vi "Autonomous Independent.vi"() -> ()   [LabVIEW 2017]
doc: "This VI is called when autonomous begins, and will automatically be terminated when autonomous ends. You can carry out timed or sensor driven robot movement independently without needing to return to the caller."
uses:
  <vilib>/Rock Robotics/WPI/Utilities/WPI_GetSetVariantRefNum.vi
  <vilib>/Rock Robotics/Network Tables/NT Read String.vi
  <vilib>/Rock Robotics/Network Tables/NT Write Numeric Array.vi
  Robot Global Data.vi
  <vilib>/Rock Robotics/WPI/Solenoid/Deprecated/WPI_SolenoidSetBool.vi
panel:
  in  "Right LLL":T1(array[cluster])=[{"Left Joystick"=0.975, "Right Joystick"=1.0, "Duration"=5.0, "SOL A"=TRUE, "SOL B"=FALSE, "Lift Up"=FALSE, "Lift Down"=FALSE, "Intake In"=FALSE, "Intake Out"=FALSE, "Left Distance"=10.0, "Right Distance"=10.0, "Drive?"=TRUE, "Wrist Up"=FALSE, "Wrist Down"=FALSE, "Lift Target"=0.0, "Wrist Target"=0.0}, {"Left Joystick"=0.0, "Right Joystick"=0.0, "Duration"=0.5, "SOL A"=TRUE, "SOL B"=FALSE, "Lift Up"=FALSE, "Lift Down"=FALSE, "Intake In"=FALSE, "Intake Out"=FALSE, "Left Distance"=0.0, "Right Distance"=0.0, "Drive?"=FALSE, "Wrist Up"=FALSE, "Wrist Down"=FALSE, "Lift Target"=0.0, "Wrist Target"=0.0}, {"Left Joystick"=0.975, "Right Joystick"=-1.0, "Duration"=5.0, "SOL A"=FALSE, "SOL B"=TRUE, "Lift Up"=FALSE, "Lift Down"=FALSE, "Intake In"=FALSE, "Intake Out"=FALSE, "Left Distance"=24.2, "Right Distance"=24.2, "Drive?"=TRUE, "Wrist Up"=FALSE, "Wrist Down"=FALSE, "Lift Target"=0.0, "Wrist Target"=0.0}, {"Left Joystick"=0.0, "Right Joystick"=0.0, "Duration"=0.5, "SOL A"=TRUE, "SOL B"=FALSE, "Lift Up"=FALSE, "Lift Down"=FALSE, "Intake In"=FALSE, "Intake Out"=FALSE, "Left Distance"=0.0, "Right Distance"=0.0, "Drive?"=FALSE, "Wrist Up"=FALSE, "Wrist Down"=FALSE, "Lift Target"=0.0, "Wrist Target"=0.0}, {"Left Joystick"=0.975, "Right Joystick"=1.0, "Duration"=5.0, "SOL A"=TRUE, "SOL B"=FALSE, "Lift Up"=FALSE, "Lift Down"=FALSE, "Intake In"=FALSE, "Intake Out"=FALSE, "Left Distance"=192.0, "Right Distance"=192.0, "Drive?"=TRUE, "Wrist Up"=FALSE, "Wrist Down"=FALSE, "Lift Target"=0.0, "Wrist Target"=0.0}, {"Left Joystick"=0.0, "Right Joystick"=0.0, "Duration"=0.5, "SOL A"=TRUE, "SOL B"=FALSE, "Lift Up"=FALSE, "Lift Down"=FALSE, "Intake In"=FALSE, "Intake Out"=FALSE, "Left Distance"=0.0, "Right Distance"=0.0, "Drive?"=FALSE, "Wrist Up"=FALSE, "Wrist Down"=FALSE, "Lift Target"=0.0, "Wrist Target"=0.0}, {"Left Joystick"=-0.975, "Right Joystick"=-1.0, "Duration"=5.0, "SOL A"=FALSE, "SOL B"=TRUE, "Lift Up"=FALSE, "Lift Down"=FALSE, "Intake In"=FALSE, "Intake Out"=FALSE, "Left Distance"=24.2, "Right Distance"=24.2, "Drive?"=TRUE, "Wrist Up"=FALSE, "Wrist Down"=FALSE, "Lift Target"=0.0, "Wrist Target"=0.0}, {"Left Joystick"=0.0, "Right Joystick"=0.0, "Duration"=0.5, "SOL A"=TRUE, "SOL B"=FALSE, "Lift Up"=FALSE, "Lift Down"=FALSE, "Intake In"=FALSE, "Intake Out"=FALSE, "Left Distance"=0.0, "Right Distance"=0.0, "Drive?"=FALSE, "Wrist Up"=FALSE, "Wrist Down"=FALSE, "Lift Target"=0.0, "Wrist Target"=0.0}, {"Left Joystick"=0.975, "Right Joystick"=1.0, "Duration"=5.0, "SOL A"=TRUE, "SOL B"=FALSE, "Lift Up"=FALSE, "Lift Down"=FALSE, "Intake In"=FALSE, "Intake Out"=FALSE, "Left Distance"=152.0, "Right Distance"=152.0, "Drive?"=TRUE, "Wrist Up"=FALSE, "Wrist Down"=FALSE, "Lift Target"=0.0, "Wrist Target"=0.0}, {"Left Joystick"=0.0, "Right Joystick"=0.0, "Duration"=0.5, "SOL A"=TRUE, "SOL B"=FALSE, "Lift Up"=FALSE, "Lift Down"=FALSE, "Intake In"=FALSE, "Intake Out"=FALSE, "Left Distance"=0.0, "Right Distance"=0.0, "Drive?"=FALSE, "Wrist Up"=FALSE, "Wrist Down"=FALSE, "Lift Target"=0.0, "Wrist Target"=0.0}, {"Left Joystick"=0.975, "Right Joystick"=-1.0, "Duration"=5.0, "SOL A"=FALSE, "SOL B"=TRUE, "Lift Up"=TRUE, "Lift Down"=FALSE, "Intake In"=FALSE, "Intake Out"=FALSE, "Left Distance"=12.1, "Right Distance"=12.1, "Drive?"=TRUE, "Wrist Up"=TRUE, "Wrist Down"=FALSE, "Lift Target"=15.0, "Wrist Target"=45.0}, {"Left Joystick"=0.0, "Right Joystick"=0.0, "Duration"=0.75, "SOL A"=TRUE, "SOL B"=FALSE, "Lift Up"=FALSE, "Lift Down"=FALSE, "Intake In"=FALSE, "Intake Out"=TRUE, "Left Distance"=0.0, "Right Distance"=0.0, "Drive?"=FALSE, "Wrist Up"=FALSE, "Wrist Down"=FALSE, "Lift Target"=0.0, "Wrist Target"=0.0}, {"Left Joystick"=0.0, "Right Joystick"=0.0, "Duration"=3.0, "SOL A"=TRUE, "SOL B"=FALSE, "Lift Up"=FALSE, "Lift Down"=FALSE, "Intake In"=FALSE, "Intake Out"=FALSE, "Left Distance"=25.0, "Right Distance"=25.0, "Drive?"=TRUE, "Wrist Up"=FALSE, "Wrist Down"=FALSE, "Lift Target"=0.0, "Wrist Target"=0.0}, {"Left Joystick"=0.0, "Right Joystick"=0.0, "Duration"=0.75, "SOL A"=TRUE, "SOL B"=FALSE, "Lift Up"=FALSE, "Lift Down"=FALSE, "Intake In"=TRUE, "Intake Out"=FALSE, "Left Distance"=0.0, "Right Distance"=0.0, "Drive?"=TRUE, "Wrist Up"=FALSE, "Wrist Down"=FALSE, "Lift Target"=0.0, "Wrist Target"=0.0}]
  in  "Right LRL":T1(array[cluster])=[{"Left Joystick"=0.975, "Right Joystick"=1.0, "Duration"=5.0, "SOL A"=TRUE, "SOL B"=FALSE, "Lift Up"=FALSE, "Lift Down"=FALSE, "Intake In"=FALSE, "Intake Out"=FALSE, "Left Distance"=10.0, "Right Distance"=10.0, "Drive?"=TRUE, "Wrist Up"=FALSE, "Wrist Down"=FALSE, "Lift Target"=0.0, "Wrist Target"=0.0}, {"Left Joystick"=0.0, "Right Joystick"=0.0, "Duration"=0.5, "SOL A"=TRUE, "SOL B"=FALSE, "Lift Up"=FALSE, "Lift Down"=FALSE, "Intake In"=FALSE, "Intake Out"=FALSE, "Left Distance"=0.0, "Right Distance"=0.0, "Drive?"=FALSE, "Wrist Up"=FALSE, "Wrist Down"=FALSE, "Lift Target"=0.0, "Wrist Target"=0.0}, {"Left Joystick"=0.975, "Right Joystick"=-1.0, "Duration"=5.0, "SOL A"=FALSE, "SOL B"=TRUE, "Lift Up"=FALSE, "Lift Down"=FALSE, "Intake In"=FALSE, "Intake Out"=FALSE, "Left Distance"=24.2, "Right Distance"=24.2, "Drive?"=TRUE, "Wrist Up"=FALSE, "Wrist Down"=FALSE, "Lift Target"=0.0, "Wrist Target"=0.0}, {"Left Joystick"=0.0, "Right Joystick"=0.0, "Duration"=0.5, "SOL A"=TRUE, "SOL B"=FALSE, "Lift Up"=FALSE, "Lift Down"=FALSE, "Intake In"=FALSE, "Intake Out"=FALSE, "Left Distance"=0.0, "Right Distance"=0.0, "Drive?"=FALSE, "Wrist Up"=FALSE, "Wrist Down"=FALSE, "Lift Target"=0.0, "Wrist Target"=0.0}, {"Left Joystick"=0.975, "Right Joystick"=1.0, "Duration"=5.0, "SOL A"=TRUE, "SOL B"=FALSE, "Lift Up"=FALSE, "Lift Down"=FALSE, "Intake In"=FALSE, "Intake Out"=FALSE, "Left Distance"=192.0, "Right Distance"=192.0, "Drive?"=TRUE, "Wrist Up"=FALSE, "Wrist Down"=FALSE, "Lift Target"=0.0, "Wrist Target"=0.0}, {"Left Joystick"=0.0, "Right Joystick"=0.0, "Duration"=0.5, "SOL A"=TRUE, "SOL B"=FALSE, "Lift Up"=FALSE, "Lift Down"=FALSE, "Intake In"=FALSE, "Intake Out"=FALSE, "Left Distance"=0.0, "Right Distance"=0.0, "Drive?"=FALSE, "Wrist Up"=FALSE, "Wrist Down"=FALSE, "Lift Target"=0.0, "Wrist Target"=0.0}, {"Left Joystick"=-0.975, "Right Joystick"=-1.0, "Duration"=5.0, "SOL A"=FALSE, "SOL B"=TRUE, "Lift Up"=FALSE, "Lift Down"=FALSE, "Intake In"=FALSE, "Intake Out"=FALSE, "Left Distance"=24.2, "Right Distance"=24.2, "Drive?"=TRUE, "Wrist Up"=FALSE, "Wrist Down"=FALSE, "Lift Target"=0.0, "Wrist Target"=0.0}, {"Left Joystick"=0.0, "Right Joystick"=0.0, "Duration"=0.5, "SOL A"=TRUE, "SOL B"=FALSE, "Lift Up"=FALSE, "Lift Down"=FALSE, "Intake In"=FALSE, "Intake Out"=FALSE, "Left Distance"=0.0, "Right Distance"=0.0, "Drive?"=FALSE, "Wrist Up"=FALSE, "Wrist Down"=FALSE, "Lift Target"=0.0, "Wrist Target"=0.0}, {"Left Joystick"=0.975, "Right Joystick"=1.0, "Duration"=5.0, "SOL A"=TRUE, "SOL B"=FALSE, "Lift Up"=FALSE, "Lift Down"=FALSE, "Intake In"=FALSE, "Intake Out"=FALSE, "Left Distance"=152.0, "Right Distance"=152.0, "Drive?"=TRUE, "Wrist Up"=FALSE, "Wrist Down"=FALSE, "Lift Target"=0.0, "Wrist Target"=0.0}, {"Left Joystick"=0.0, "Right Joystick"=0.0, "Duration"=0.5, "SOL A"=TRUE, "SOL B"=FALSE, "Lift Up"=FALSE, "Lift Down"=FALSE, "Intake In"=FALSE, "Intake Out"=FALSE, "Left Distance"=0.0, "Right Distance"=0.0, "Drive?"=FALSE, "Wrist Up"=FALSE, "Wrist Down"=FALSE, "Lift Target"=0.0, "Wrist Target"=0.0}, {"Left Joystick"=0.975, "Right Joystick"=-1.0, "Duration"=5.0, "SOL A"=FALSE, "SOL B"=TRUE, "Lift Up"=TRUE, "Lift Down"=FALSE, "Intake In"=FALSE, "Intake Out"=FALSE, "Left Distance"=12.1, "Right Distance"=12.1, "Drive?"=TRUE, "Wrist Up"=TRUE, "Wrist Down"=FALSE, "Lift Target"=15.0, "Wrist Target"=45.0}, {"Left Joystick"=0.0, "Right Joystick"=0.0, "Duration"=0.75, "SOL A"=TRUE, "SOL B"=FALSE, "Lift Up"=FALSE, "Lift Down"=FALSE, "Intake In"=FALSE, "Intake Out"=TRUE, "Left Distance"=0.0, "Right Distance"=0.0, "Drive?"=FALSE, "Wrist Up"=FALSE, "Wrist Down"=FALSE, "Lift Target"=0.0, "Wrist Target"=0.0}, {"Left Joystick"=0.0, "Right Joystick"=0.0, "Duration"=3.0, "SOL A"=TRUE, "SOL B"=FALSE, "Lift Up"=FALSE, "Lift Down"=FALSE, "Intake In"=FALSE, "Intake Out"=FALSE, "Left Distance"=25.0, "Right Distance"=25.0, "Drive?"=TRUE, "Wrist Up"=FALSE, "Wrist Down"=FALSE, "Lift Target"=0.0, "Wrist Target"=0.0}, {"Left Joystick"=0.0, "Right Joystick"=0.0, "Duration"=0.75, "SOL A"=TRUE, "SOL B"=FALSE, "Lift Up"=FALSE, "Lift Down"=FALSE, "Intake In"=TRUE, "Intake Out"=FALSE, "Left Distance"=0.0, "Right Distance"=0.0, "Drive?"=TRUE, "Wrist Up"=FALSE, "Wrist Down"=FALSE, "Lift Target"=0.0, "Wrist Target"=0.0}, {"Left Joystick"=0.0, "Right Joystick"=0.0, "Duration"=0.5, "SOL A"=TRUE, "SOL B"=FALSE, "Lift Up"=FALSE, "Lift Down"=FALSE, "Intake In"=FALSE, "Intake Out"=FALSE, "Left Distance"=0.0, "Right Distance"=0.0, "Drive?"=FALSE, "Wrist Up"=FALSE, "Wrist Down"=FALSE, "Lift Target"=0.0, "Wrist Target"=0.0}, {"Left Joystick"=0.975, "Right Joystick"=1.0, "Duration"=5.0, "SOL A"=TRUE, "SOL B"=FALSE, "Lift Up"=FALSE, "Lift Down"=FALSE, "Intake In"=FALSE, "Intake Out"=FALSE, "Left Distance"=12.0, "Right Distance"=12.0, "Drive?"=TRUE, "Wrist Up"=FALSE, "Wrist Down"=FALSE, "Lift Target"=0.0, "Wrist Target"=0.0}, {"Left Joystick"=0.0, "Right Joystick"=0.0, "Duration"=0.5, "SOL A"=TRUE, "SOL B"=FALSE, "Lift Up"=FALSE, "Lift Down"=FALSE, "Intake In"=FALSE, "Intake Out"=FALSE, "Left Distance"=0.0, "Right Distance"=0.0, "Drive?"=FALSE, "Wrist Up"=FALSE, "Wrist Down"=FALSE, "Lift Target"=0.0, "Wrist Target"=0.0}, {"Left Joystick"=0.975, "Right Joystick"=-1.0, "Duration"=5.0, "SOL A"=FALSE, "SOL B"=TRUE, "Lift Up"=FALSE, "Lift Down"=FALSE, "Intake In"=FALSE, "Intake Out"=FALSE, "Left Distance"=12.1, "Right Distance"=12.1, "Drive?"=TRUE, "Wrist Up"=FALSE, "Wrist Down"=FALSE, "Lift Target"=0.0, "Wrist Target"=0.0}, {"Left Joystick"=0.0, "Right Joystick"=0.0, "Duration"=0.5, "SOL A"=TRUE, "SOL B"=FALSE, "Lift Up"=FALSE, "Lift Down"=FALSE, "Intake In"=FALSE, "Intake Out"=FALSE, "Left Distance"=0.0, "Right Distance"=0.0, "Drive?"=FALSE, "Wrist Up"=FALSE, "Wrist Down"=FALSE, "Lift Target"=0.0, "Wrist Target"=0.0}, {"Left Joystick"=-0.975, "Right Joystick"=-1.0, "Duration"=5.0, "SOL A"=TRUE, "SOL B"=FALSE, "Lift Up"=FALSE, "Lift Down"=FALSE, "Intake In"=FALSE, "Intake Out"=FALSE, "Left Distance"=156.0, "Right Distance"=156.0, "Drive?"=TRUE, "Wrist Up"=FALSE, "Wrist Down"=FALSE, "Lift Target"=0.0, "Wrist Target"=0.0}, {"Left Joystick"=0.0, "Right Joystick"=0.0, "Duration"=0.5, "SOL A"=TRUE, "SOL B"=FALSE, "Lift Up"=FALSE, "Lift Down"=FALSE, "Intake In"=FALSE, "Intake Out"=FALSE, "Left Distance"=0.0, "Right Distance"=0.0, "Drive?"=FALSE, "Wrist Up"=FALSE, "Wrist Down"=FALSE, "Lift Target"=0.0, "Wrist Target"=0.0}, {"Left Joystick"=0.975, "Right Joystick"=-1.0, "Duration"=5.0, "SOL A"=FALSE, "SOL B"=TRUE, "Lift Up"=FALSE, "Lift Down"=FALSE, "Intake In"=FALSE, "Intake Out"=FALSE, "Left Distance"=24.2, "Right Distance"=24.2, "Drive?"=TRUE, "Wrist Up"=FALSE, "Wrist Down"=FALSE, "Lift Target"=0.0, "Wrist Target"=0.0}, {"Left Joystick"=0.0, "Right Joystick"=0.0, "Duration"=0.5, "SOL A"=TRUE, "SOL B"=FALSE, "Lift Up"=FALSE, "Lift Down"=FALSE, "Intake In"=FALSE, "Intake Out"=FALSE, "Left Distance"=0.0, "Right Distance"=0.0, "Drive?"=FALSE, "Wrist Up"=FALSE, "Wrist Down"=FALSE, "Lift Target"=0.0, "Wrist Target"=0.0}, {"Left Joystick"=-0.975, "Right Joystick"=-1.0, "Duration"=5.0, "SOL A"=TRUE, "SOL B"=FALSE, "Lift Up"=FALSE, "Lift Down"=FALSE, "Intake In"=FALSE, "Intake Out"=FALSE, "Left Distance"=48.0, "Right Distance"=48.0, "Drive?"=TRUE, "Wrist Up"=FALSE, "Wrist Down"=FALSE, "Lift Target"=0.0, "Wrist Target"=0.0}, {"Left Joystick"=0.0, "Right Joystick"=0.0, "Duration"=0.5, "SOL A"=TRUE, "SOL B"=FALSE, "Lift Up"=FALSE, "Lift Down"=FALSE, "Intake In"=FALSE, "Intake Out"=FALSE, "Left Distance"=0.0, "Right Distance"=0.0, "Drive?"=FALSE, "Wrist Up"=FALSE, "Wrist Down"=FALSE, "Lift Target"=0.0, "Wrist Target"=0.0}, {"Left Joystick"=0.975, "Right Joystick"=-1.0, "Duration"=5.0, "SOL A"=FALSE, "SOL B"=TRUE, "Lift Up"=TRUE, "Lift Down"=FALSE, "Intake In"=FALSE, "Intake Out"=FALSE, "Left Distance"=6.05, "Right Distance"=6.05, "Drive?"=TRUE, "Wrist Up"=TRUE, "Wrist Down"=FALSE, "Lift Target"=50.0, "Wrist Target"=45.0}, {"Left Joystick"=0.0, "Right Joystick"=0.0, "Duration"=0.75, "SOL A"=TRUE, "SOL B"=FALSE, "Lift Up"=FALSE, "Lift Down"=FALSE, "Intake In"=FALSE, "Intake Out"=TRUE, "Left Distance"=0.0, "Right Distance"=0.0, "Drive?"=FALSE, "Wrist Up"=FALSE, "Wrist Down"=FALSE, "Lift Target"=0.0, "Wrist Target"=0.0}]
  in  "Left RLR":T1(array[cluster])=[{"Left Joystick"=0.975, "Right Joystick"=1.0, "Duration"=5.0, "SOL A"=TRUE, "SOL B"=FALSE, "Lift Up"=FALSE, "Lift Down"=FALSE, "Intake In"=FALSE, "Intake Out"=FALSE, "Left Distance"=10.0, "Right Distance"=10.0, "Drive?"=TRUE, "Wrist Up"=FALSE, "Wrist Down"=FALSE, "Lift Target"=0.0, "Wrist Target"=0.0}, {"Left Joystick"=0.0, "Right Joystick"=0.0, "Duration"=0.5, "SOL A"=TRUE, "SOL B"=FALSE, "Lift Up"=FALSE, "Lift Down"=FALSE, "Intake In"=FALSE, "Intake Out"=FALSE, "Left Distance"=0.0, "Right Distance"=0.0, "Drive?"=FALSE, "Wrist Up"=FALSE, "Wrist Down"=FALSE, "Lift Target"=0.0, "Wrist Target"=0.0}, {"Left Joystick"=-0.975, "Right Joystick"=1.0, "Duration"=5.0, "SOL A"=FALSE, "SOL B"=TRUE, "Lift Up"=FALSE, "Lift Down"=FALSE, "Intake In"=FALSE, "Intake Out"=FALSE, "Left Distance"=24.2, "Right Distance"=24.2, "Drive?"=TRUE, "Wrist Up"=FALSE, "Wrist Down"=FALSE, "Lift Target"=0.0, "Wrist Target"=0.0}, {"Left Joystick"=0.0, "Right Joystick"=0.0, "Duration"=0.5, "SOL A"=TRUE, "SOL B"=FALSE, "Lift Up"=FALSE, "Lift Down"=FALSE, "Intake In"=FALSE, "Intake Out"=FALSE, "Left Distance"=0.0, "Right Distance"=0.0, "Drive?"=FALSE, "Wrist Up"=FALSE, "Wrist Down"=FALSE, "Lift Target"=0.0, "Wrist Target"=0.0}, {"Left Joystick"=0.975, "Right Joystick"=1.0, "Duration"=5.0, "SOL A"=TRUE, "SOL B"=FALSE, "Lift Up"=FALSE, "Lift Down"=FALSE, "Intake In"=FALSE, "Intake Out"=FALSE, "Left Distance"=192.0, "Right Distance"=192.0, "Drive?"=TRUE, "Wrist Up"=FALSE, "Wrist Down"=FALSE, "Lift Target"=0.0, "Wrist Target"=0.0}, {"Left Joystick"=0.0, "Right Joystick"=0.0, "Duration"=0.5, "SOL A"=TRUE, "SOL B"=FALSE, "Lift Up"=FALSE, "Lift Down"=FALSE, "Intake In"=FALSE, "Intake Out"=FALSE, "Left Distance"=0.0, "Right Distance"=0.0, "Drive?"=FALSE, "Wrist Up"=FALSE, "Wrist Down"=FALSE, "Lift Target"=0.0, "Wrist Target"=0.0}, {"Left Joystick"=0.975, "Right Joystick"=-1.0, "Duration"=5.0, "SOL A"=FALSE, "SOL B"=TRUE, "Lift Up"=FALSE, "Lift Down"=FALSE, "Intake In"=FALSE, "Intake Out"=FALSE, "Left Distance"=24.2, "Right Distance"=24.2, "Drive?"=TRUE, "Wrist Up"=FALSE, "Wrist Down"=FALSE, "Lift Target"=0.0, "Wrist Target"=0.0}, {"Left Joystick"=0.0, "Right Joystick"=0.0, "Duration"=0.5, "SOL A"=TRUE, "SOL B"=FALSE, "Lift Up"=FALSE, "Lift Down"=FALSE, "Intake In"=FALSE, "Intake Out"=FALSE, "Left Distance"=0.0, "Right Distance"=0.0, "Drive?"=FALSE, "Wrist Up"=FALSE, "Wrist Down"=FALSE, "Lift Target"=0.0, "Wrist Target"=0.0}, {"Left Joystick"=0.975, "Right Joystick"=1.0, "Duration"=5.0, "SOL A"=TRUE, "SOL B"=FALSE, "Lift Up"=FALSE, "Lift Down"=FALSE, "Intake In"=FALSE, "Intake Out"=FALSE, "Left Distance"=152.0, "Right Distance"=152.0, "Drive?"=TRUE, "Wrist Up"=FALSE, "Wrist Down"=FALSE, "Lift Target"=0.0, "Wrist Target"=0.0}, {"Left Joystick"=0.0, "Right Joystick"=0.0, "Duration"=0.5, "SOL A"=TRUE, "SOL B"=FALSE, "Lift Up"=FALSE, "Lift Down"=FALSE, "Intake In"=FALSE, "Intake Out"=FALSE, "Left Distance"=0.0, "Right Distance"=0.0, "Drive?"=FALSE, "Wrist Up"=FALSE, "Wrist Down"=FALSE, "Lift Target"=0.0, "Wrist Target"=0.0}, {"Left Joystick"=-0.975, "Right Joystick"=1.0, "Duration"=5.0, "SOL A"=FALSE, "SOL B"=TRUE, "Lift Up"=TRUE, "Lift Down"=FALSE, "Intake In"=FALSE, "Intake Out"=FALSE, "Left Distance"=12.1, "Right Distance"=12.1, "Drive?"=TRUE, "Wrist Up"=TRUE, "Wrist Down"=FALSE, "Lift Target"=15.0, "Wrist Target"=45.0}, {"Left Joystick"=0.0, "Right Joystick"=0.0, "Duration"=0.75, "SOL A"=TRUE, "SOL B"=FALSE, "Lift Up"=FALSE, "Lift Down"=FALSE, "Intake In"=FALSE, "Intake Out"=TRUE, "Left Distance"=0.0, "Right Distance"=0.0, "Drive?"=FALSE, "Wrist Up"=FALSE, "Wrist Down"=FALSE, "Lift Target"=0.0, "Wrist Target"=0.0}, {"Left Joystick"=0.0, "Right Joystick"=0.0, "Duration"=3.0, "SOL A"=TRUE, "SOL B"=FALSE, "Lift Up"=FALSE, "Lift Down"=FALSE, "Intake In"=FALSE, "Intake Out"=FALSE, "Left Distance"=25.0, "Right Distance"=25.0, "Drive?"=TRUE, "Wrist Up"=FALSE, "Wrist Down"=FALSE, "Lift Target"=0.0, "Wrist Target"=0.0}, {"Left Joystick"=0.0, "Right Joystick"=0.0, "Duration"=0.75, "SOL A"=TRUE, "SOL B"=FALSE, "Lift Up"=FALSE, "Lift Down"=FALSE, "Intake In"=TRUE, "Intake Out"=FALSE, "Left Distance"=0.0, "Right Distance"=0.0, "Drive?"=TRUE, "Wrist Up"=FALSE, "Wrist Down"=FALSE, "Lift Target"=0.0, "Wrist Target"=0.0}]
  in  "Left RRR":T1(array[cluster])=[{"Left Joystick"=0.975, "Right Joystick"=1.0, "Duration"=5.0, "SOL A"=TRUE, "SOL B"=FALSE, "Lift Up"=FALSE, "Lift Down"=FALSE, "Intake In"=FALSE, "Intake Out"=FALSE, "Left Distance"=10.0, "Right Distance"=10.0, "Drive?"=TRUE, "Wrist Up"=FALSE, "Wrist Down"=FALSE, "Lift Target"=0.0, "Wrist Target"=0.0}, {"Left Joystick"=0.0, "Right Joystick"=0.0, "Duration"=0.5, "SOL A"=TRUE, "SOL B"=FALSE, "Lift Up"=FALSE, "Lift Down"=FALSE, "Intake In"=FALSE, "Intake Out"=FALSE, "Left Distance"=0.0, "Right Distance"=0.0, "Drive?"=FALSE, "Wrist Up"=FALSE, "Wrist Down"=FALSE, "Lift Target"=0.0, "Wrist Target"=0.0}, {"Left Joystick"=-0.975, "Right Joystick"=1.0, "Duration"=5.0, "SOL A"=FALSE, "SOL B"=TRUE, "Lift Up"=FALSE, "Lift Down"=FALSE, "Intake In"=FALSE, "Intake Out"=FALSE, "Left Distance"=24.2, "Right Distance"=24.2, "Drive?"=TRUE, "Wrist Up"=FALSE, "Wrist Down"=FALSE, "Lift Target"=0.0, "Wrist Target"=0.0}, {"Left Joystick"=0.0, "Right Joystick"=0.0, "Duration"=0.5, "SOL A"=TRUE, "SOL B"=FALSE, "Lift Up"=FALSE, "Lift Down"=FALSE, "Intake In"=FALSE, "Intake Out"=FALSE, "Left Distance"=0.0, "Right Distance"=0.0, "Drive?"=FALSE, "Wrist Up"=FALSE, "Wrist Down"=FALSE, "Lift Target"=0.0, "Wrist Target"=0.0}, {"Left Joystick"=0.975, "Right Joystick"=1.0, "Duration"=5.0, "SOL A"=TRUE, "SOL B"=FALSE, "Lift Up"=FALSE, "Lift Down"=FALSE, "Intake In"=FALSE, "Intake Out"=FALSE, "Left Distance"=192.0, "Right Distance"=192.0, "Drive?"=TRUE, "Wrist Up"=FALSE, "Wrist Down"=FALSE, "Lift Target"=0.0, "Wrist Target"=0.0}, {"Left Joystick"=0.0, "Right Joystick"=0.0, "Duration"=0.5, "SOL A"=TRUE, "SOL B"=FALSE, "Lift Up"=FALSE, "Lift Down"=FALSE, "Intake In"=FALSE, "Intake Out"=FALSE, "Left Distance"=0.0, "Right Distance"=0.0, "Drive?"=FALSE, "Wrist Up"=FALSE, "Wrist Down"=FALSE, "Lift Target"=0.0, "Wrist Target"=0.0}, {"Left Joystick"=0.975, "Right Joystick"=-1.0, "Duration"=5.0, "SOL A"=FALSE, "SOL B"=TRUE, "Lift Up"=FALSE, "Lift Down"=FALSE, "Intake In"=FALSE, "Intake Out"=FALSE, "Left Distance"=24.2, "Right Distance"=24.2, "Drive?"=TRUE, "Wrist Up"=FALSE, "Wrist Down"=FALSE, "Lift Target"=0.0, "Wrist Target"=0.0}, {"Left Joystick"=0.0, "Right Joystick"=0.0, "Duration"=0.5, "SOL A"=TRUE, "SOL B"=FALSE, "Lift Up"=FALSE, "Lift Down"=FALSE, "Intake In"=FALSE, "Intake Out"=FALSE, "Left Distance"=0.0, "Right Distance"=0.0, "Drive?"=FALSE, "Wrist Up"=FALSE, "Wrist Down"=FALSE, "Lift Target"=0.0, "Wrist Target"=0.0}, {"Left Joystick"=0.975, "Right Joystick"=1.0, "Duration"=5.0, "SOL A"=TRUE, "SOL B"=FALSE, "Lift Up"=FALSE, "Lift Down"=FALSE, "Intake In"=FALSE, "Intake Out"=FALSE, "Left Distance"=152.0, "Right Distance"=152.0, "Drive?"=TRUE, "Wrist Up"=FALSE, "Wrist Down"=FALSE, "Lift Target"=0.0, "Wrist Target"=0.0}, {"Left Joystick"=0.0, "Right Joystick"=0.0, "Duration"=0.5, "SOL A"=TRUE, "SOL B"=FALSE, "Lift Up"=FALSE, "Lift Down"=FALSE, "Intake In"=FALSE, "Intake Out"=FALSE, "Left Distance"=0.0, "Right Distance"=0.0, "Drive?"=FALSE, "Wrist Up"=FALSE, "Wrist Down"=FALSE, "Lift Target"=0.0, "Wrist Target"=0.0}, {"Left Joystick"=-0.975, "Right Joystick"=1.0, "Duration"=5.0, "SOL A"=FALSE, "SOL B"=TRUE, "Lift Up"=TRUE, "Lift Down"=FALSE, "Intake In"=FALSE, "Intake Out"=FALSE, "Left Distance"=12.1, "Right Distance"=12.1, "Drive?"=TRUE, "Wrist Up"=TRUE, "Wrist Down"=FALSE, "Lift Target"=15.0, "Wrist Target"=45.0}, {"Left Joystick"=0.0, "Right Joystick"=0.0, "Duration"=0.75, "SOL A"=TRUE, "SOL B"=FALSE, "Lift Up"=FALSE, "Lift Down"=FALSE, "Intake In"=FALSE, "Intake Out"=TRUE, "Left Distance"=0.0, "Right Distance"=0.0, "Drive?"=FALSE, "Wrist Up"=FALSE, "Wrist Down"=FALSE, "Lift Target"=0.0, "Wrist Target"=0.0}, {"Left Joystick"=0.0, "Right Joystick"=0.0, "Duration"=3.0, "SOL A"=TRUE, "SOL B"=FALSE, "Lift Up"=FALSE, "Lift Down"=FALSE, "Intake In"=FALSE, "Intake Out"=FALSE, "Left Distance"=25.0, "Right Distance"=25.0, "Drive?"=TRUE, "Wrist Up"=FALSE, "Wrist Down"=FALSE, "Lift Target"=0.0, "Wrist Target"=0.0}, {"Left Joystick"=0.0, "Right Joystick"=0.0, "Duration"=0.75, "SOL A"=TRUE, "SOL B"=FALSE, "Lift Up"=FALSE, "Lift Down"=FALSE, "Intake In"=TRUE, "Intake Out"=FALSE, "Left Distance"=0.0, "Right Distance"=0.0, "Drive?"=TRUE, "Wrist Up"=FALSE, "Wrist Down"=FALSE, "Lift Target"=0.0, "Wrist Target"=0.0}]
  in  "Center LRL":T1(array[cluster])=[{"Left Joystick"=-0.975, "Right Joystick"=-1.0, "Duration"=5.0, "SOL A"=TRUE, "SOL B"=FALSE, "Lift Up"=FALSE, "Lift Down"=FALSE, "Intake In"=FALSE, "Intake Out"=FALSE, "Left Distance"=10.0, "Right Distance"=10.0, "Drive?"=TRUE, "Wrist Up"=FALSE, "Wrist Down"=FALSE, "Lift Target"=0.0, "Wrist Target"=0.0}, {"Left Joystick"=0.0, "Right Joystick"=0.0, "Duration"=0.5, "SOL A"=TRUE, "SOL B"=FALSE, "Lift Up"=FALSE, "Lift Down"=FALSE, "Intake In"=FALSE, "Intake Out"=FALSE, "Left Distance"=0.0, "Right Distance"=0.0, "Drive?"=FALSE, "Wrist Up"=FALSE, "Wrist Down"=FALSE, "Lift Target"=0.0, "Wrist Target"=0.0}, {"Left Joystick"=0.975, "Right Joystick"=-1.0, "Duration"=5.0, "SOL A"=FALSE, "SOL B"=TRUE, "Lift Up"=FALSE, "Lift Down"=FALSE, "Intake In"=FALSE, "Intake Out"=FALSE, "Left Distance"=24.2, "Right Distance"=24.2, "Drive?"=TRUE, "Wrist Up"=FALSE, "Wrist Down"=FALSE, "Lift Target"=0.0, "Wrist Target"=0.0}, {"Left Joystick"=0.0, "Right Joystick"=0.0, "Duration"=0.5, "SOL A"=TRUE, "SOL B"=FALSE, "Lift Up"=FALSE, "Lift Down"=FALSE, "Intake In"=FALSE, "Intake Out"=FALSE, "Left Distance"=0.0, "Right Distance"=0.0, "Drive?"=FALSE, "Wrist Up"=FALSE, "Wrist Down"=FALSE, "Lift Target"=0.0, "Wrist Target"=0.0}, {"Left Joystick"=-0.975, "Right Joystick"=-1.0, "Duration"=5.0, "SOL A"=TRUE, "SOL B"=FALSE, "Lift Up"=FALSE, "Lift Down"=FALSE, "Intake In"=FALSE, "Intake Out"=FALSE, "Left Distance"=84.0, "Right Distance"=84.0, "Drive?"=TRUE, "Wrist Up"=FALSE, "Wrist Down"=FALSE, "Lift Target"=0.0, "Wrist Target"=0.0}, {"Left Joystick"=0.0, "Right Joystick"=0.0, "Duration"=0.5, "SOL A"=TRUE, "SOL B"=FALSE, "Lift Up"=FALSE, "Lift Down"=FALSE, "Intake In"=FALSE, "Intake Out"=FALSE, "Left Distance"=0.0, "Right Distance"=0.0, "Drive?"=FALSE, "Wrist Up"=FALSE, "Wrist Down"=FALSE, "Lift Target"=0.0, "Wrist Target"=0.0}, {"Left Joystick"=-0.975, "Right Joystick"=1.0, "Duration"=5.0, "SOL A"=FALSE, "SOL B"=TRUE, "Lift Up"=FALSE, "Lift Down"=FALSE, "Intake In"=FALSE, "Intake Out"=FALSE, "Left Distance"=24.2, "Right Distance"=24.2, "Drive?"=TRUE, "Wrist Up"=FALSE, "Wrist Down"=FALSE, "Lift Target"=0.0, "Wrist Target"=0.0}, {"Left Joystick"=0.0, "Right Joystick"=0.0, "Duration"=0.5, "SOL A"=TRUE, "SOL B"=FALSE, "Lift Up"=FALSE, "Lift Down"=FALSE, "Intake In"=FALSE, "Intake Out"=FALSE, "Left Distance"=0.0, "Right Distance"=0.0, "Drive?"=FALSE, "Wrist Up"=FALSE, "Wrist Down"=FALSE, "Lift Target"=0.0, "Wrist Target"=0.0}, {"Left Joystick"=-0.975, "Right Joystick"=-1.0, "Duration"=5.0, "SOL A"=TRUE, "SOL B"=FALSE, "Lift Up"=FALSE, "Lift Down"=FALSE, "Intake In"=FALSE, "Intake Out"=FALSE, "Left Distance"=152.0, "Right Distance"=152.0, "Drive?"=TRUE, "Wrist Up"=FALSE, "Wrist Down"=FALSE, "Lift Target"=0.0, "Wrist Target"=0.0}, {"Left Joystick"=0.0, "Right Joystick"=0.0, "Duration"=0.5, "SOL A"=TRUE, "SOL B"=FALSE, "Lift Up"=FALSE, "Lift Down"=FALSE, "Intake In"=FALSE, "Intake Out"=FALSE, "Left Distance"=0.0, "Right Distance"=0.0, "Drive?"=FALSE, "Wrist Up"=FALSE, "Wrist Down"=FALSE, "Lift Target"=0.0, "Wrist Target"=0.0}, {"Left Joystick"=-0.975, "Right Joystick"=1.0, "Duration"=5.0, "SOL A"=FALSE, "SOL B"=TRUE, "Lift Up"=TRUE, "Lift Down"=FALSE, "Intake In"=FALSE, "Intake Out"=FALSE, "Left Distance"=36.3, "Right Distance"=36.3, "Drive?"=TRUE, "Wrist Up"=TRUE, "Wrist Down"=FALSE, "Lift Target"=15.0, "Wrist Target"=45.0}, {"Left Joystick"=0.0, "Right Joystick"=0.0, "Duration"=0.75, "SOL A"=TRUE, "SOL B"=FALSE, "Lift Up"=FALSE, "Lift Down"=FALSE, "Intake In"=FALSE, "Intake Out"=TRUE, "Left Distance"=0.0, "Right Distance"=0.0, "Drive?"=FALSE, "Wrist Up"=FALSE, "Wrist Down"=FALSE, "Lift Target"=0.0, "Wrist Target"=0.0}, {"Left Joystick"=0.0, "Right Joystick"=0.0, "Duration"=3.0, "SOL A"=TRUE, "SOL B"=FALSE, "Lift Up"=FALSE, "Lift Down"=FALSE, "Intake In"=FALSE, "Intake Out"=FALSE, "Left Distance"=25.0, "Right Distance"=25.0, "Drive?"=TRUE, "Wrist Up"=FALSE, "Wrist Down"=FALSE, "Lift Target"=0.0, "Wrist Target"=0.0}, {"Left Joystick"=0.0, "Right Joystick"=0.0, "Duration"=0.75, "SOL A"=TRUE, "SOL B"=FALSE, "Lift Up"=FALSE, "Lift Down"=FALSE, "Intake In"=TRUE, "Intake Out"=FALSE, "Left Distance"=0.0, "Right Distance"=0.0, "Drive?"=TRUE, "Wrist Up"=FALSE, "Wrist Down"=FALSE, "Lift Target"=0.0, "Wrist Target"=0.0}]
  in  "Right RRR":T1(array[cluster])=[{"Left Joystick"=0.975, "Right Joystick"=1.0, "Duration"=5.0, "SOL A"=TRUE, "SOL B"=FALSE, "Lift Up"=FALSE, "Lift Down"=FALSE, "Intake In"=FALSE, "Intake Out"=FALSE, "Left Distance"=199.6, "Right Distance"=199.6, "Drive?"=TRUE, "Wrist Up"=FALSE, "Wrist Down"=FALSE, "Lift Target"=0.0, "Wrist Target"=0.0}, {"Left Joystick"=0.0, "Right Joystick"=0.0, "Duration"=0.5, "SOL A"=TRUE, "SOL B"=FALSE, "Lift Up"=FALSE, "Lift Down"=FALSE, "Intake In"=FALSE, "Intake Out"=FALSE, "Left Distance"=0.0, "Right Distance"=0.0, "Drive?"=FALSE, "Wrist Up"=FALSE, "Wrist Down"=FALSE, "Lift Target"=0.0, "Wrist Target"=0.0}, {"Left Joystick"=-0.975, "Right Joystick"=1.0, "Duration"=5.0, "SOL A"=FALSE, "SOL B"=TRUE, "Lift Up"=FALSE, "Lift Down"=FALSE, "Intake In"=FALSE, "Intake Out"=FALSE, "Left Distance"=13.2, "Right Distance"=13.2, "Drive?"=TRUE, "Wrist Up"=FALSE, "Wrist Down"=FALSE, "Lift Target"=0.0, "Wrist Target"=0.0}, {"Left Joystick"=0.0, "Right Joystick"=0.0, "Duration"=0.5, "SOL A"=TRUE, "SOL B"=FALSE, "Lift Up"=FALSE, "Lift Down"=FALSE, "Intake In"=FALSE, "Intake Out"=FALSE, "Left Distance"=0.0, "Right Distance"=0.0, "Drive?"=FALSE, "Wrist Up"=FALSE, "Wrist Down"=FALSE, "Lift Target"=0.0, "Wrist Target"=0.0}, {"Left Joystick"=-0.975, "Right Joystick"=-1.0, "Duration"=5.0, "SOL A"=TRUE, "SOL B"=FALSE, "Lift Up"=TRUE, "Lift Down"=FALSE, "Intake In"=FALSE, "Intake Out"=FALSE, "Left Distance"=18.2, "Right Distance"=18.2, "Drive?"=TRUE, "Wrist Up"=TRUE, "Wrist Down"=FALSE, "Lift Target"=15.0, "Wrist Target"=45.0}, {"Left Joystick"=0.0, "Right Joystick"=0.0, "Duration"=0.75, "SOL A"=TRUE, "SOL B"=FALSE, "Lift Up"=FALSE, "Lift Down"=FALSE, "Intake In"=FALSE, "Intake Out"=TRUE, "Left Distance"=0.0, "Right Distance"=0.0, "Drive?"=FALSE, "Wrist Up"=FALSE, "Wrist Down"=FALSE, "Lift Target"=0.0, "Wrist Target"=0.0}, {"Left Joystick"=0.975, "Right Joystick"=1.0, "Duration"=5.0, "SOL A"=TRUE, "SOL B"=FALSE, "Lift Up"=FALSE, "Lift Down"=FALSE, "Intake In"=FALSE, "Intake Out"=FALSE, "Left Distance"=18.2, "Right Distance"=18.2, "Drive?"=TRUE, "Wrist Up"=FALSE, "Wrist Down"=FALSE, "Lift Target"=0.0, "Wrist Target"=0.0}, {"Left Joystick"=0.0, "Right Joystick"=0.0, "Duration"=0.5, "SOL A"=TRUE, "SOL B"=FALSE, "Lift Up"=FALSE, "Lift Down"=FALSE, "Intake In"=FALSE, "Intake Out"=FALSE, "Left Distance"=0.0, "Right Distance"=0.0, "Drive?"=FALSE, "Wrist Up"=FALSE, "Wrist Down"=FALSE, "Lift Target"=0.0, "Wrist Target"=0.0}, {"Left Joystick"=0.975, "Right Joystick"=-1.0, "Duration"=5.0, "SOL A"=FALSE, "SOL B"=TRUE, "Lift Up"=FALSE, "Lift Down"=FALSE, "Intake In"=FALSE, "Intake Out"=FALSE, "Left Distance"=27.0, "Right Distance"=27.0, "Drive?"=TRUE, "Wrist Up"=FALSE, "Wrist Down"=FALSE, "Lift Target"=0.0, "Wrist Target"=0.0}, {"Left Joystick"=0.0, "Right Joystick"=0.0, "Duration"=0.5, "SOL A"=TRUE, "SOL B"=FALSE, "Lift Up"=FALSE, "Lift Down"=FALSE, "Intake In"=FALSE, "Intake Out"=FALSE, "Left Distance"=0.0, "Right Distance"=0.0, "Drive?"=FALSE, "Wrist Up"=FALSE, "Wrist Down"=FALSE, "Lift Target"=0.0, "Wrist Target"=0.0}, {"Left Joystick"=0.975, "Right Joystick"=1.0, "Duration"=5.0, "SOL A"=TRUE, "SOL B"=FALSE, "Lift Up"=FALSE, "Lift Down"=FALSE, "Intake In"=FALSE, "Intake Out"=FALSE, "Left Distance"=19.7, "Right Distance"=19.7, "Drive?"=TRUE, "Wrist Up"=FALSE, "Wrist Down"=FALSE, "Lift Target"=0.0, "Wrist Target"=0.0}, {"Left Joystick"=0.0, "Right Joystick"=0.0, "Duration"=0.5, "SOL A"=TRUE, "SOL B"=FALSE, "Lift Up"=FALSE, "Lift Down"=FALSE, "Intake In"=FALSE, "Intake Out"=FALSE, "Left Distance"=0.0, "Right Distance"=0.0, "Drive?"=FALSE, "Wrist Up"=FALSE, "Wrist Down"=FALSE, "Lift Target"=0.0, "Wrist Target"=0.0}, {"Left Joystick"=-0.975, "Right Joystick"=1.0, "Duration"=5.0, "SOL A"=FALSE, "SOL B"=TRUE, "Lift Up"=FALSE, "Lift Down"=FALSE, "Intake In"=FALSE, "Intake Out"=FALSE, "Left Distance"=25.6, "Right Distance"=25.6, "Drive?"=TRUE, "Wrist Up"=FALSE, "Wrist Down"=FALSE, "Lift Target"=0.0, "Wrist Target"=0.0}, {"Left Joystick"=0.0, "Right Joystick"=0.0, "Duration"=0.5, "SOL A"=TRUE, "SOL B"=FALSE, "Lift Up"=FALSE, "Lift Down"=FALSE, "Intake In"=FALSE, "Intake Out"=FALSE, "Left Distance"=0.0, "Right Distance"=0.0, "Drive?"=FALSE, "Wrist Up"=FALSE, "Wrist Down"=FALSE, "Lift Target"=0.0, "Wrist Target"=0.0}, {"Left Joystick"=-0.975, "Right Joystick"=-1.0, "Duration"=5.0, "SOL A"=TRUE, "SOL B"=FALSE, "Lift Up"=FALSE, "Lift Down"=FALSE, "Intake In"=FALSE, "Intake Out"=FALSE, "Left Distance"=4.0, "Right Distance"=4.0, "Drive?"=TRUE, "Wrist Up"=FALSE, "Wrist Down"=FALSE, "Lift Target"=0.0, "Wrist Target"=0.0}, {"Left Joystick"=0.0, "Right Joystick"=0.0, "Duration"=0.75, "SOL A"=TRUE, "SOL B"=FALSE, "Lift Up"=FALSE, "Lift Down"=FALSE, "Intake In"=TRUE, "Intake Out"=FALSE, "Left Distance"=0.0, "Right Distance"=0.0, "Drive?"=FALSE, "Wrist Up"=FALSE, "Wrist Down"=FALSE, "Lift Target"=0.0, "Wrist Target"=0.0}, {"Left Joystick"=0.975, "Right Joystick"=1.0, "Duration"=5.0, "SOL A"=TRUE, "SOL B"=FALSE, "Lift Up"=FALSE, "Lift Down"=FALSE, "Intake In"=FALSE, "Intake Out"=FALSE, "Left Distance"=4.0, "Right Distance"=4.0, "Drive?"=TRUE, "Wrist Up"=FALSE, "Wrist Down"=FALSE, "Lift Target"=0.0, "Wrist Target"=0.0}, {"Left Joystick"=0.0, "Right Joystick"=0.0, "Duration"=0.5, "SOL A"=TRUE, "SOL B"=FALSE, "Lift Up"=FALSE, "Lift Down"=FALSE, "Intake In"=FALSE, "Intake Out"=FALSE, "Left Distance"=0.0, "Right Distance"=0.0, "Drive?"=FALSE, "Wrist Up"=FALSE, "Wrist Down"=FALSE, "Lift Target"=0.0, "Wrist Target"=0.0}, {"Left Joystick"=-0.975, "Right Joystick"=-1.0, "Duration"=5.0, "SOL A"=TRUE, "SOL B"=FALSE, "Lift Up"=FALSE, "Lift Down"=FALSE, "Intake In"=FALSE, "Intake Out"=FALSE, "Left Distance"=30.1, "Right Distance"=30.1, "Drive?"=TRUE, "Wrist Up"=FALSE, "Wrist Down"=FALSE, "Lift Target"=0.0, "Wrist Target"=0.0}, {"Left Joystick"=0.0, "Right Joystick"=0.0, "Duration"=0.5, "SOL A"=TRUE, "SOL B"=FALSE, "Lift Up"=FALSE, "Lift Down"=FALSE, "Intake In"=FALSE, "Intake Out"=FALSE, "Left Distance"=0.0, "Right Distance"=0.0, "Drive?"=FALSE, "Wrist Up"=FALSE, "Wrist Down"=FALSE, "Lift Target"=0.0, "Wrist Target"=0.0}, {"Left Joystick"=-0.975, "Right Joystick"=-1.0, "Duration"=5.0, "SOL A"=TRUE, "SOL B"=FALSE, "Lift Up"=TRUE, "Lift Down"=FALSE, "Intake In"=FALSE, "Intake Out"=FALSE, "Left Distance"=25.0, "Right Distance"=25.0, "Drive?"=TRUE, "Wrist Up"=TRUE, "Wrist Down"=FALSE, "Lift Target"=50.0, "Wrist Target"=45.0}, {"Left Joystick"=0.0, "Right Joystick"=0.0, "Duration"=0.75, "SOL A"=TRUE, "SOL B"=FALSE, "Lift Up"=FALSE, "Lift Down"=FALSE, "Intake In"=FALSE, "Intake Out"=TRUE, "Left Distance"=0.0, "Right Distance"=0.0, "Drive?"=FALSE, "Wrist Up"=FALSE, "Wrist Down"=FALSE, "Lift Target"=0.0, "Wrist Target"=0.0}]
  in  "Right RLR":T1(array[cluster])=[{"Left Joystick"=0.975, "Right Joystick"=1.0, "Duration"=5.0, "SOL A"=TRUE, "SOL B"=FALSE, "Lift Up"=FALSE, "Lift Down"=FALSE, "Intake In"=FALSE, "Intake Out"=FALSE, "Left Distance"=199.6, "Right Distance"=199.6, "Drive?"=TRUE, "Wrist Up"=FALSE, "Wrist Down"=FALSE, "Lift Target"=0.0, "Wrist Target"=0.0}, {"Left Joystick"=0.0, "Right Joystick"=0.0, "Duration"=0.5, "SOL A"=TRUE, "SOL B"=FALSE, "Lift Up"=FALSE, "Lift Down"=FALSE, "Intake In"=FALSE, "Intake Out"=FALSE, "Left Distance"=0.0, "Right Distance"=0.0, "Drive?"=FALSE, "Wrist Up"=FALSE, "Wrist Down"=FALSE, "Lift Target"=0.0, "Wrist Target"=0.0}, {"Left Joystick"=-0.975, "Right Joystick"=1.0, "Duration"=5.0, "SOL A"=FALSE, "SOL B"=TRUE, "Lift Up"=FALSE, "Lift Down"=FALSE, "Intake In"=FALSE, "Intake Out"=FALSE, "Left Distance"=13.2, "Right Distance"=13.2, "Drive?"=TRUE, "Wrist Up"=FALSE, "Wrist Down"=FALSE, "Lift Target"=0.0, "Wrist Target"=0.0}, {"Left Joystick"=0.0, "Right Joystick"=0.0, "Duration"=0.5, "SOL A"=TRUE, "SOL B"=FALSE, "Lift Up"=FALSE, "Lift Down"=FALSE, "Intake In"=FALSE, "Intake Out"=FALSE, "Left Distance"=0.0, "Right Distance"=0.0, "Drive?"=FALSE, "Wrist Up"=FALSE, "Wrist Down"=FALSE, "Lift Target"=0.0, "Wrist Target"=0.0}, {"Left Joystick"=-0.975, "Right Joystick"=-1.0, "Duration"=5.0, "SOL A"=TRUE, "SOL B"=FALSE, "Lift Up"=TRUE, "Lift Down"=FALSE, "Intake In"=FALSE, "Intake Out"=FALSE, "Left Distance"=18.2, "Right Distance"=18.2, "Drive?"=TRUE, "Wrist Up"=TRUE, "Wrist Down"=FALSE, "Lift Target"=15.0, "Wrist Target"=45.0}, {"Left Joystick"=0.0, "Right Joystick"=0.0, "Duration"=0.75, "SOL A"=TRUE, "SOL B"=FALSE, "Lift Up"=FALSE, "Lift Down"=FALSE, "Intake In"=FALSE, "Intake Out"=TRUE, "Left Distance"=0.0, "Right Distance"=0.0, "Drive?"=FALSE, "Wrist Up"=FALSE, "Wrist Down"=FALSE, "Lift Target"=0.0, "Wrist Target"=0.0}, {"Left Joystick"=0.975, "Right Joystick"=1.0, "Duration"=5.0, "SOL A"=FALSE, "SOL B"=TRUE, "Lift Up"=FALSE, "Lift Down"=FALSE, "Intake In"=FALSE, "Intake Out"=FALSE, "Left Distance"=18.2, "Right Distance"=18.2, "Drive?"=TRUE, "Wrist Up"=FALSE, "Wrist Down"=FALSE, "Lift Target"=0.0, "Wrist Target"=0.0}, {"Left Joystick"=0.0, "Right Joystick"=0.0, "Duration"=0.5, "SOL A"=TRUE, "SOL B"=FALSE, "Lift Up"=FALSE, "Lift Down"=FALSE, "Intake In"=FALSE, "Intake Out"=FALSE, "Left Distance"=0.0, "Right Distance"=0.0, "Drive?"=FALSE, "Wrist Up"=FALSE, "Wrist Down"=FALSE, "Lift Target"=0.0, "Wrist Target"=0.0}, {"Left Joystick"=0.975, "Right Joystick"=-1.0, "Duration"=5.0, "SOL A"=FALSE, "SOL B"=TRUE, "Lift Up"=FALSE, "Lift Down"=FALSE, "Intake In"=FALSE, "Intake Out"=FALSE, "Left Distance"=27.0, "Right Distance"=27.0, "Drive?"=TRUE, "Wrist Up"=FALSE, "Wrist Down"=FALSE, "Lift Target"=0.0, "Wrist Target"=0.0}, {"Left Joystick"=0.0, "Right Joystick"=0.0, "Duration"=0.5, "SOL A"=TRUE, "SOL B"=FALSE, "Lift Up"=FALSE, "Lift Down"=FALSE, "Intake In"=FALSE, "Intake Out"=FALSE, "Left Distance"=0.0, "Right Distance"=0.0, "Drive?"=FALSE, "Wrist Up"=FALSE, "Wrist Down"=FALSE, "Lift Target"=0.0, "Wrist Target"=0.0}, {"Left Joystick"=0.975, "Right Joystick"=1.0, "Duration"=5.0, "SOL A"=TRUE, "SOL B"=FALSE, "Lift Up"=FALSE, "Lift Down"=FALSE, "Intake In"=FALSE, "Intake Out"=FALSE, "Left Distance"=19.7, "Right Distance"=19.7, "Drive?"=TRUE, "Wrist Up"=FALSE, "Wrist Down"=FALSE, "Lift Target"=0.0, "Wrist Target"=0.0}, {"Left Joystick"=0.0, "Right Joystick"=0.0, "Duration"=0.5, "SOL A"=TRUE, "SOL B"=FALSE, "Lift Up"=FALSE, "Lift Down"=FALSE, "Intake In"=FALSE, "Intake Out"=FALSE, "Left Distance"=0.0, "Right Distance"=0.0, "Drive?"=FALSE, "Wrist Up"=FALSE, "Wrist Down"=FALSE, "Lift Target"=0.0, "Wrist Target"=0.0}, {"Left Joystick"=-0.975, "Right Joystick"=1.0, "Duration"=5.0, "SOL A"=FALSE, "SOL B"=TRUE, "Lift Up"=FALSE, "Lift Down"=FALSE, "Intake In"=FALSE, "Intake Out"=FALSE, "Left Distance"=25.6, "Right Distance"=25.6, "Drive?"=TRUE, "Wrist Up"=FALSE, "Wrist Down"=FALSE, "Lift Target"=0.0, "Wrist Target"=0.0}, {"Left Joystick"=0.0, "Right Joystick"=0.0, "Duration"=0.5, "SOL A"=TRUE, "SOL B"=FALSE, "Lift Up"=FALSE, "Lift Down"=FALSE, "Intake In"=FALSE, "Intake Out"=FALSE, "Left Distance"=0.0, "Right Distance"=0.0, "Drive?"=FALSE, "Wrist Up"=FALSE, "Wrist Down"=FALSE, "Lift Target"=0.0, "Wrist Target"=0.0}, {"Left Joystick"=-0.975, "Right Joystick"=-1.0, "Duration"=5.0, "SOL A"=TRUE, "SOL B"=FALSE, "Lift Up"=FALSE, "Lift Down"=FALSE, "Intake In"=FALSE, "Intake Out"=FALSE, "Left Distance"=4.0, "Right Distance"=4.0, "Drive?"=TRUE, "Wrist Up"=FALSE, "Wrist Down"=FALSE, "Lift Target"=0.0, "Wrist Target"=0.0}, {"Left Joystick"=0.0, "Right Joystick"=0.0, "Duration"=0.75, "SOL A"=TRUE, "SOL B"=FALSE, "Lift Up"=FALSE, "Lift Down"=FALSE, "Intake In"=TRUE, "Intake Out"=FALSE, "Left Distance"=0.0, "Right Distance"=0.0, "Drive?"=FALSE, "Wrist Up"=FALSE, "Wrist Down"=FALSE, "Lift Target"=0.0, "Wrist Target"=0.0}]
  in  "Center RRR":T1(array[cluster])=[{"Left Joystick"=-0.975, "Right Joystick"=-1.0, "Duration"=5.0, "SOL A"=TRUE, "SOL B"=FALSE, "Lift Up"=FALSE, "Lift Down"=FALSE, "Intake In"=FALSE, "Intake Out"=FALSE, "Left Distance"=12.0, "Right Distance"=12.0, "Drive?"=TRUE, "Wrist Up"=FALSE, "Wrist Down"=FALSE, "Lift Target"=0.0, "Wrist Target"=0.0}, {"Left Joystick"=0.0, "Right Joystick"=0.0, "Duration"=0.5, "SOL A"=TRUE, "SOL B"=FALSE, "Lift Up"=FALSE, "Lift Down"=FALSE, "Intake In"=FALSE, "Intake Out"=FALSE, "Left Distance"=0.0, "Right Distance"=0.0, "Drive?"=FALSE, "Wrist Up"=FALSE, "Wrist Down"=FALSE, "Lift Target"=0.0, "Wrist Target"=0.0}, {"Left Joystick"=-0.975, "Right Joystick"=1.0, "Duration"=5.0, "SOL A"=FALSE, "SOL B"=TRUE, "Lift Up"=FALSE, "Lift Down"=FALSE, "Intake In"=FALSE, "Intake Out"=FALSE, "Left Distance"=4.4, "Right Distance"=4.4, "Drive?"=TRUE, "Wrist Up"=FALSE, "Wrist Down"=FALSE, "Lift Target"=0.0, "Wrist Target"=0.0}, {"Left Joystick"=0.0, "Right Joystick"=0.0, "Duration"=0.5, "SOL A"=TRUE, "SOL B"=FALSE, "Lift Up"=FALSE, "Lift Down"=FALSE, "Intake In"=FALSE, "Intake Out"=FALSE, "Left Distance"=0.0, "Right Distance"=0.0, "Drive?"=FALSE, "Wrist Up"=FALSE, "Wrist Down"=FALSE, "Lift Target"=0.0, "Wrist Target"=0.0}, {"Left Joystick"=-0.975, "Right Joystick"=-1.0, "Duration"=5.0, "SOL A"=TRUE, "SOL B"=FALSE, "Lift Up"=FALSE, "Lift Down"=FALSE, "Intake In"=FALSE, "Intake Out"=FALSE, "Left Distance"=80.0, "Right Distance"=80.0, "Drive?"=TRUE, "Wrist Up"=FALSE, "Wrist Down"=FALSE, "Lift Target"=0.0, "Wrist Target"=0.0}, {"Left Joystick"=0.0, "Right Joystick"=0.0, "Duration"=3.0, "SOL A"=TRUE, "SOL B"=FALSE, "Lift Up"=TRUE, "Lift Down"=FALSE, "Intake In"=FALSE, "Intake Out"=FALSE, "Left Distance"=0.0, "Right Distance"=0.0, "Drive?"=TRUE, "Wrist Up"=TRUE, "Wrist Down"=FALSE, "Lift Target"=15.0, "Wrist Target"=45.0}, {"Left Joystick"=0.0, "Right Joystick"=0.0, "Duration"=0.5, "SOL A"=FALSE, "SOL B"=FALSE, "Lift Up"=FALSE, "Lift Down"=FALSE, "Intake In"=FALSE, "Intake Out"=TRUE, "Left Distance"=0.0, "Right Distance"=0.0, "Drive?"=FALSE, "Wrist Up"=FALSE, "Wrist Down"=FALSE, "Lift Target"=0.0, "Wrist Target"=0.0}, {"Left Joystick"=0.975, "Right Joystick"=1.0, "Duration"=5.0, "SOL A"=TRUE, "SOL B"=FALSE, "Lift Up"=FALSE, "Lift Down"=FALSE, "Intake In"=FALSE, "Intake Out"=FALSE, "Left Distance"=46.0, "Right Distance"=46.0, "Drive?"=TRUE, "Wrist Up"=FALSE, "Wrist Down"=FALSE, "Lift Target"=0.0, "Wrist Target"=0.0}, {"Left Joystick"=0.0, "Right Joystick"=0.0, "Duration"=0.5, "SOL A"=TRUE, "SOL B"=FALSE, "Lift Up"=FALSE, "Lift Down"=FALSE, "Intake In"=FALSE, "Intake Out"=FALSE, "Left Distance"=0.0, "Right Distance"=0.0, "Drive?"=FALSE, "Wrist Up"=FALSE, "Wrist Down"=FALSE, "Lift Target"=0.0, "Wrist Target"=0.0}, {"Left Joystick"=0.975, "Right Joystick"=-1.0, "Duration"=5.0, "SOL A"=FALSE, "SOL B"=TRUE, "Lift Up"=FALSE, "Lift Down"=FALSE, "Intake In"=FALSE, "Intake Out"=FALSE, "Left Distance"=7.7, "Right Distance"=7.7, "Drive?"=TRUE, "Wrist Up"=FALSE, "Wrist Down"=FALSE, "Lift Target"=0.0, "Wrist Target"=0.0}, {"Left Joystick"=0.0, "Right Joystick"=0.0, "Duration"=0.5, "SOL A"=TRUE, "SOL B"=FALSE, "Lift Up"=FALSE, "Lift Down"=FALSE, "Intake In"=FALSE, "Intake Out"=FALSE, "Left Distance"=0.0, "Right Distance"=0.0, "Drive?"=FALSE, "Wrist Up"=FALSE, "Wrist Down"=FALSE, "Lift Target"=0.0, "Wrist Target"=0.0}, {"Left Joystick"=-0.975, "Right Joystick"=-1.0, "Duration"=5.0, "SOL A"=TRUE, "SOL B"=FALSE, "Lift Up"=FALSE, "Lift Down"=FALSE, "Intake In"=FALSE, "Intake Out"=FALSE, "Left Distance"=10.0, "Right Distance"=10.0, "Drive?"=TRUE, "Wrist Up"=FALSE, "Wrist Down"=FALSE, "Lift Target"=0.0, "Wrist Target"=0.0}, {"Left Joystick"=0.0, "Right Joystick"=0.0, "Duration"=0.75, "SOL A"=TRUE, "SOL B"=FALSE, "Lift Up"=FALSE, "Lift Down"=FALSE, "Intake In"=TRUE, "Intake Out"=FALSE, "Left Distance"=0.0, "Right Distance"=0.0, "Drive?"=TRUE, "Wrist Up"=FALSE, "Wrist Down"=FALSE, "Lift Target"=0.0, "Wrist Target"=0.0}, {"Left Joystick"=0.0, "Right Joystick"=0.0, "Duration"=0.5, "SOL A"=TRUE, "SOL B"=FALSE, "Lift Up"=FALSE, "Lift Down"=FALSE, "Intake In"=FALSE, "Intake Out"=FALSE, "Left Distance"=0.0, "Right Distance"=0.0, "Drive?"=FALSE, "Wrist Up"=FALSE, "Wrist Down"=FALSE, "Lift Target"=0.0, "Wrist Target"=0.0}, {"Left Joystick"=0.975, "Right Joystick"=1.0, "Duration"=5.0, "SOL A"=TRUE, "SOL B"=FALSE, "Lift Up"=FALSE, "Lift Down"=FALSE, "Intake In"=FALSE, "Intake Out"=FALSE, "Left Distance"=10.0, "Right Distance"=10.0, "Drive?"=TRUE, "Wrist Up"=FALSE, "Wrist Down"=FALSE, "Lift Target"=0.0, "Wrist Target"=0.0}, {"Left Joystick"=0.0, "Right Joystick"=0.0, "Duration"=0.5, "SOL A"=TRUE, "SOL B"=FALSE, "Lift Up"=FALSE, "Lift Down"=FALSE, "Intake In"=FALSE, "Intake Out"=FALSE, "Left Distance"=0.0, "Right Distance"=0.0, "Drive?"=FALSE, "Wrist Up"=FALSE, "Wrist Down"=FALSE, "Lift Target"=0.0, "Wrist Target"=0.0}, {"Left Joystick"=-0.975, "Right Joystick"=1.0, "Duration"=5.0, "SOL A"=FALSE, "SOL B"=TRUE, "Lift Up"=FALSE, "Lift Down"=FALSE, "Intake In"=FALSE, "Intake Out"=FALSE, "Left Distance"=7.7, "Right Distance"=7.7, "Drive?"=TRUE, "Wrist Up"=FALSE, "Wrist Down"=FALSE, "Lift Target"=0.0, "Wrist Target"=0.0}, {"Left Joystick"=0.0, "Right Joystick"=0.0, "Duration"=0.5, "SOL A"=TRUE, "SOL B"=FALSE, "Lift Up"=FALSE, "Lift Down"=FALSE, "Intake In"=FALSE, "Intake Out"=FALSE, "Left Distance"=0.0, "Right Distance"=0.0, "Drive?"=FALSE, "Wrist Up"=FALSE, "Wrist Down"=FALSE, "Lift Target"=0.0, "Wrist Target"=0.0}, {"Left Joystick"=-0.975, "Right Joystick"=-1.0, "Duration"=5.0, "SOL A"=TRUE, "SOL B"=FALSE, "Lift Up"=FALSE, "Lift Down"=FALSE, "Intake In"=FALSE, "Intake Out"=FALSE, "Left Distance"=46.0, "Right Distance"=46.0, "Drive?"=TRUE, "Wrist Up"=FALSE, "Wrist Down"=FALSE, "Lift Target"=0.0, "Wrist Target"=0.0}, {"Left Joystick"=0.0, "Right Joystick"=0.0, "Duration"=0.5, "SOL A"=TRUE, "SOL B"=FALSE, "Lift Up"=FALSE, "Lift Down"=FALSE, "Intake In"=FALSE, "Intake Out"=FALSE, "Left Distance"=0.0, "Right Distance"=0.0, "Drive?"=FALSE, "Wrist Up"=FALSE, "Wrist Down"=FALSE, "Lift Target"=0.0, "Wrist Target"=0.0}, {"Left Joystick"=0.0, "Right Joystick"=0.0, "Duration"=5.0, "SOL A"=TRUE, "SOL B"=FALSE, "Lift Up"=TRUE, "Lift Down"=FALSE, "Intake In"=FALSE, "Intake Out"=FALSE, "Left Distance"=0.0, "Right Distance"=0.0, "Drive?"=TRUE, "Wrist Up"=TRUE, "Wrist Down"=FALSE, "Lift Target"=15.0, "Wrist Target"=45.0}, {"Left Joystick"=0.0, "Right Joystick"=0.0, "Duration"=0.75, "SOL A"=TRUE, "SOL B"=FALSE, "Lift Up"=FALSE, "Lift Down"=FALSE, "Intake In"=FALSE, "Intake Out"=TRUE, "Left Distance"=0.0, "Right Distance"=0.0, "Drive?"=FALSE, "Wrist Up"=FALSE, "Wrist Down"=FALSE, "Lift Target"=0.0, "Wrist Target"=0.0}, {"Left Joystick"=0.975, "Right Joystick"=1.0, "Duration"=5.0, "SOL A"=TRUE, "SOL B"=FALSE, "Lift Up"=FALSE, "Lift Down"=FALSE, "Intake In"=FALSE, "Intake Out"=FALSE, "Left Distance"=31.0, "Right Distance"=31.0, "Drive?"=TRUE, "Wrist Up"=FALSE, "Wrist Down"=FALSE, "Lift Target"=0.0, "Wrist Target"=0.0}, {"Left Joystick"=0.0, "Right Joystick"=0.0, "Duration"=0.5, "SOL A"=TRUE, "SOL B"=FALSE, "Lift Up"=FALSE, "Lift Down"=FALSE, "Intake In"=FALSE, "Intake Out"=FALSE, "Left Distance"=0.0, "Right Distance"=0.0, "Drive?"=FALSE, "Wrist Up"=FALSE, "Wrist Down"=FALSE, "Lift Target"=0.0, "Wrist Target"=0.0}, {"Left Joystick"=0.975, "Right Joystick"=-1.0, "Duration"=5.0, "SOL A"=TRUE, "SOL B"=FALSE, "Lift Up"=FALSE, "Lift Down"=FALSE, "Intake In"=FALSE, "Intake Out"=FALSE, "Left Distance"=9.6, "Right Distance"=9.6, "Drive?"=TRUE, "Wrist Up"=FALSE, "Wrist Down"=FALSE, "Lift Target"=0.0, "Wrist Target"=0.0}, {"Left Joystick"=0.0, "Right Joystick"=0.0, "Duration"=0.5, "SOL A"=TRUE, "SOL B"=FALSE, "Lift Up"=FALSE, "Lift Down"=FALSE, "Intake In"=FALSE, "Intake Out"=FALSE, "Left Distance"=0.0, "Right Distance"=0.0, "Drive?"=FALSE, "Wrist Up"=FALSE, "Wrist Down"=FALSE, "Lift Target"=0.0, "Wrist Target"=0.0}, {"Left Joystick"=-0.975, "Right Joystick"=-1.0, "Duration"=5.0, "SOL A"=TRUE, "SOL B"=FALSE, "Lift Up"=FALSE, "Lift Down"=FALSE, "Intake In"=FALSE, "Intake Out"=FALSE, "Left Distance"=10.0, "Right Distance"=10.0, "Drive?"=TRUE, "Wrist Up"=FALSE, "Wrist Down"=FALSE, "Lift Target"=0.0, "Wrist Target"=0.0}, {"Left Joystick"=0.0, "Right Joystick"=0.0, "Duration"=0.75, "SOL A"=TRUE, "SOL B"=FALSE, "Lift Up"=FALSE, "Lift Down"=FALSE, "Intake In"=TRUE, "Intake Out"=FALSE, "Left Distance"=0.0, "Right Distance"=0.0, "Drive?"=TRUE, "Wrist Up"=FALSE, "Wrist Down"=FALSE, "Lift Target"=0.0, "Wrist Target"=0.0}, {"Left Joystick"=0.0, "Right Joystick"=0.0, "Duration"=0.5, "SOL A"=TRUE, "SOL B"=FALSE, "Lift Up"=FALSE, "Lift Down"=FALSE, "Intake In"=FALSE, "Intake Out"=FALSE, "Left Distance"=0.0, "Right Distance"=0.0, "Drive?"=FALSE, "Wrist Up"=FALSE, "Wrist Down"=FALSE, "Lift Target"=0.0, "Wrist Target"=0.0}, {"Left Joystick"=0.975, "Right Joystick"=1.0, "Duration"=5.0, "SOL A"=TRUE, "SOL B"=FALSE, "Lift Up"=FALSE, "Lift Down"=FALSE, "Intake In"=FALSE, "Intake Out"=FALSE, "Left Distance"=10.0, "Right Distance"=10.0, "Drive?"=TRUE, "Wrist Up"=FALSE, "Wrist Down"=FALSE, "Lift Target"=0.0, "Wrist Target"=0.0}, {"Left Joystick"=0.0, "Right Joystick"=0.0, "Duration"=0.5, "SOL A"=TRUE, "SOL B"=FALSE, "Lift Up"=FALSE, "Lift Down"=FALSE, "Intake In"=FALSE, "Intake Out"=FALSE, "Left Distance"=0.0, "Right Distance"=0.0, "Drive?"=FALSE, "Wrist Up"=FALSE, "Wrist Down"=FALSE, "Lift Target"=0.0, "Wrist Target"=0.0}, {"Left Joystick"=-0.975, "Right Joystick"=1.0, "Duration"=5.0, "SOL A"=TRUE, "SOL B"=FALSE, "Lift Up"=FALSE, "Lift Down"=FALSE, "Intake In"=FALSE, "Intake Out"=FALSE, "Left Distance"=9.6, "Right Distance"=9.6, "Drive?"=TRUE, "Wrist Up"=FALSE, "Wrist Down"=FALSE, "Lift Target"=0.0, "Wrist Target"=0.0}, {"Left Joystick"=0.0, "Right Joystick"=0.0, "Duration"=0.5, "SOL A"=TRUE, "SOL B"=FALSE, "Lift Up"=FALSE, "Lift Down"=FALSE, "Intake In"=FALSE, "Intake Out"=FALSE, "Left Distance"=0.0, "Right Distance"=0.0, "Drive?"=FALSE, "Wrist Up"=FALSE, "Wrist Down"=FALSE, "Lift Target"=0.0, "Wrist Target"=0.0}, {"Left Joystick"=0.975, "Right Joystick"=1.0, "Duration"=5.0, "SOL A"=TRUE, "SOL B"=FALSE, "Lift Up"=FALSE, "Lift Down"=FALSE, "Intake In"=FALSE, "Intake Out"=FALSE, "Left Distance"=31.0, "Right Distance"=31.0, "Drive?"=TRUE, "Wrist Up"=FALSE, "Wrist Down"=FALSE, "Lift Target"=0.0, "Wrist Target"=0.0}, {"Left Joystick"=0.0, "Right Joystick"=0.0, "Duration"=5.0, "SOL A"=TRUE, "SOL B"=FALSE, "Lift Up"=TRUE, "Lift Down"=FALSE, "Intake In"=FALSE, "Intake Out"=FALSE, "Left Distance"=0.0, "Right Distance"=0.0, "Drive?"=TRUE, "Wrist Up"=TRUE, "Wrist Down"=FALSE, "Lift Target"=15.0, "Wrist Target"=45.0}, {"Left Joystick"=0.0, "Right Joystick"=0.0, "Duration"=0.75, "SOL A"=TRUE, "SOL B"=FALSE, "Lift Up"=FALSE, "Lift Down"=FALSE, "Intake In"=FALSE, "Intake Out"=TRUE, "Left Distance"=0.0, "Right Distance"=0.0, "Drive?"=FALSE, "Wrist Up"=FALSE, "Wrist Down"=FALSE, "Lift Target"=0.0, "Wrist Target"=0.0}]
  in  "Center LLL":T1(array[cluster])=[{"Left Joystick"=-0.975, "Right Joystick"=-1.0, "Duration"=5.0, "SOL A"=TRUE, "SOL B"=FALSE, "Lift Up"=FALSE, "Lift Down"=FALSE, "Intake In"=FALSE, "Intake Out"=FALSE, "Left Distance"=10.0, "Right Distance"=10.0, "Drive?"=TRUE, "Wrist Up"=FALSE, "Wrist Down"=FALSE, "Lift Target"=0.0, "Wrist Target"=0.0}, {"Left Joystick"=0.0, "Right Joystick"=0.0, "Duration"=0.5, "SOL A"=TRUE, "SOL B"=FALSE, "Lift Up"=FALSE, "Lift Down"=FALSE, "Intake In"=FALSE, "Intake Out"=FALSE, "Left Distance"=0.0, "Right Distance"=0.0, "Drive?"=FALSE, "Wrist Up"=FALSE, "Wrist Down"=FALSE, "Lift Target"=0.0, "Wrist Target"=0.0}, {"Left Joystick"=0.975, "Right Joystick"=-1.0, "Duration"=5.0, "SOL A"=FALSE, "SOL B"=TRUE, "Lift Up"=FALSE, "Lift Down"=FALSE, "Intake In"=FALSE, "Intake Out"=FALSE, "Left Distance"=24.2, "Right Distance"=24.2, "Drive?"=TRUE, "Wrist Up"=FALSE, "Wrist Down"=FALSE, "Lift Target"=0.0, "Wrist Target"=0.0}, {"Left Joystick"=0.0, "Right Joystick"=0.0, "Duration"=0.5, "SOL A"=TRUE, "SOL B"=FALSE, "Lift Up"=FALSE, "Lift Down"=FALSE, "Intake In"=FALSE, "Intake Out"=FALSE, "Left Distance"=0.0, "Right Distance"=0.0, "Drive?"=FALSE, "Wrist Up"=FALSE, "Wrist Down"=FALSE, "Lift Target"=0.0, "Wrist Target"=0.0}, {"Left Joystick"=-0.975, "Right Joystick"=-1.0, "Duration"=5.0, "SOL A"=TRUE, "SOL B"=FALSE, "Lift Up"=FALSE, "Lift Down"=FALSE, "Intake In"=FALSE, "Intake Out"=FALSE, "Left Distance"=84.0, "Right Distance"=84.0, "Drive?"=TRUE, "Wrist Up"=FALSE, "Wrist Down"=FALSE, "Lift Target"=0.0, "Wrist Target"=0.0}, {"Left Joystick"=0.0, "Right Joystick"=0.0, "Duration"=0.5, "SOL A"=TRUE, "SOL B"=FALSE, "Lift Up"=FALSE, "Lift Down"=FALSE, "Intake In"=FALSE, "Intake Out"=FALSE, "Left Distance"=0.0, "Right Distance"=0.0, "Drive?"=FALSE, "Wrist Up"=FALSE, "Wrist Down"=FALSE, "Lift Target"=0.0, "Wrist Target"=0.0}, {"Left Joystick"=-0.975, "Right Joystick"=1.0, "Duration"=5.0, "SOL A"=FALSE, "SOL B"=TRUE, "Lift Up"=FALSE, "Lift Down"=FALSE, "Intake In"=FALSE, "Intake Out"=FALSE, "Left Distance"=24.2, "Right Distance"=24.2, "Drive?"=TRUE, "Wrist Up"=FALSE, "Wrist Down"=FALSE, "Lift Target"=0.0, "Wrist Target"=0.0}, {"Left Joystick"=0.0, "Right Joystick"=0.0, "Duration"=0.5, "SOL A"=TRUE, "SOL B"=FALSE, "Lift Up"=FALSE, "Lift Down"=FALSE, "Intake In"=FALSE, "Intake Out"=FALSE, "Left Distance"=0.0, "Right Distance"=0.0, "Drive?"=FALSE, "Wrist Up"=FALSE, "Wrist Down"=FALSE, "Lift Target"=0.0, "Wrist Target"=0.0}, {"Left Joystick"=-0.975, "Right Joystick"=-1.0, "Duration"=5.0, "SOL A"=TRUE, "SOL B"=FALSE, "Lift Up"=FALSE, "Lift Down"=FALSE, "Intake In"=FALSE, "Intake Out"=FALSE, "Left Distance"=152.0, "Right Distance"=152.0, "Drive?"=TRUE, "Wrist Up"=FALSE, "Wrist Down"=FALSE, "Lift Target"=0.0, "Wrist Target"=0.0}, {"Left Joystick"=0.0, "Right Joystick"=0.0, "Duration"=0.5, "SOL A"=TRUE, "SOL B"=FALSE, "Lift Up"=FALSE, "Lift Down"=FALSE, "Intake In"=FALSE, "Intake Out"=FALSE, "Left Distance"=0.0, "Right Distance"=0.0, "Drive?"=FALSE, "Wrist Up"=FALSE, "Wrist Down"=FALSE, "Lift Target"=0.0, "Wrist Target"=0.0}, {"Left Joystick"=-0.975, "Right Joystick"=1.0, "Duration"=5.0, "SOL A"=FALSE, "SOL B"=TRUE, "Lift Up"=TRUE, "Lift Down"=FALSE, "Intake In"=FALSE, "Intake Out"=FALSE, "Left Distance"=36.3, "Right Distance"=36.3, "Drive?"=TRUE, "Wrist Up"=TRUE, "Wrist Down"=FALSE, "Lift Target"=15.0, "Wrist Target"=45.0}, {"Left Joystick"=0.0, "Right Joystick"=0.0, "Duration"=0.75, "SOL A"=TRUE, "SOL B"=FALSE, "Lift Up"=FALSE, "Lift Down"=FALSE, "Intake In"=FALSE, "Intake Out"=TRUE, "Left Distance"=0.0, "Right Distance"=0.0, "Drive?"=FALSE, "Wrist Up"=FALSE, "Wrist Down"=FALSE, "Lift Target"=0.0, "Wrist Target"=0.0}, {"Left Joystick"=0.0, "Right Joystick"=0.0, "Duration"=3.0, "SOL A"=TRUE, "SOL B"=FALSE, "Lift Up"=FALSE, "Lift Down"=FALSE, "Intake In"=FALSE, "Intake Out"=FALSE, "Left Distance"=25.0, "Right Distance"=25.0, "Drive?"=TRUE, "Wrist Up"=FALSE, "Wrist Down"=FALSE, "Lift Target"=0.0, "Wrist Target"=0.0}, {"Left Joystick"=0.0, "Right Joystick"=0.0, "Duration"=0.75, "SOL A"=TRUE, "SOL B"=FALSE, "Lift Up"=FALSE, "Lift Down"=FALSE, "Intake In"=TRUE, "Intake Out"=FALSE, "Left Distance"=0.0, "Right Distance"=0.0, "Drive?"=TRUE, "Wrist Up"=FALSE, "Wrist Down"=FALSE, "Lift Target"=0.0, "Wrist Target"=0.0}]
  in  "Center RLR":T1(array[cluster])=[{"Left Joystick"=-0.975, "Right Joystick"=-1.0, "Duration"=5.0, "SOL A"=TRUE, "SOL B"=FALSE, "Lift Up"=FALSE, "Lift Down"=FALSE, "Intake In"=FALSE, "Intake Out"=FALSE, "Left Distance"=12.0, "Right Distance"=12.0, "Drive?"=TRUE, "Wrist Up"=FALSE, "Wrist Down"=FALSE, "Lift Target"=0.0, "Wrist Target"=0.0}, {"Left Joystick"=0.0, "Right Joystick"=0.0, "Duration"=0.5, "SOL A"=TRUE, "SOL B"=FALSE, "Lift Up"=FALSE, "Lift Down"=FALSE, "Intake In"=FALSE, "Intake Out"=FALSE, "Left Distance"=0.0, "Right Distance"=0.0, "Drive?"=FALSE, "Wrist Up"=FALSE, "Wrist Down"=FALSE, "Lift Target"=0.0, "Wrist Target"=0.0}, {"Left Joystick"=-0.975, "Right Joystick"=1.0, "Duration"=5.0, "SOL A"=FALSE, "SOL B"=TRUE, "Lift Up"=FALSE, "Lift Down"=FALSE, "Intake In"=FALSE, "Intake Out"=FALSE, "Left Distance"=4.4, "Right Distance"=4.4, "Drive?"=TRUE, "Wrist Up"=FALSE, "Wrist Down"=FALSE, "Lift Target"=0.0, "Wrist Target"=0.0}, {"Left Joystick"=0.0, "Right Joystick"=0.0, "Duration"=0.5, "SOL A"=TRUE, "SOL B"=FALSE, "Lift Up"=FALSE, "Lift Down"=FALSE, "Intake In"=FALSE, "Intake Out"=FALSE, "Left Distance"=0.0, "Right Distance"=0.0, "Drive?"=FALSE, "Wrist Up"=FALSE, "Wrist Down"=FALSE, "Lift Target"=0.0, "Wrist Target"=0.0}, {"Left Joystick"=-0.975, "Right Joystick"=-1.0, "Duration"=5.0, "SOL A"=TRUE, "SOL B"=FALSE, "Lift Up"=FALSE, "Lift Down"=FALSE, "Intake In"=FALSE, "Intake Out"=FALSE, "Left Distance"=80.0, "Right Distance"=80.0, "Drive?"=TRUE, "Wrist Up"=FALSE, "Wrist Down"=FALSE, "Lift Target"=0.0, "Wrist Target"=0.0}, {"Left Joystick"=0.0, "Right Joystick"=0.0, "Duration"=2.0, "SOL A"=TRUE, "SOL B"=FALSE, "Lift Up"=TRUE, "Lift Down"=FALSE, "Intake In"=FALSE, "Intake Out"=FALSE, "Left Distance"=0.0, "Right Distance"=0.0, "Drive?"=TRUE, "Wrist Up"=TRUE, "Wrist Down"=FALSE, "Lift Target"=15.0, "Wrist Target"=45.0}, {"Left Joystick"=0.0, "Right Joystick"=0.0, "Duration"=0.75, "SOL A"=TRUE, "SOL B"=FALSE, "Lift Up"=FALSE, "Lift Down"=FALSE, "Intake In"=FALSE, "Intake Out"=TRUE, "Left Distance"=0.0, "Right Distance"=0.0, "Drive?"=FALSE, "Wrist Up"=FALSE, "Wrist Down"=FALSE, "Lift Target"=0.0, "Wrist Target"=0.0}, {"Left Joystick"=0.975, "Right Joystick"=1.0, "Duration"=5.0, "SOL A"=TRUE, "SOL B"=FALSE, "Lift Up"=FALSE, "Lift Down"=FALSE, "Intake In"=FALSE, "Intake Out"=FALSE, "Left Distance"=46.0, "Right Distance"=46.0, "Drive?"=TRUE, "Wrist Up"=FALSE, "Wrist Down"=FALSE, "Lift Target"=0.0, "Wrist Target"=0.0}, {"Left Joystick"=0.0, "Right Joystick"=0.0, "Duration"=0.5, "SOL A"=TRUE, "SOL B"=FALSE, "Lift Up"=FALSE, "Lift Down"=FALSE, "Intake In"=FALSE, "Intake Out"=FALSE, "Left Distance"=0.0, "Right Distance"=0.0, "Drive?"=FALSE, "Wrist Up"=FALSE, "Wrist Down"=FALSE, "Lift Target"=0.0, "Wrist Target"=0.0}, {"Left Joystick"=0.975, "Right Joystick"=-1.0, "Duration"=5.0, "SOL A"=FALSE, "SOL B"=TRUE, "Lift Up"=FALSE, "Lift Down"=FALSE, "Intake In"=FALSE, "Intake Out"=FALSE, "Left Distance"=7.7, "Right Distance"=7.7, "Drive?"=TRUE, "Wrist Up"=FALSE, "Wrist Down"=FALSE, "Lift Target"=0.0, "Wrist Target"=0.0}, {"Left Joystick"=0.0, "Right Joystick"=0.0, "Duration"=0.5, "SOL A"=TRUE, "SOL B"=FALSE, "Lift Up"=FALSE, "Lift Down"=FALSE, "Intake In"=FALSE, "Intake Out"=FALSE, "Left Distance"=0.0, "Right Distance"=0.0, "Drive?"=FALSE, "Wrist Up"=FALSE, "Wrist Down"=FALSE, "Lift Target"=0.0, "Wrist Target"=0.0}, {"Left Joystick"=-0.975, "Right Joystick"=-1.0, "Duration"=5.0, "SOL A"=TRUE, "SOL B"=FALSE, "Lift Up"=FALSE, "Lift Down"=FALSE, "Intake In"=FALSE, "Intake Out"=FALSE, "Left Distance"=10.0, "Right Distance"=10.0, "Drive?"=TRUE, "Wrist Up"=FALSE, "Wrist Down"=FALSE, "Lift Target"=0.0, "Wrist Target"=0.0}, {"Left Joystick"=0.0, "Right Joystick"=0.0, "Duration"=0.75, "SOL A"=TRUE, "SOL B"=FALSE, "Lift Up"=FALSE, "Lift Down"=FALSE, "Intake In"=TRUE, "Intake Out"=FALSE, "Left Distance"=0.0, "Right Distance"=0.0, "Drive?"=TRUE, "Wrist Up"=FALSE, "Wrist Down"=FALSE, "Lift Target"=0.0, "Wrist Target"=0.0}, {"Left Joystick"=0.0, "Right Joystick"=0.0, "Duration"=0.5, "SOL A"=TRUE, "SOL B"=FALSE, "Lift Up"=FALSE, "Lift Down"=FALSE, "Intake In"=FALSE, "Intake Out"=FALSE, "Left Distance"=0.0, "Right Distance"=0.0, "Drive?"=FALSE, "Wrist Up"=FALSE, "Wrist Down"=FALSE, "Lift Target"=0.0, "Wrist Target"=0.0}, {"Left Joystick"=0.975, "Right Joystick"=1.0, "Duration"=5.0, "SOL A"=TRUE, "SOL B"=FALSE, "Lift Up"=FALSE, "Lift Down"=FALSE, "Intake In"=FALSE, "Intake Out"=FALSE, "Left Distance"=10.0, "Right Distance"=10.0, "Drive?"=TRUE, "Wrist Up"=FALSE, "Wrist Down"=FALSE, "Lift Target"=0.0, "Wrist Target"=0.0}, {"Left Joystick"=0.0, "Right Joystick"=0.0, "Duration"=0.5, "SOL A"=TRUE, "SOL B"=FALSE, "Lift Up"=FALSE, "Lift Down"=FALSE, "Intake In"=FALSE, "Intake Out"=FALSE, "Left Distance"=0.0, "Right Distance"=0.0, "Drive?"=FALSE, "Wrist Up"=FALSE, "Wrist Down"=FALSE, "Lift Target"=0.0, "Wrist Target"=0.0}, {"Left Joystick"=-0.975, "Right Joystick"=1.0, "Duration"=5.0, "SOL A"=FALSE, "SOL B"=TRUE, "Lift Up"=FALSE, "Lift Down"=FALSE, "Intake In"=FALSE, "Intake Out"=FALSE, "Left Distance"=7.7, "Right Distance"=7.7, "Drive?"=TRUE, "Wrist Up"=FALSE, "Wrist Down"=FALSE, "Lift Target"=0.0, "Wrist Target"=0.0}, {"Left Joystick"=0.0, "Right Joystick"=0.0, "Duration"=0.5, "SOL A"=TRUE, "SOL B"=FALSE, "Lift Up"=FALSE, "Lift Down"=FALSE, "Intake In"=FALSE, "Intake Out"=FALSE, "Left Distance"=0.0, "Right Distance"=0.0, "Drive?"=FALSE, "Wrist Up"=FALSE, "Wrist Down"=FALSE, "Lift Target"=0.0, "Wrist Target"=0.0}, {"Left Joystick"=-0.975, "Right Joystick"=-1.0, "Duration"=5.0, "SOL A"=TRUE, "SOL B"=FALSE, "Lift Up"=FALSE, "Lift Down"=FALSE, "Intake In"=FALSE, "Intake Out"=FALSE, "Left Distance"=46.0, "Right Distance"=46.0, "Drive?"=TRUE, "Wrist Up"=FALSE, "Wrist Down"=FALSE, "Lift Target"=0.0, "Wrist Target"=0.0}, {"Left Joystick"=0.0, "Right Joystick"=0.0, "Duration"=0.5, "SOL A"=TRUE, "SOL B"=FALSE, "Lift Up"=FALSE, "Lift Down"=FALSE, "Intake In"=FALSE, "Intake Out"=FALSE, "Left Distance"=0.0, "Right Distance"=0.0, "Drive?"=FALSE, "Wrist Up"=FALSE, "Wrist Down"=FALSE, "Lift Target"=0.0, "Wrist Target"=0.0}, {"Left Joystick"=0.0, "Right Joystick"=0.0, "Duration"=5.0, "SOL A"=TRUE, "SOL B"=FALSE, "Lift Up"=TRUE, "Lift Down"=FALSE, "Intake In"=FALSE, "Intake Out"=FALSE, "Left Distance"=0.0, "Right Distance"=0.0, "Drive?"=TRUE, "Wrist Up"=TRUE, "Wrist Down"=FALSE, "Lift Target"=15.0, "Wrist Target"=45.0}, {"Left Joystick"=0.0, "Right Joystick"=0.0, "Duration"=0.5, "SOL A"=TRUE, "SOL B"=FALSE, "Lift Up"=FALSE, "Lift Down"=FALSE, "Intake In"=FALSE, "Intake Out"=TRUE, "Left Distance"=0.0, "Right Distance"=0.0, "Drive?"=FALSE, "Wrist Up"=FALSE, "Wrist Down"=FALSE, "Lift Target"=0.0, "Wrist Target"=0.0}, {"Left Joystick"=0.975, "Right Joystick"=1.0, "Duration"=5.0, "SOL A"=TRUE, "SOL B"=FALSE, "Lift Up"=FALSE, "Lift Down"=FALSE, "Intake In"=FALSE, "Intake Out"=FALSE, "Left Distance"=31.0, "Right Distance"=31.0, "Drive?"=TRUE, "Wrist Up"=FALSE, "Wrist Down"=FALSE, "Lift Target"=0.0, "Wrist Target"=0.0}, {"Left Joystick"=0.0, "Right Joystick"=0.0, "Duration"=0.5, "SOL A"=TRUE, "SOL B"=FALSE, "Lift Up"=FALSE, "Lift Down"=FALSE, "Intake In"=FALSE, "Intake Out"=FALSE, "Left Distance"=0.0, "Right Distance"=0.0, "Drive?"=FALSE, "Wrist Up"=FALSE, "Wrist Down"=FALSE, "Lift Target"=0.0, "Wrist Target"=0.0}, {"Left Joystick"=0.975, "Right Joystick"=-1.0, "Duration"=5.0, "SOL A"=FALSE, "SOL B"=TRUE, "Lift Up"=FALSE, "Lift Down"=FALSE, "Intake In"=FALSE, "Intake Out"=FALSE, "Left Distance"=9.6, "Right Distance"=9.6, "Drive?"=TRUE, "Wrist Up"=FALSE, "Wrist Down"=FALSE, "Lift Target"=0.0, "Wrist Target"=0.0}, {"Left Joystick"=0.0, "Right Joystick"=0.0, "Duration"=0.5, "SOL A"=TRUE, "SOL B"=FALSE, "Lift Up"=FALSE, "Lift Down"=FALSE, "Intake In"=FALSE, "Intake Out"=FALSE, "Left Distance"=0.0, "Right Distance"=0.0, "Drive?"=FALSE, "Wrist Up"=FALSE, "Wrist Down"=FALSE, "Lift Target"=0.0, "Wrist Target"=0.0}, {"Left Joystick"=-0.975, "Right Joystick"=-1.0, "Duration"=5.0, "SOL A"=TRUE, "SOL B"=FALSE, "Lift Up"=FALSE, "Lift Down"=FALSE, "Intake In"=FALSE, "Intake Out"=FALSE, "Left Distance"=10.0, "Right Distance"=10.0, "Drive?"=TRUE, "Wrist Up"=FALSE, "Wrist Down"=FALSE, "Lift Target"=0.0, "Wrist Target"=0.0}, {"Left Joystick"=0.0, "Right Joystick"=0.0, "Duration"=0.75, "SOL A"=TRUE, "SOL B"=FALSE, "Lift Up"=FALSE, "Lift Down"=FALSE, "Intake In"=TRUE, "Intake Out"=FALSE, "Left Distance"=0.0, "Right Distance"=0.0, "Drive?"=TRUE, "Wrist Up"=FALSE, "Wrist Down"=FALSE, "Lift Target"=0.0, "Wrist Target"=0.0}, {"Left Joystick"=0.0, "Right Joystick"=0.0, "Duration"=0.5, "SOL A"=TRUE, "SOL B"=FALSE, "Lift Up"=FALSE, "Lift Down"=FALSE, "Intake In"=FALSE, "Intake Out"=FALSE, "Left Distance"=0.0, "Right Distance"=0.0, "Drive?"=FALSE, "Wrist Up"=FALSE, "Wrist Down"=FALSE, "Lift Target"=0.0, "Wrist Target"=0.0}, {"Left Joystick"=0.975, "Right Joystick"=1.0, "Duration"=5.0, "SOL A"=TRUE, "SOL B"=FALSE, "Lift Up"=FALSE, "Lift Down"=FALSE, "Intake In"=FALSE, "Intake Out"=FALSE, "Left Distance"=10.0, "Right Distance"=10.0, "Drive?"=TRUE, "Wrist Up"=FALSE, "Wrist Down"=FALSE, "Lift Target"=0.0, "Wrist Target"=0.0}, {"Left Joystick"=0.0, "Right Joystick"=0.0, "Duration"=0.5, "SOL A"=TRUE, "SOL B"=FALSE, "Lift Up"=FALSE, "Lift Down"=FALSE, "Intake In"=FALSE, "Intake Out"=FALSE, "Left Distance"=0.0, "Right Distance"=0.0, "Drive?"=FALSE, "Wrist Up"=FALSE, "Wrist Down"=FALSE, "Lift Target"=0.0, "Wrist Target"=0.0}, {"Left Joystick"=-0.975, "Right Joystick"=1.0, "Duration"=5.0, "SOL A"=FALSE, "SOL B"=TRUE, "Lift Up"=FALSE, "Lift Down"=FALSE, "Intake In"=FALSE, "Intake Out"=FALSE, "Left Distance"=0.0, "Right Distance"=0.0, "Drive?"=TRUE, "Wrist Up"=FALSE, "Wrist Down"=FALSE, "Lift Target"=0.0, "Wrist Target"=0.0}, {"Left Joystick"=0.0, "Right Joystick"=0.0, "Duration"=0.5, "SOL A"=TRUE, "SOL B"=FALSE, "Lift Up"=FALSE, "Lift Down"=FALSE, "Intake In"=FALSE, "Intake Out"=FALSE, "Left Distance"=0.0, "Right Distance"=0.0, "Drive?"=FALSE, "Wrist Up"=FALSE, "Wrist Down"=FALSE, "Lift Target"=0.0, "Wrist Target"=0.0}, {"Left Joystick"=-0.975, "Right Joystick"=-1.0, "Duration"=5.0, "SOL A"=TRUE, "SOL B"=FALSE, "Lift Up"=FALSE, "Lift Down"=FALSE, "Intake In"=FALSE, "Intake Out"=FALSE, "Left Distance"=31.0, "Right Distance"=31.0, "Drive?"=TRUE, "Wrist Up"=FALSE, "Wrist Down"=FALSE, "Lift Target"=0.0, "Wrist Target"=0.0}, {"Left Joystick"=0.0, "Right Joystick"=0.0, "Duration"=5.0, "SOL A"=TRUE, "SOL B"=FALSE, "Lift Up"=TRUE, "Lift Down"=FALSE, "Intake In"=FALSE, "Intake Out"=FALSE, "Left Distance"=0.0, "Right Distance"=0.0, "Drive?"=TRUE, "Wrist Up"=TRUE, "Wrist Down"=FALSE, "Lift Target"=15.0, "Wrist Target"=45.0}, {"Left Joystick"=0.0, "Right Joystick"=0.0, "Duration"=0.75, "SOL A"=TRUE, "SOL B"=FALSE, "Lift Up"=FALSE, "Lift Down"=FALSE, "Intake In"=TRUE, "Intake Out"=FALSE, "Left Distance"=0.0, "Right Distance"=0.0, "Drive?"=FALSE, "Wrist Up"=FALSE, "Wrist Down"=FALSE, "Lift Target"=0.0, "Wrist Target"=0.0}]
  in  "Left LLL":T1(array[cluster])=[{"Left Joystick"=0.975, "Right Joystick"=1.0, "Duration"=5.0, "SOL A"=TRUE, "SOL B"=FALSE, "Lift Up"=FALSE, "Lift Down"=FALSE, "Intake In"=FALSE, "Intake Out"=FALSE, "Left Distance"=199.6, "Right Distance"=199.6, "Drive?"=TRUE, "Wrist Up"=FALSE, "Wrist Down"=FALSE, "Lift Target"=0.0, "Wrist Target"=0.0}, {"Left Joystick"=0.0, "Right Joystick"=0.0, "Duration"=0.5, "SOL A"=TRUE, "SOL B"=FALSE, "Lift Up"=FALSE, "Lift Down"=FALSE, "Intake In"=FALSE, "Intake Out"=FALSE, "Left Distance"=0.0, "Right Distance"=0.0, "Drive?"=FALSE, "Wrist Up"=FALSE, "Wrist Down"=FALSE, "Lift Target"=0.0, "Wrist Target"=0.0}, {"Left Joystick"=0.975, "Right Joystick"=-1.0, "Duration"=5.0, "SOL A"=FALSE, "SOL B"=TRUE, "Lift Up"=FALSE, "Lift Down"=FALSE, "Intake In"=FALSE, "Intake Out"=FALSE, "Left Distance"=13.2, "Right Distance"=13.2, "Drive?"=TRUE, "Wrist Up"=FALSE, "Wrist Down"=FALSE, "Lift Target"=0.0, "Wrist Target"=0.0}, {"Left Joystick"=0.0, "Right Joystick"=0.0, "Duration"=0.5, "SOL A"=TRUE, "SOL B"=FALSE, "Lift Up"=FALSE, "Lift Down"=FALSE, "Intake In"=FALSE, "Intake Out"=FALSE, "Left Distance"=0.0, "Right Distance"=0.0, "Drive?"=FALSE, "Wrist Up"=FALSE, "Wrist Down"=FALSE, "Lift Target"=0.0, "Wrist Target"=0.0}, {"Left Joystick"=-0.975, "Right Joystick"=-1.0, "Duration"=5.0, "SOL A"=TRUE, "SOL B"=FALSE, "Lift Up"=TRUE, "Lift Down"=FALSE, "Intake In"=FALSE, "Intake Out"=FALSE, "Left Distance"=18.2, "Right Distance"=18.2, "Drive?"=TRUE, "Wrist Up"=TRUE, "Wrist Down"=FALSE, "Lift Target"=15.0, "Wrist Target"=45.0}, {"Left Joystick"=0.0, "Right Joystick"=0.0, "Duration"=0.75, "SOL A"=TRUE, "SOL B"=FALSE, "Lift Up"=FALSE, "Lift Down"=FALSE, "Intake In"=FALSE, "Intake Out"=TRUE, "Left Distance"=0.0, "Right Distance"=0.0, "Drive?"=FALSE, "Wrist Up"=FALSE, "Wrist Down"=FALSE, "Lift Target"=0.0, "Wrist Target"=0.0}, {"Left Joystick"=0.975, "Right Joystick"=1.0, "Duration"=5.0, "SOL A"=TRUE, "SOL B"=FALSE, "Lift Up"=FALSE, "Lift Down"=FALSE, "Intake In"=FALSE, "Intake Out"=FALSE, "Left Distance"=18.2, "Right Distance"=18.2, "Drive?"=TRUE, "Wrist Up"=FALSE, "Wrist Down"=FALSE, "Lift Target"=0.0, "Wrist Target"=0.0}, {"Left Joystick"=0.0, "Right Joystick"=0.0, "Duration"=0.5, "SOL A"=TRUE, "SOL B"=FALSE, "Lift Up"=FALSE, "Lift Down"=FALSE, "Intake In"=FALSE, "Intake Out"=FALSE, "Left Distance"=0.0, "Right Distance"=0.0, "Drive?"=FALSE, "Wrist Up"=FALSE, "Wrist Down"=FALSE, "Lift Target"=0.0, "Wrist Target"=0.0}, {"Left Joystick"=-0.975, "Right Joystick"=1.0, "Duration"=5.0, "SOL A"=FALSE, "SOL B"=TRUE, "Lift Up"=FALSE, "Lift Down"=FALSE, "Intake In"=FALSE, "Intake Out"=FALSE, "Left Distance"=27.0, "Right Distance"=27.0, "Drive?"=TRUE, "Wrist Up"=FALSE, "Wrist Down"=FALSE, "Lift Target"=0.0, "Wrist Target"=0.0}, {"Left Joystick"=0.0, "Right Joystick"=0.0, "Duration"=0.5, "SOL A"=TRUE, "SOL B"=FALSE, "Lift Up"=FALSE, "Lift Down"=FALSE, "Intake In"=FALSE, "Intake Out"=FALSE, "Left Distance"=0.0, "Right Distance"=0.0, "Drive?"=FALSE, "Wrist Up"=FALSE, "Wrist Down"=FALSE, "Lift Target"=0.0, "Wrist Target"=0.0}, {"Left Joystick"=0.975, "Right Joystick"=1.0, "Duration"=5.0, "SOL A"=TRUE, "SOL B"=FALSE, "Lift Up"=FALSE, "Lift Down"=FALSE, "Intake In"=FALSE, "Intake Out"=FALSE, "Left Distance"=19.7, "Right Distance"=19.7, "Drive?"=TRUE, "Wrist Up"=FALSE, "Wrist Down"=FALSE, "Lift Target"=0.0, "Wrist Target"=0.0}, {"Left Joystick"=0.0, "Right Joystick"=0.0, "Duration"=0.5, "SOL A"=TRUE, "SOL B"=FALSE, "Lift Up"=FALSE, "Lift Down"=FALSE, "Intake In"=FALSE, "Intake Out"=FALSE, "Left Distance"=0.0, "Right Distance"=0.0, "Drive?"=FALSE, "Wrist Up"=FALSE, "Wrist Down"=FALSE, "Lift Target"=0.0, "Wrist Target"=0.0}, {"Left Joystick"=0.975, "Right Joystick"=-1.0, "Duration"=5.0, "SOL A"=FALSE, "SOL B"=TRUE, "Lift Up"=FALSE, "Lift Down"=FALSE, "Intake In"=FALSE, "Intake Out"=FALSE, "Left Distance"=25.6, "Right Distance"=25.6, "Drive?"=TRUE, "Wrist Up"=FALSE, "Wrist Down"=FALSE, "Lift Target"=0.0, "Wrist Target"=0.0}, {"Left Joystick"=0.0, "Right Joystick"=0.0, "Duration"=0.5, "SOL A"=TRUE, "SOL B"=FALSE, "Lift Up"=FALSE, "Lift Down"=FALSE, "Intake In"=FALSE, "Intake Out"=FALSE, "Left Distance"=0.0, "Right Distance"=0.0, "Drive?"=FALSE, "Wrist Up"=FALSE, "Wrist Down"=FALSE, "Lift Target"=0.0, "Wrist Target"=0.0}, {"Left Joystick"=-0.975, "Right Joystick"=-1.0, "Duration"=5.0, "SOL A"=TRUE, "SOL B"=FALSE, "Lift Up"=FALSE, "Lift Down"=FALSE, "Intake In"=FALSE, "Intake Out"=FALSE, "Left Distance"=4.0, "Right Distance"=4.0, "Drive?"=TRUE, "Wrist Up"=FALSE, "Wrist Down"=FALSE, "Lift Target"=0.0, "Wrist Target"=0.0}, {"Left Joystick"=0.0, "Right Joystick"=0.0, "Duration"=0.75, "SOL A"=TRUE, "SOL B"=FALSE, "Lift Up"=FALSE, "Lift Down"=FALSE, "Intake In"=TRUE, "Intake Out"=FALSE, "Left Distance"=0.0, "Right Distance"=0.0, "Drive?"=FALSE, "Wrist Up"=FALSE, "Wrist Down"=FALSE, "Lift Target"=0.0, "Wrist Target"=0.0}, {"Left Joystick"=0.975, "Right Joystick"=1.0, "Duration"=5.0, "SOL A"=TRUE, "SOL B"=FALSE, "Lift Up"=FALSE, "Lift Down"=FALSE, "Intake In"=FALSE, "Intake Out"=FALSE, "Left Distance"=4.0, "Right Distance"=4.0, "Drive?"=TRUE, "Wrist Up"=FALSE, "Wrist Down"=FALSE, "Lift Target"=0.0, "Wrist Target"=0.0}, {"Left Joystick"=0.0, "Right Joystick"=0.0, "Duration"=0.5, "SOL A"=TRUE, "SOL B"=FALSE, "Lift Up"=FALSE, "Lift Down"=FALSE, "Intake In"=FALSE, "Intake Out"=FALSE, "Left Distance"=0.0, "Right Distance"=0.0, "Drive?"=FALSE, "Wrist Up"=FALSE, "Wrist Down"=FALSE, "Lift Target"=0.0, "Wrist Target"=0.0}, {"Left Joystick"=-0.975, "Right Joystick"=-1.0, "Duration"=5.0, "SOL A"=TRUE, "SOL B"=FALSE, "Lift Up"=FALSE, "Lift Down"=FALSE, "Intake In"=FALSE, "Intake Out"=FALSE, "Left Distance"=30.1, "Right Distance"=30.1, "Drive?"=TRUE, "Wrist Up"=FALSE, "Wrist Down"=FALSE, "Lift Target"=0.0, "Wrist Target"=0.0}, {"Left Joystick"=0.0, "Right Joystick"=0.0, "Duration"=0.5, "SOL A"=TRUE, "SOL B"=FALSE, "Lift Up"=FALSE, "Lift Down"=FALSE, "Intake In"=FALSE, "Intake Out"=FALSE, "Left Distance"=0.0, "Right Distance"=0.0, "Drive?"=FALSE, "Wrist Up"=FALSE, "Wrist Down"=FALSE, "Lift Target"=0.0, "Wrist Target"=0.0}, {"Left Joystick"=-0.975, "Right Joystick"=-1.0, "Duration"=5.0, "SOL A"=TRUE, "SOL B"=FALSE, "Lift Up"=TRUE, "Lift Down"=FALSE, "Intake In"=FALSE, "Intake Out"=FALSE, "Left Distance"=25.0, "Right Distance"=25.0, "Drive?"=TRUE, "Wrist Up"=TRUE, "Wrist Down"=FALSE, "Lift Target"=50.0, "Wrist Target"=45.0}, {"Left Joystick"=0.0, "Right Joystick"=0.0, "Duration"=0.75, "SOL A"=TRUE, "SOL B"=FALSE, "Lift Up"=FALSE, "Lift Down"=FALSE, "Intake In"=FALSE, "Intake Out"=TRUE, "Left Distance"=0.0, "Right Distance"=0.0, "Drive?"=FALSE, "Wrist Up"=FALSE, "Wrist Down"=FALSE, "Lift Target"=0.0, "Wrist Target"=0.0}]
  in  "Left LRL":T1(array[cluster])=[{"Left Joystick"=0.975, "Right Joystick"=1.0, "Duration"=5.0, "SOL A"=TRUE, "SOL B"=FALSE, "Lift Up"=FALSE, "Lift Down"=FALSE, "Intake In"=FALSE, "Intake Out"=FALSE, "Left Distance"=199.6, "Right Distance"=199.6, "Drive?"=TRUE, "Wrist Up"=FALSE, "Wrist Down"=FALSE, "Lift Target"=0.0, "Wrist Target"=0.0}, {"Left Joystick"=0.0, "Right Joystick"=0.0, "Duration"=0.5, "SOL A"=TRUE, "SOL B"=FALSE, "Lift Up"=FALSE, "Lift Down"=FALSE, "Intake In"=FALSE, "Intake Out"=FALSE, "Left Distance"=0.0, "Right Distance"=0.0, "Drive?"=FALSE, "Wrist Up"=FALSE, "Wrist Down"=FALSE, "Lift Target"=0.0, "Wrist Target"=0.0}, {"Left Joystick"=0.975, "Right Joystick"=-1.0, "Duration"=5.0, "SOL A"=FALSE, "SOL B"=TRUE, "Lift Up"=FALSE, "Lift Down"=FALSE, "Intake In"=FALSE, "Intake Out"=FALSE, "Left Distance"=13.2, "Right Distance"=13.2, "Drive?"=TRUE, "Wrist Up"=FALSE, "Wrist Down"=FALSE, "Lift Target"=0.0, "Wrist Target"=0.0}, {"Left Joystick"=0.0, "Right Joystick"=0.0, "Duration"=0.5, "SOL A"=TRUE, "SOL B"=FALSE, "Lift Up"=FALSE, "Lift Down"=FALSE, "Intake In"=FALSE, "Intake Out"=FALSE, "Left Distance"=0.0, "Right Distance"=0.0, "Drive?"=FALSE, "Wrist Up"=FALSE, "Wrist Down"=FALSE, "Lift Target"=0.0, "Wrist Target"=0.0}, {"Left Joystick"=-0.975, "Right Joystick"=-1.0, "Duration"=5.0, "SOL A"=TRUE, "SOL B"=FALSE, "Lift Up"=TRUE, "Lift Down"=FALSE, "Intake In"=FALSE, "Intake Out"=FALSE, "Left Distance"=18.2, "Right Distance"=18.2, "Drive?"=TRUE, "Wrist Up"=TRUE, "Wrist Down"=FALSE, "Lift Target"=15.0, "Wrist Target"=45.0}, {"Left Joystick"=0.0, "Right Joystick"=0.0, "Duration"=0.75, "SOL A"=TRUE, "SOL B"=FALSE, "Lift Up"=FALSE, "Lift Down"=FALSE, "Intake In"=FALSE, "Intake Out"=TRUE, "Left Distance"=0.0, "Right Distance"=0.0, "Drive?"=FALSE, "Wrist Up"=FALSE, "Wrist Down"=FALSE, "Lift Target"=0.0, "Wrist Target"=0.0}, {"Left Joystick"=0.975, "Right Joystick"=1.0, "Duration"=5.0, "SOL A"=TRUE, "SOL B"=FALSE, "Lift Up"=FALSE, "Lift Down"=FALSE, "Intake In"=FALSE, "Intake Out"=FALSE, "Left Distance"=18.2, "Right Distance"=18.2, "Drive?"=TRUE, "Wrist Up"=FALSE, "Wrist Down"=FALSE, "Lift Target"=0.0, "Wrist Target"=80.0}, {"Left Joystick"=0.0, "Right Joystick"=0.0, "Duration"=0.5, "SOL A"=TRUE, "SOL B"=FALSE, "Lift Up"=FALSE, "Lift Down"=FALSE, "Intake In"=FALSE, "Intake Out"=FALSE, "Left Distance"=0.0, "Right Distance"=0.0, "Drive?"=FALSE, "Wrist Up"=FALSE, "Wrist Down"=FALSE, "Lift Target"=0.0, "Wrist Target"=0.0}, {"Left Joystick"=-0.975, "Right Joystick"=1.0, "Duration"=5.0, "SOL A"=FALSE, "SOL B"=TRUE, "Lift Up"=FALSE, "Lift Down"=FALSE, "Intake In"=FALSE, "Intake Out"=FALSE, "Left Distance"=27.0, "Right Distance"=27.0, "Drive?"=TRUE, "Wrist Up"=FALSE, "Wrist Down"=FALSE, "Lift Target"=0.0, "Wrist Target"=0.0}, {"Left Joystick"=0.0, "Right Joystick"=0.0, "Duration"=0.5, "SOL A"=TRUE, "SOL B"=FALSE, "Lift Up"=FALSE, "Lift Down"=FALSE, "Intake In"=FALSE, "Intake Out"=FALSE, "Left Distance"=0.0, "Right Distance"=0.0, "Drive?"=FALSE, "Wrist Up"=FALSE, "Wrist Down"=FALSE, "Lift Target"=0.0, "Wrist Target"=0.0}, {"Left Joystick"=0.975, "Right Joystick"=1.0, "Duration"=5.0, "SOL A"=TRUE, "SOL B"=FALSE, "Lift Up"=FALSE, "Lift Down"=FALSE, "Intake In"=FALSE, "Intake Out"=FALSE, "Left Distance"=19.7, "Right Distance"=19.7, "Drive?"=TRUE, "Wrist Up"=FALSE, "Wrist Down"=FALSE, "Lift Target"=0.0, "Wrist Target"=0.0}, {"Left Joystick"=0.0, "Right Joystick"=0.0, "Duration"=0.5, "SOL A"=FALSE, "SOL B"=FALSE, "Lift Up"=FALSE, "Lift Down"=FALSE, "Intake In"=FALSE, "Intake Out"=FALSE, "Left Distance"=0.0, "Right Distance"=0.0, "Drive?"=FALSE, "Wrist Up"=FALSE, "Wrist Down"=FALSE, "Lift Target"=0.0, "Wrist Target"=0.0}, {"Left Joystick"=-0.975, "Right Joystick"=1.0, "Duration"=5.0, "SOL A"=TRUE, "SOL B"=FALSE, "Lift Up"=FALSE, "Lift Down"=FALSE, "Intake In"=FALSE, "Intake Out"=FALSE, "Left Distance"=25.6, "Right Distance"=25.6, "Drive?"=TRUE, "Wrist Up"=FALSE, "Wrist Down"=FALSE, "Lift Target"=0.0, "Wrist Target"=0.0}, {"Left Joystick"=0.0, "Right Joystick"=0.0, "Duration"=0.5, "SOL A"=TRUE, "SOL B"=FALSE, "Lift Up"=FALSE, "Lift Down"=FALSE, "Intake In"=FALSE, "Intake Out"=FALSE, "Left Distance"=0.0, "Right Distance"=0.0, "Drive?"=FALSE, "Wrist Up"=FALSE, "Wrist Down"=FALSE, "Lift Target"=0.0, "Wrist Target"=0.0}, {"Left Joystick"=-0.975, "Right Joystick"=-1.0, "Duration"=5.0, "SOL A"=TRUE, "SOL B"=FALSE, "Lift Up"=FALSE, "Lift Down"=FALSE, "Intake In"=FALSE, "Intake Out"=FALSE, "Left Distance"=4.0, "Right Distance"=4.0, "Drive?"=TRUE, "Wrist Up"=FALSE, "Wrist Down"=FALSE, "Lift Target"=0.0, "Wrist Target"=0.0}, {"Left Joystick"=0.0, "Right Joystick"=0.0, "Duration"=0.75, "SOL A"=TRUE, "SOL B"=FALSE, "Lift Up"=FALSE, "Lift Down"=FALSE, "Intake In"=TRUE, "Intake Out"=FALSE, "Left Distance"=0.0, "Right Distance"=0.0, "Drive?"=TRUE, "Wrist Up"=FALSE, "Wrist Down"=FALSE, "Lift Target"=0.0, "Wrist Target"=0.0}]
  in  "Testing":T1(array[cluster])=[{"Left Joystick"=0.975, "Right Joystick"=1.0, "Duration"=5.0, "SOL A"=TRUE, "SOL B"=FALSE, "Lift Up"=FALSE, "Lift Down"=FALSE, "Intake In"=FALSE, "Intake Out"=FALSE, "Left Distance"=199.6, "Right Distance"=199.6, "Drive?"=TRUE, "Wrist Up"=FALSE, "Wrist Down"=FALSE, "Lift Target"=0.0, "Wrist Target"=0.0}, {"Left Joystick"=0.0, "Right Joystick"=0.0, "Duration"=0.5, "SOL A"=TRUE, "SOL B"=FALSE, "Lift Up"=FALSE, "Lift Down"=FALSE, "Intake In"=FALSE, "Intake Out"=FALSE, "Left Distance"=0.0, "Right Distance"=0.0, "Drive?"=FALSE, "Wrist Up"=FALSE, "Wrist Down"=FALSE, "Lift Target"=0.0, "Wrist Target"=0.0}, {"Left Joystick"=0.975, "Right Joystick"=-1.0, "Duration"=5.0, "SOL A"=FALSE, "SOL B"=TRUE, "Lift Up"=FALSE, "Lift Down"=FALSE, "Intake In"=FALSE, "Intake Out"=FALSE, "Left Distance"=13.2, "Right Distance"=13.2, "Drive?"=TRUE, "Wrist Up"=FALSE, "Wrist Down"=FALSE, "Lift Target"=0.0, "Wrist Target"=0.0}, {"Left Joystick"=0.0, "Right Joystick"=0.0, "Duration"=0.5, "SOL A"=TRUE, "SOL B"=FALSE, "Lift Up"=FALSE, "Lift Down"=FALSE, "Intake In"=FALSE, "Intake Out"=FALSE, "Left Distance"=0.0, "Right Distance"=0.0, "Drive?"=FALSE, "Wrist Up"=FALSE, "Wrist Down"=FALSE, "Lift Target"=0.0, "Wrist Target"=0.0}, {"Left Joystick"=-0.975, "Right Joystick"=-1.0, "Duration"=5.0, "SOL A"=TRUE, "SOL B"=FALSE, "Lift Up"=TRUE, "Lift Down"=FALSE, "Intake In"=FALSE, "Intake Out"=FALSE, "Left Distance"=18.2, "Right Distance"=18.2, "Drive?"=TRUE, "Wrist Up"=TRUE, "Wrist Down"=FALSE, "Lift Target"=0.0, "Wrist Target"=0.0}, {"Left Joystick"=0.0, "Right Joystick"=0.0, "Duration"=0.75, "SOL A"=TRUE, "SOL B"=FALSE, "Lift Up"=TRUE, "Lift Down"=FALSE, "Intake In"=FALSE, "Intake Out"=TRUE, "Left Distance"=0.0, "Right Distance"=0.0, "Drive?"=FALSE, "Wrist Up"=TRUE, "Wrist Down"=FALSE, "Lift Target"=15.0, "Wrist Target"=45.0}, {"Left Joystick"=0.975, "Right Joystick"=1.0, "Duration"=5.0, "SOL A"=TRUE, "SOL B"=FALSE, "Lift Up"=FALSE, "Lift Down"=FALSE, "Intake In"=FALSE, "Intake Out"=FALSE, "Left Distance"=18.2, "Right Distance"=18.2, "Drive?"=TRUE, "Wrist Up"=FALSE, "Wrist Down"=FALSE, "Lift Target"=1.0, "Wrist Target"=0.0}, {"Left Joystick"=0.0, "Right Joystick"=0.0, "Duration"=0.5, "SOL A"=TRUE, "SOL B"=FALSE, "Lift Up"=FALSE, "Lift Down"=FALSE, "Intake In"=FALSE, "Intake Out"=FALSE, "Left Distance"=0.0, "Right Distance"=0.0, "Drive?"=FALSE, "Wrist Up"=FALSE, "Wrist Down"=FALSE, "Lift Target"=0.0, "Wrist Target"=0.0}, {"Left Joystick"=-0.975, "Right Joystick"=1.0, "Duration"=5.0, "SOL A"=FALSE, "SOL B"=TRUE, "Lift Up"=FALSE, "Lift Down"=FALSE, "Intake In"=FALSE, "Intake Out"=FALSE, "Left Distance"=27.0, "Right Distance"=27.0, "Drive?"=TRUE, "Wrist Up"=FALSE, "Wrist Down"=FALSE, "Lift Target"=0.0, "Wrist Target"=0.0}, {"Left Joystick"=0.0, "Right Joystick"=0.0, "Duration"=0.5, "SOL A"=TRUE, "SOL B"=FALSE, "Lift Up"=FALSE, "Lift Down"=FALSE, "Intake In"=FALSE, "Intake Out"=FALSE, "Left Distance"=0.0, "Right Distance"=0.0, "Drive?"=FALSE, "Wrist Up"=FALSE, "Wrist Down"=FALSE, "Lift Target"=0.0, "Wrist Target"=0.0}, {"Left Joystick"=0.975, "Right Joystick"=1.0, "Duration"=5.0, "SOL A"=TRUE, "SOL B"=FALSE, "Lift Up"=FALSE, "Lift Down"=FALSE, "Intake In"=FALSE, "Intake Out"=FALSE, "Left Distance"=19.7, "Right Distance"=19.7, "Drive?"=TRUE, "Wrist Up"=FALSE, "Wrist Down"=FALSE, "Lift Target"=0.0, "Wrist Target"=0.0}, {"Left Joystick"=0.0, "Right Joystick"=0.0, "Duration"=0.5, "SOL A"=TRUE, "SOL B"=FALSE, "Lift Up"=FALSE, "Lift Down"=FALSE, "Intake In"=FALSE, "Intake Out"=FALSE, "Left Distance"=0.0, "Right Distance"=0.0, "Drive?"=FALSE, "Wrist Up"=FALSE, "Wrist Down"=FALSE, "Lift Target"=0.0, "Wrist Target"=0.0}, {"Left Joystick"=0.975, "Right Joystick"=-1.0, "Duration"=5.0, "SOL A"=FALSE, "SOL B"=TRUE, "Lift Up"=FALSE, "Lift Down"=FALSE, "Intake In"=FALSE, "Intake Out"=FALSE, "Left Distance"=25.6, "Right Distance"=25.6, "Drive?"=TRUE, "Wrist Up"=FALSE, "Wrist Down"=FALSE, "Lift Target"=0.0, "Wrist Target"=0.0}, {"Left Joystick"=0.0, "Right Joystick"=0.0, "Duration"=0.5, "SOL A"=TRUE, "SOL B"=FALSE, "Lift Up"=FALSE, "Lift Down"=FALSE, "Intake In"=FALSE, "Intake Out"=FALSE, "Left Distance"=0.0, "Right Distance"=0.0, "Drive?"=FALSE, "Wrist Up"=FALSE, "Wrist Down"=FALSE, "Lift Target"=0.0, "Wrist Target"=0.0}, {"Left Joystick"=-0.0975, "Right Joystick"=-1.0, "Duration"=5.0, "SOL A"=TRUE, "SOL B"=FALSE, "Lift Up"=FALSE, "Lift Down"=FALSE, "Intake In"=FALSE, "Intake Out"=FALSE, "Left Distance"=4.0, "Right Distance"=4.0, "Drive?"=TRUE, "Wrist Up"=FALSE, "Wrist Down"=FALSE, "Lift Target"=0.0, "Wrist Target"=0.0}, {"Left Joystick"=0.0, "Right Joystick"=0.0, "Duration"=0.75, "SOL A"=TRUE, "SOL B"=FALSE, "Lift Up"=FALSE, "Lift Down"=FALSE, "Intake In"=TRUE, "Intake Out"=FALSE, "Left Distance"=0.0, "Right Distance"=0.0, "Drive?"=FALSE, "Wrist Up"=FALSE, "Wrist Down"=FALSE, "Lift Target"=0.0, "Wrist Target"=0.0}, {"Left Joystick"=0.975, "Right Joystick"=1.0, "Duration"=5.0, "SOL A"=TRUE, "SOL B"=FALSE, "Lift Up"=FALSE, "Lift Down"=FALSE, "Intake In"=FALSE, "Intake Out"=FALSE, "Left Distance"=4.0, "Right Distance"=4.0, "Drive?"=TRUE, "Wrist Up"=FALSE, "Wrist Down"=FALSE, "Lift Target"=0.0, "Wrist Target"=0.0}, {"Left Joystick"=0.0, "Right Joystick"=0.0, "Duration"=0.5, "SOL A"=TRUE, "SOL B"=FALSE, "Lift Up"=FALSE, "Lift Down"=FALSE, "Intake In"=FALSE, "Intake Out"=FALSE, "Left Distance"=0.0, "Right Distance"=0.0, "Drive?"=FALSE, "Wrist Up"=FALSE, "Wrist Down"=FALSE, "Lift Target"=0.0, "Wrist Target"=0.0}, {"Left Joystick"=0.975, "Right Joystick"=-1.0, "Duration"=5.0, "SOL A"=FALSE, "SOL B"=TRUE, "Lift Up"=FALSE, "Lift Down"=FALSE, "Intake In"=FALSE, "Intake Out"=FALSE, "Left Distance"=30.1, "Right Distance"=30.1, "Drive?"=TRUE, "Wrist Up"=FALSE, "Wrist Down"=FALSE, "Lift Target"=0.0, "Wrist Target"=0.0}, {"Left Joystick"=0.0, "Right Joystick"=0.0, "Duration"=0.5, "SOL A"=TRUE, "SOL B"=FALSE, "Lift Up"=FALSE, "Lift Down"=FALSE, "Intake In"=FALSE, "Intake Out"=FALSE, "Left Distance"=0.0, "Right Distance"=0.0, "Drive?"=FALSE, "Wrist Up"=FALSE, "Wrist Down"=FALSE, "Lift Target"=0.0, "Wrist Target"=0.0}, {"Left Joystick"=-0.975, "Right Joystick"=-1.0, "Duration"=5.0, "SOL A"=TRUE, "SOL B"=FALSE, "Lift Up"=TRUE, "Lift Down"=FALSE, "Intake In"=FALSE, "Intake Out"=FALSE, "Left Distance"=25.0, "Right Distance"=25.0, "Drive?"=TRUE, "Wrist Up"=TRUE, "Wrist Down"=FALSE, "Lift Target"=50.0, "Wrist Target"=45.0}, {"Left Joystick"=0.0, "Right Joystick"=0.0, "Duration"=0.75, "SOL A"=TRUE, "SOL B"=FALSE, "Lift Up"=FALSE, "Lift Down"=FALSE, "Intake In"=FALSE, "Intake Out"=TRUE, "Left Distance"=0.0, "Right Distance"=0.0, "Drive?"=FALSE, "Wrist Up"=FALSE, "Wrist Down"=FALSE, "Lift Target"=0.0, "Wrist Target"=0.0}]
  # "Be sure to right-click and choose Data Operations>>Make Current Value default if you want to save the array values with the VI"
types:
  T1 = cluster{"Left Joystick":dbl, "Right Joystick":dbl, "Duration":dbl, "SOL A":bool, "SOL B":bool, "Lift Up":bool, "Lift Down":bool, "Intake In":bool, "Intake Out":bool, "Left Distance":dbl, "Right Distance":dbl, "Drive?":bool, "Wrist Up":bool, "Wrist Down":bool, "Lift Target":dbl, "Wrist Target":dbl}[]
  T2 = typedef "WPI_JoystickDevRef.ctl" = cluster{"Device":T3}
  T3 = typedef "WPI_JoystickDeviceEnum.ctl" = enum16{"USB 0", "USB 1", "USB 2", "USB 3", "USB 4", "USB 5"}
  T4 = typedef "WPI_RobotDriveDevRef.ctl" = cluster{"DevStatus":errorcluster, "Motors[]":T5[], "Square Inputs":bool, "Max Output":dbl}
  T5 = typedef "WPI_MotorControlDeviceRef.ctl" = cluster{"DeviceStatus":errorcluster, "Type":T6, "PWM":cluster{"PWM Channel":T7, "DeadBand":T8}, "CAN":cluster{"Device Number":u8, "SetOutput VI Ref":variant, "GetOutput VI Ref":variant, "Enable VI Ref":variant, "Disable VI Ref":variant, "Data":variant}, "Invert":bool, "DIO PWM":cluster{"PWM \"Enable\" Channel":T7, "DIOChannel":T9, "PWM Rate":dbl}}
  T6 = typedef "WPI_MotorControlType.ctl" = enum16{"PWM", "CAN", "DIO PWM"}
  T7 = typedef "FPGA_DIOPWMChannel.ctl" = enum8{"PWM 0", "PWM 1", "PWM 2", "PWM 3", "PWM 4", "PWM 5", "PWM 6", "PWM 7", "PWM 8", "PWM 9", "PWM MXP 0", "PWM MXP 1", "PWM MXP 2", "PWM MXP 3", "PWM MXP 4", "PWM MXP 5", "PWM MXP 6", "PWM MXP 7", "PWM MXP 8", "PWM MXP 9", "Invalid"}
  T8 = typedef "WPI_PWMDeadband.ctl" = cluster{"Name":string, "maxPositivePwm":i32, "minPositivePwm":i32, "centerPwm":i32, "maxNegativePwm":i32, "minNegativePwm":i32, "angularRange":u16}
  T9 = typedef "FPGA_DIOChannel.ctl" = enum8{"DIO 0", "DIO 1", "DIO 2", "DIO 3", "DIO 4", "DIO 5", "DIO 6", "DIO 7", "DIO 8", "DIO 9", "DIO MXP 0", "DIO MXP 1", "DIO MXP 2", "DIO MXP 3", "DIO MXP 4", "DIO MXP 5", "DIO MXP 6", "DIO MXP 7", "DIO MXP 8", "DIO MXP 9", "DIO MXP 10", "DIO MXP 11", "DIO MXP 12", "DIO MXP 13", "DIO MXP 14", "DIO MXP 15", "SPI Port CS1", "SPI Port CS2", "SPI Port CS3", "SPI Port MISO", "SPI Port MOSI", "Invalid"}
  T10 = typedef "WPI_SolenoidDevRef.ctl" = cluster{"DevStatus":errorcluster, "Pneumatics Control Module":u8, "Forward Solenoid Channel":T11, "Reverse Solenoid Channel":T11}
  T11 = typedef "WPI_SolenoidChannel.ctl" = enum8{"Solenoid 0", "Solenoid 1", "Solenoid 2", "Solenoid 3", "Solenoid 4", "Solenoid 5", "Solenoid 6", "Solenoid 7", "Invalid"}
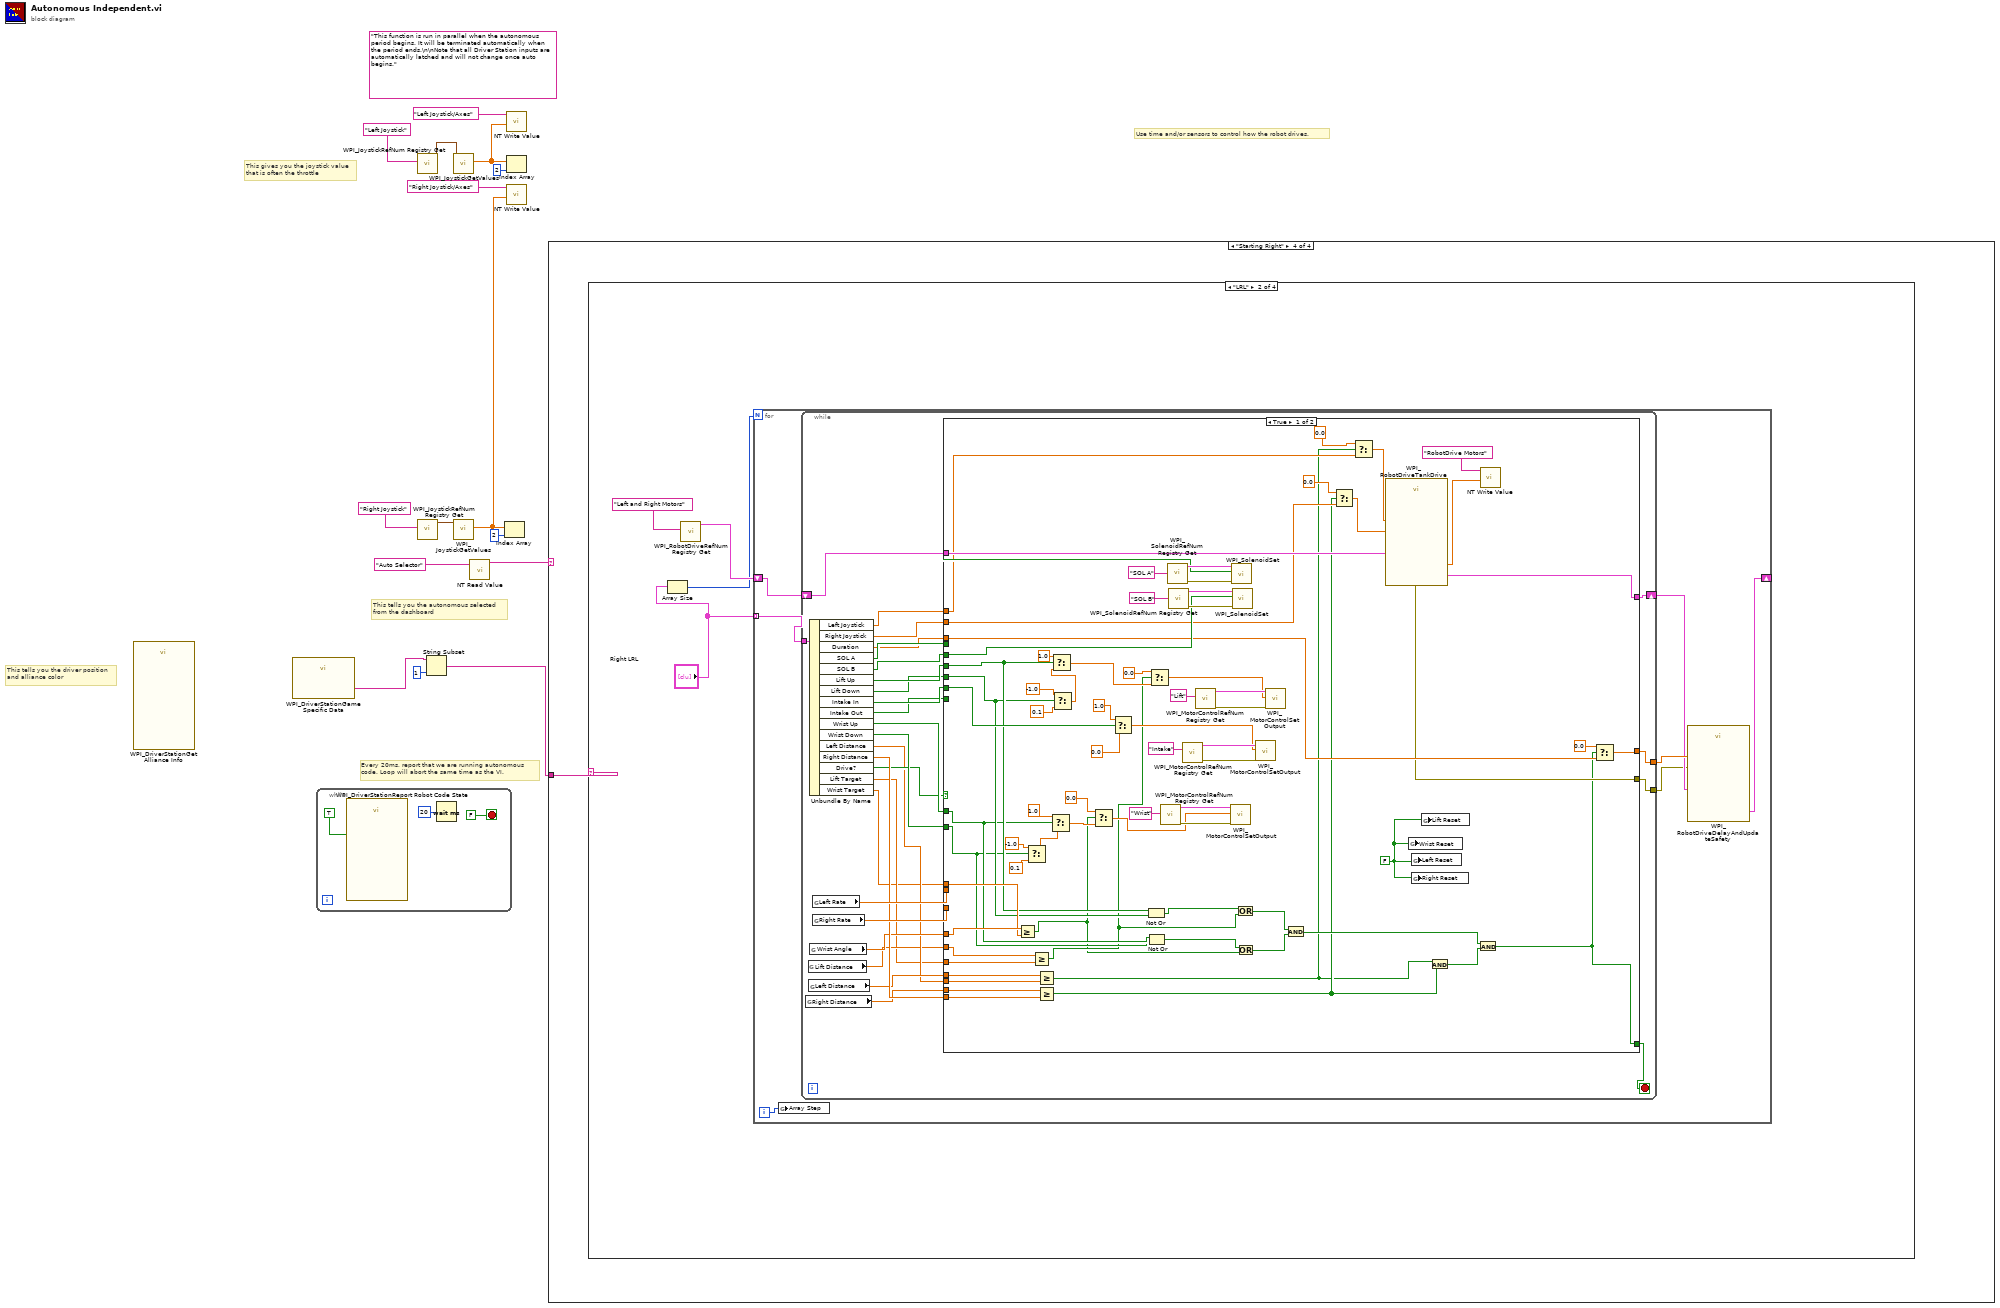
[diagram p0: block diagram]
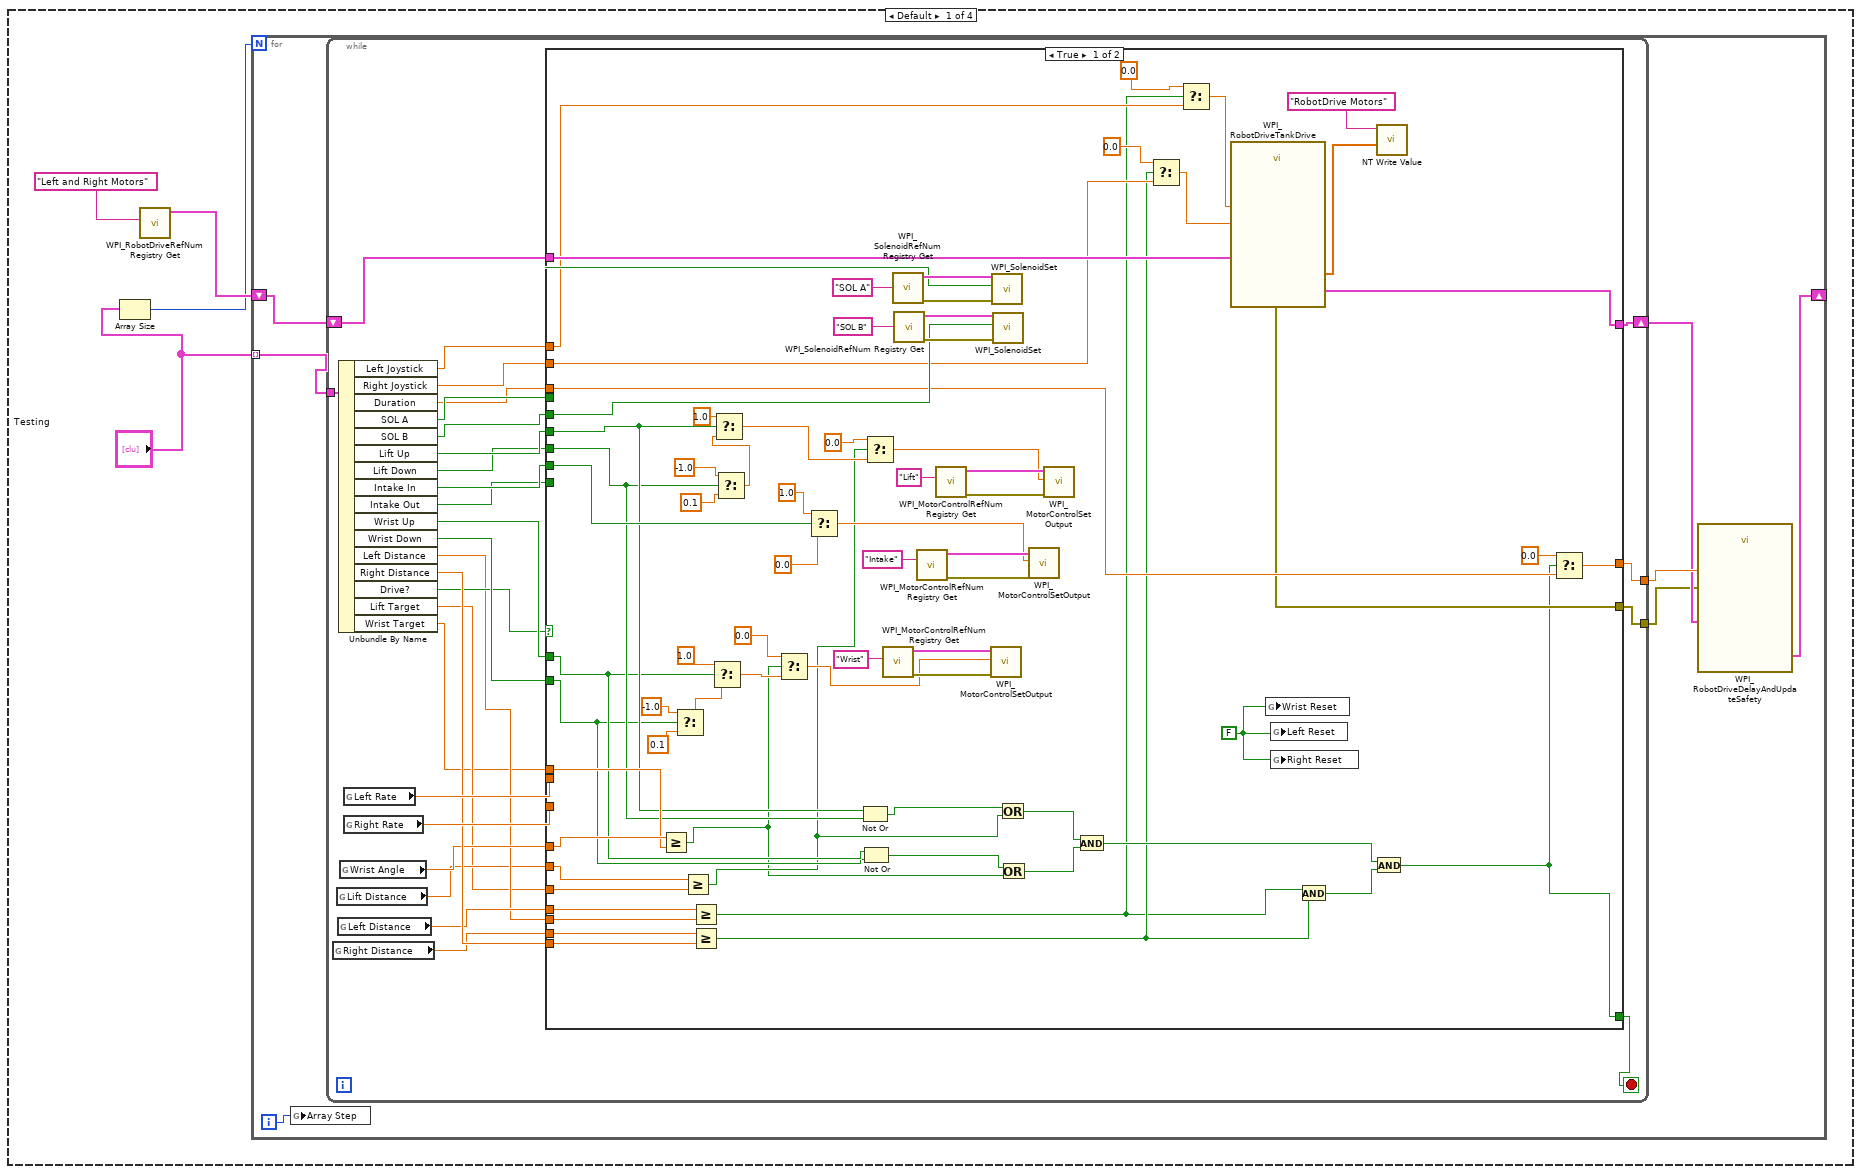
[diagram p2: hidden frame]
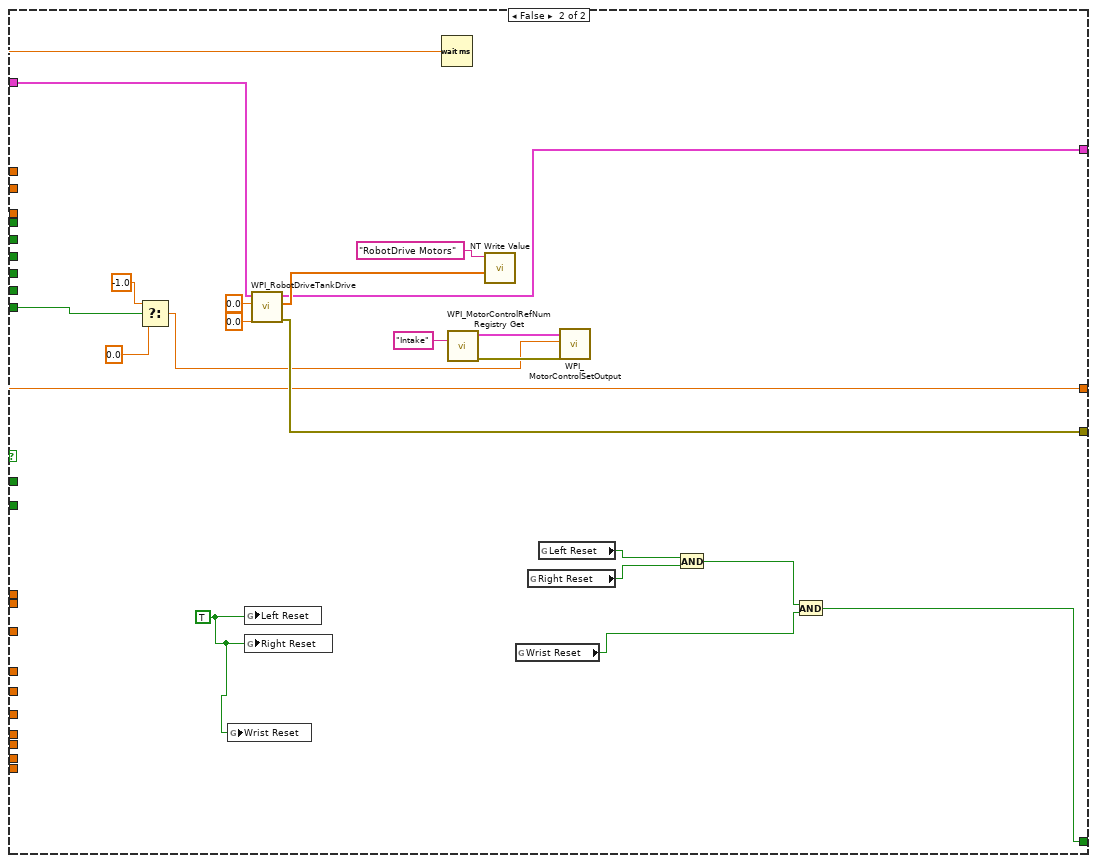
[diagram p3: hidden frame]
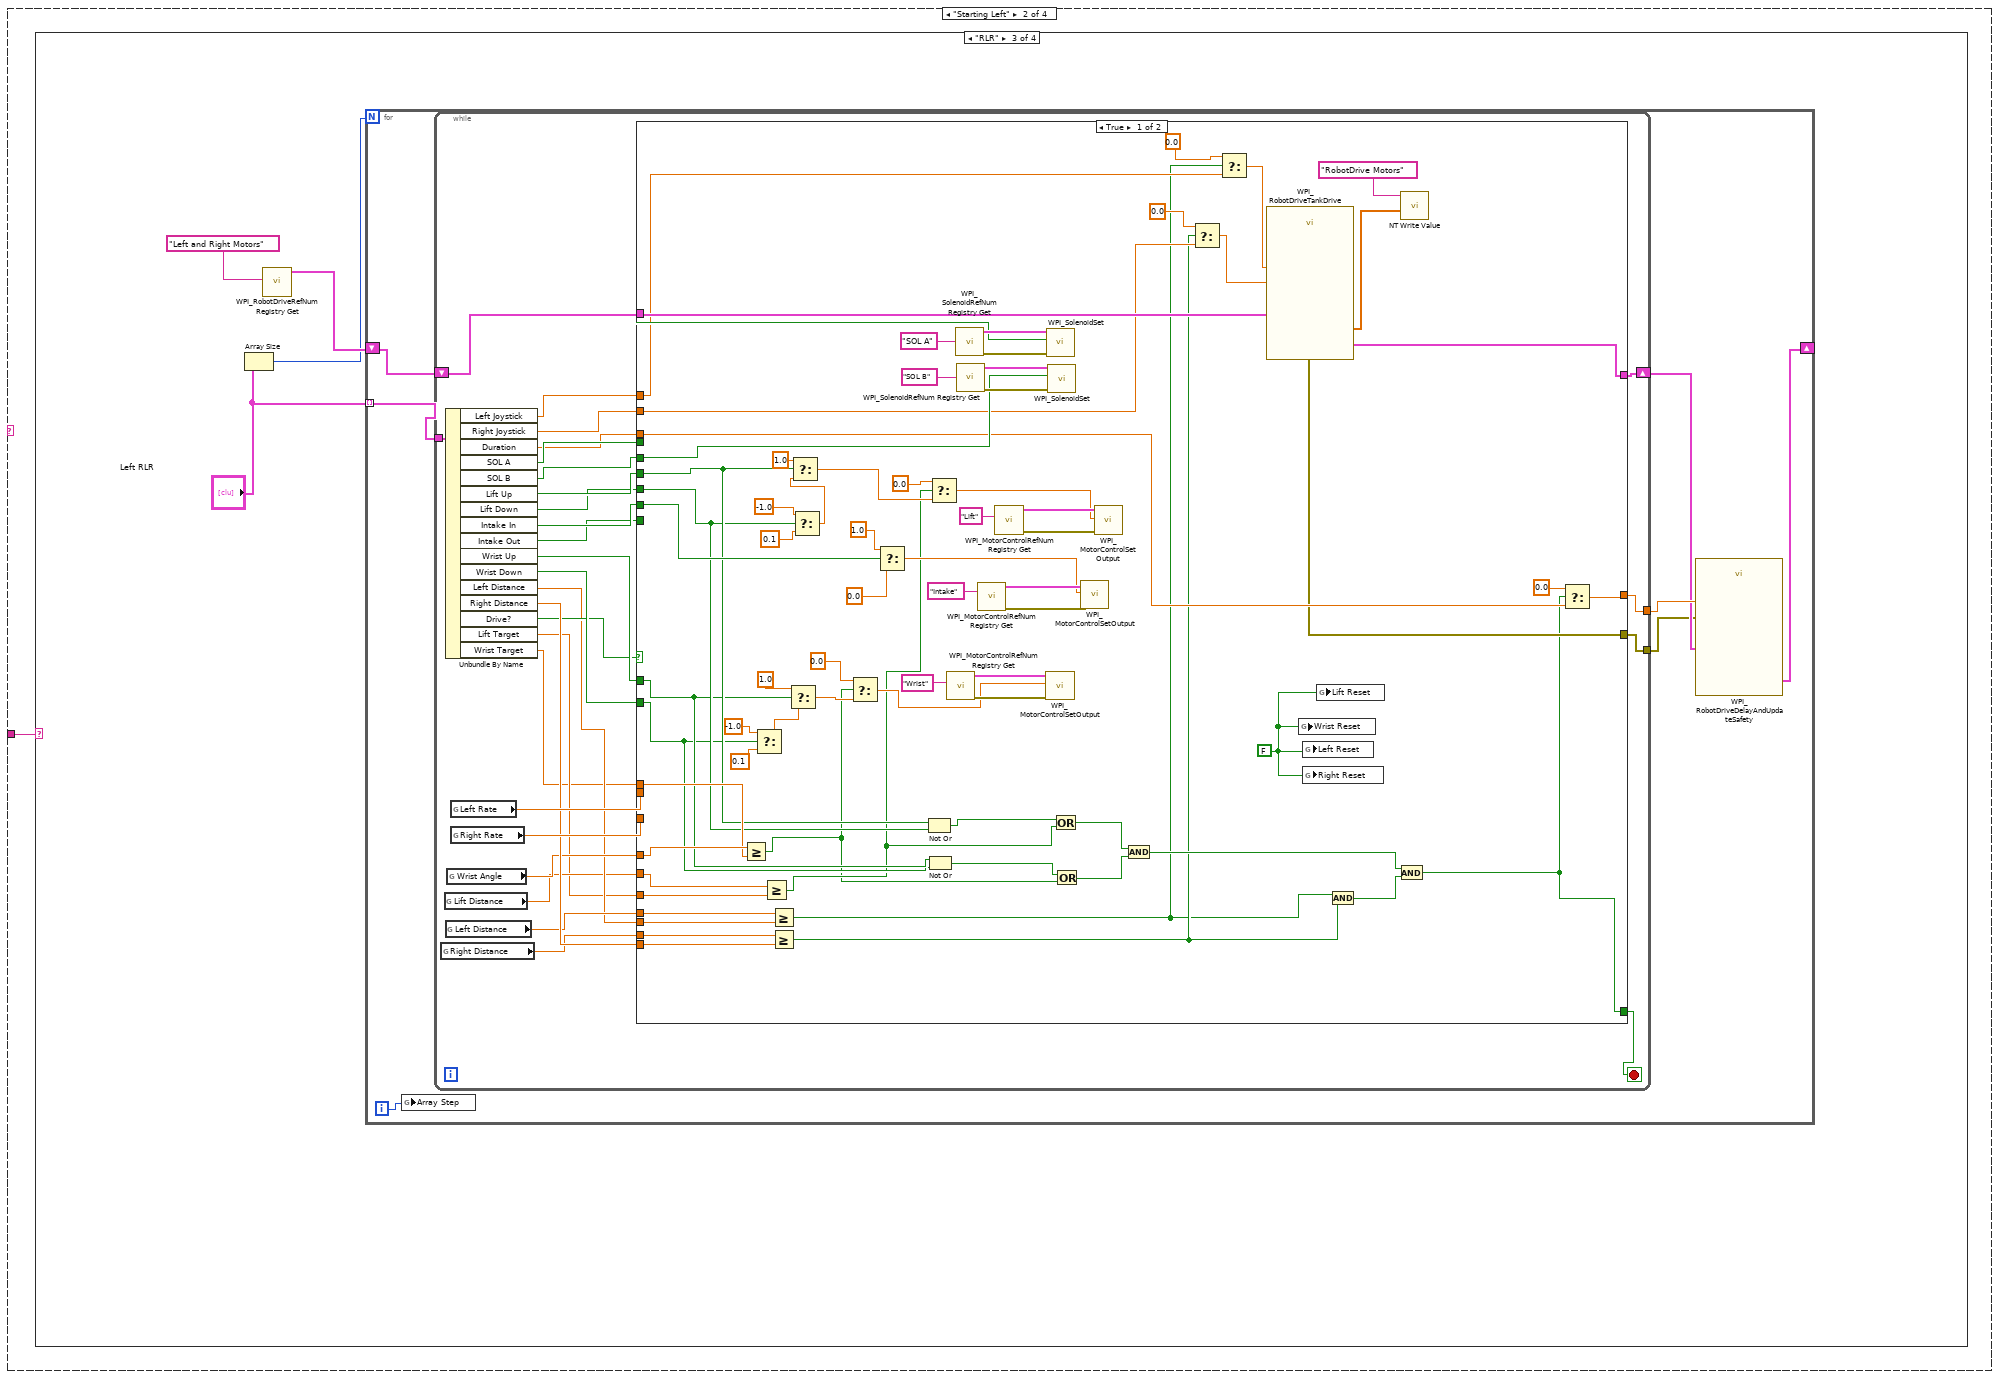
[diagram p4: hidden frame]
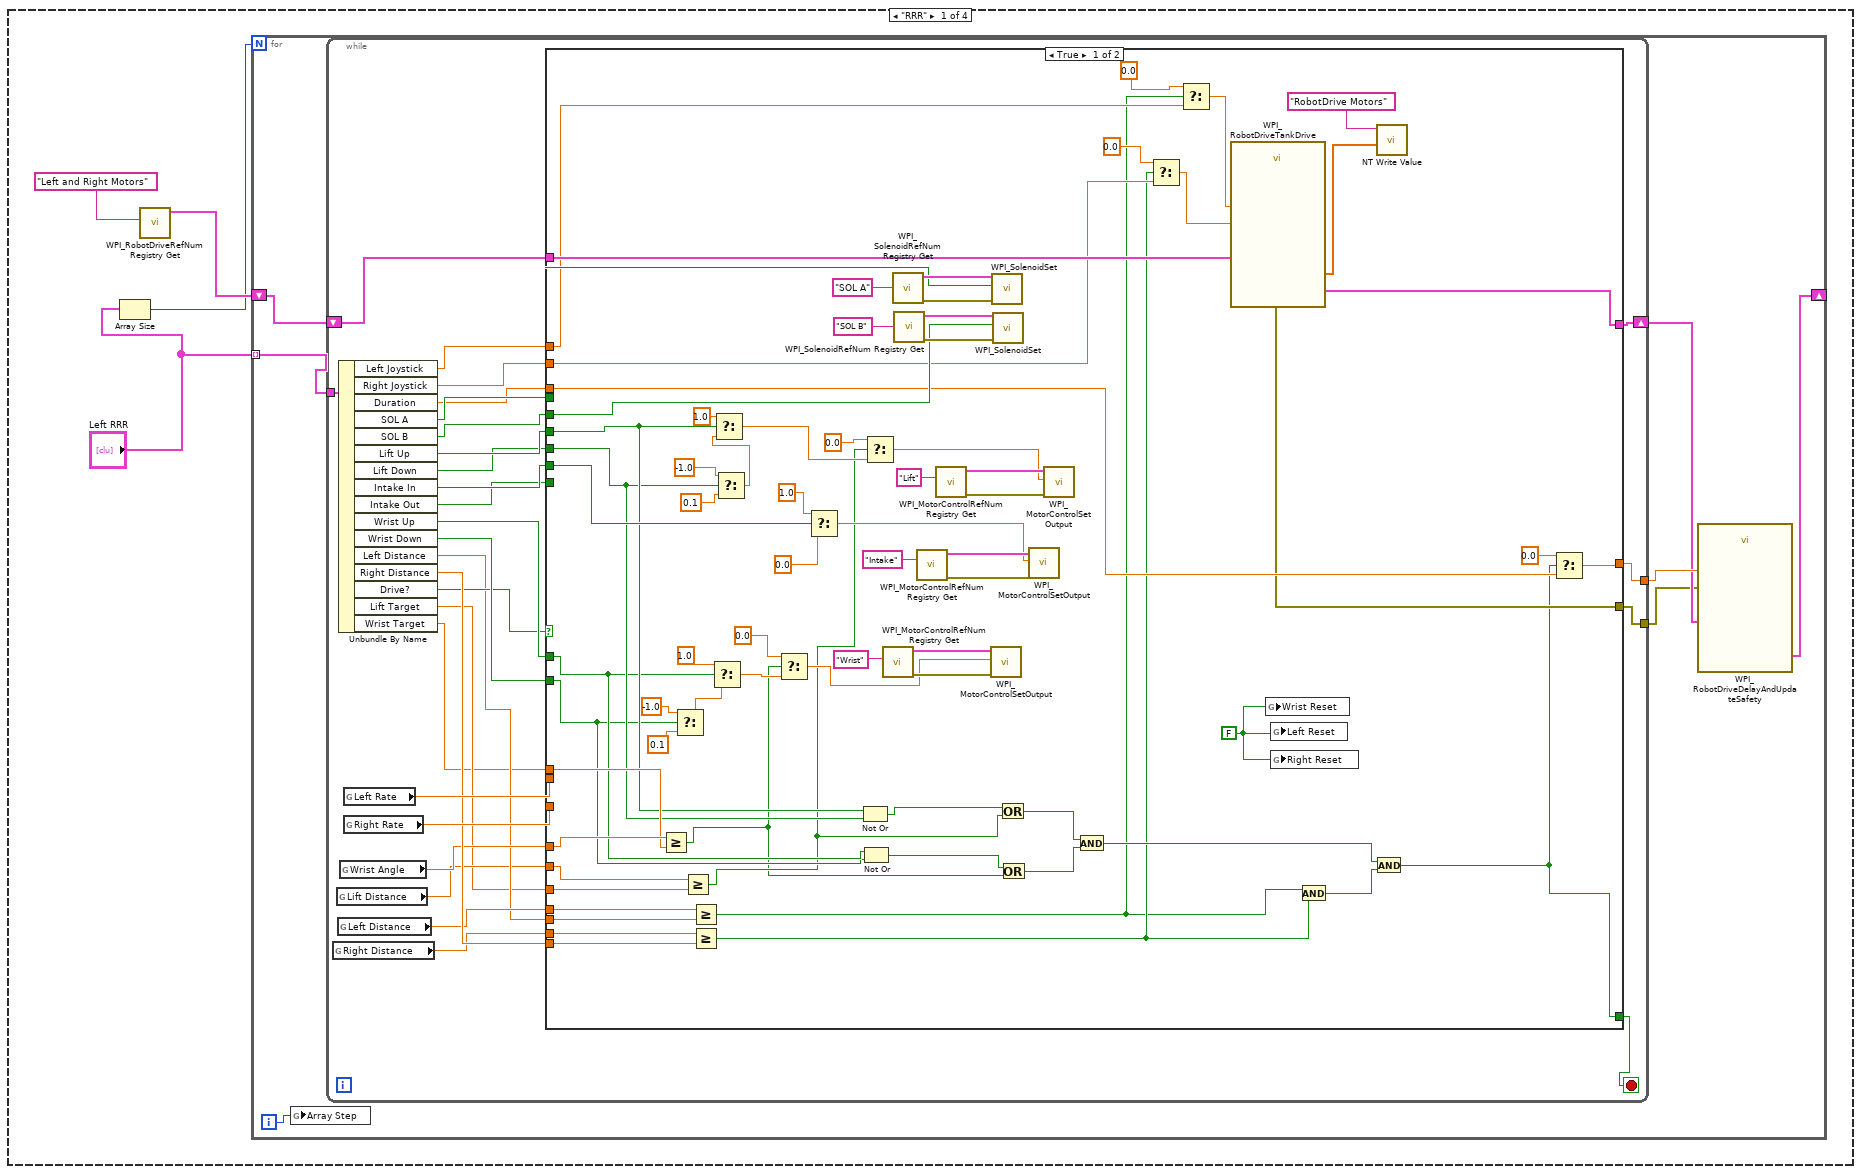
[diagram p5: hidden frame]
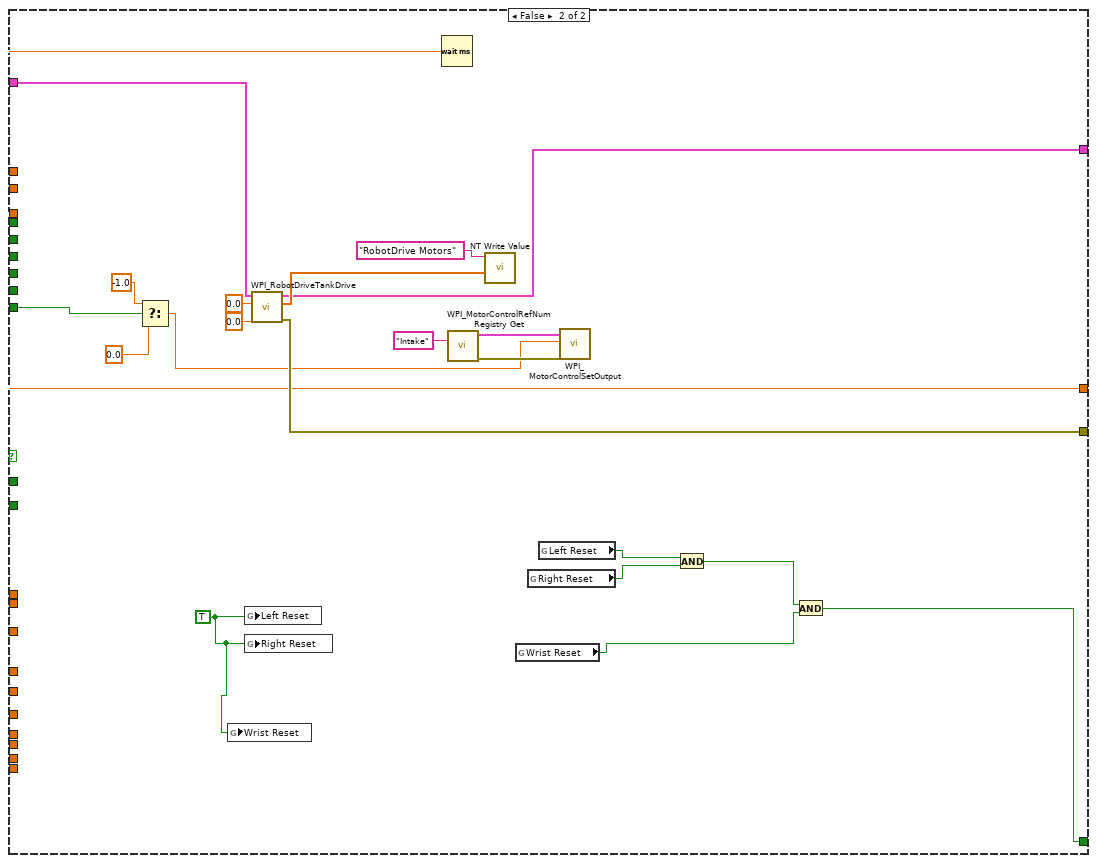
[diagram p6: hidden frame]
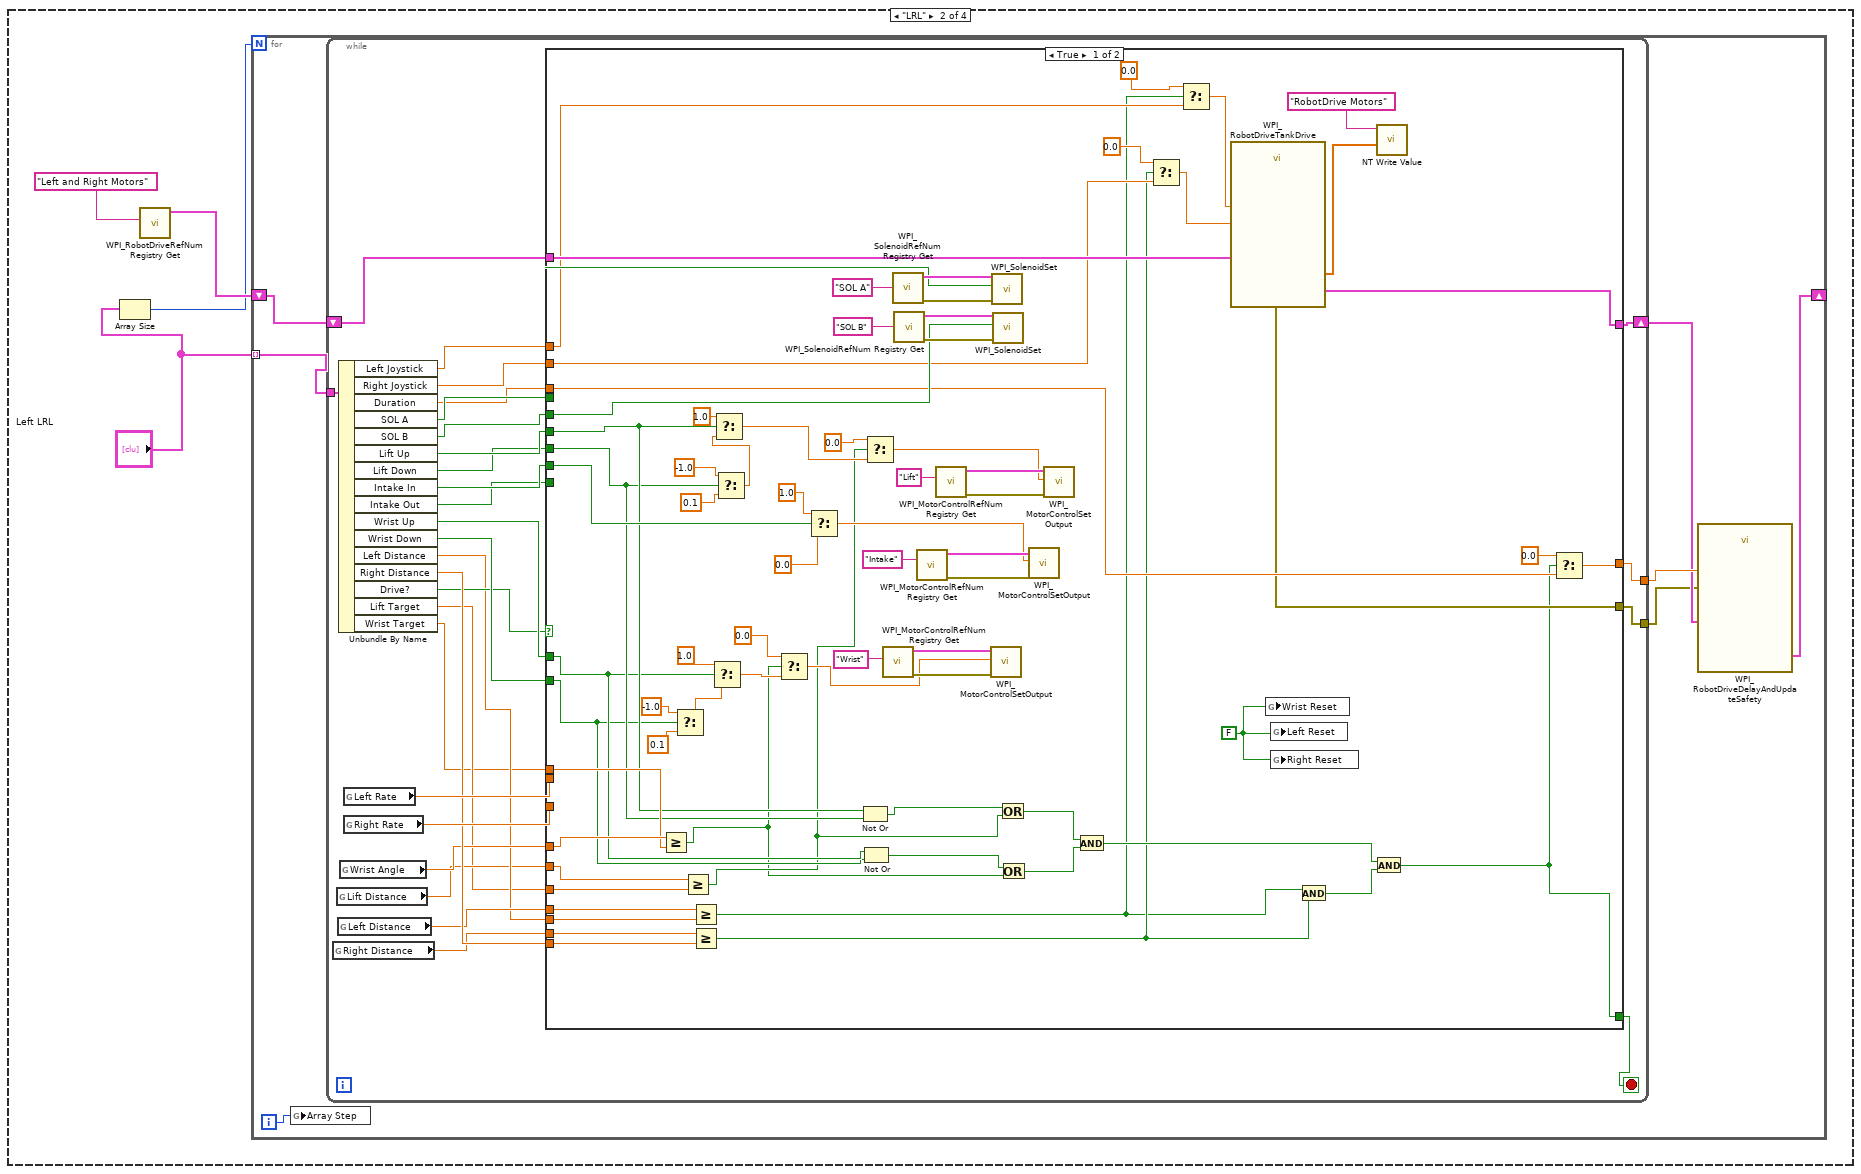
[diagram p7: hidden frame]
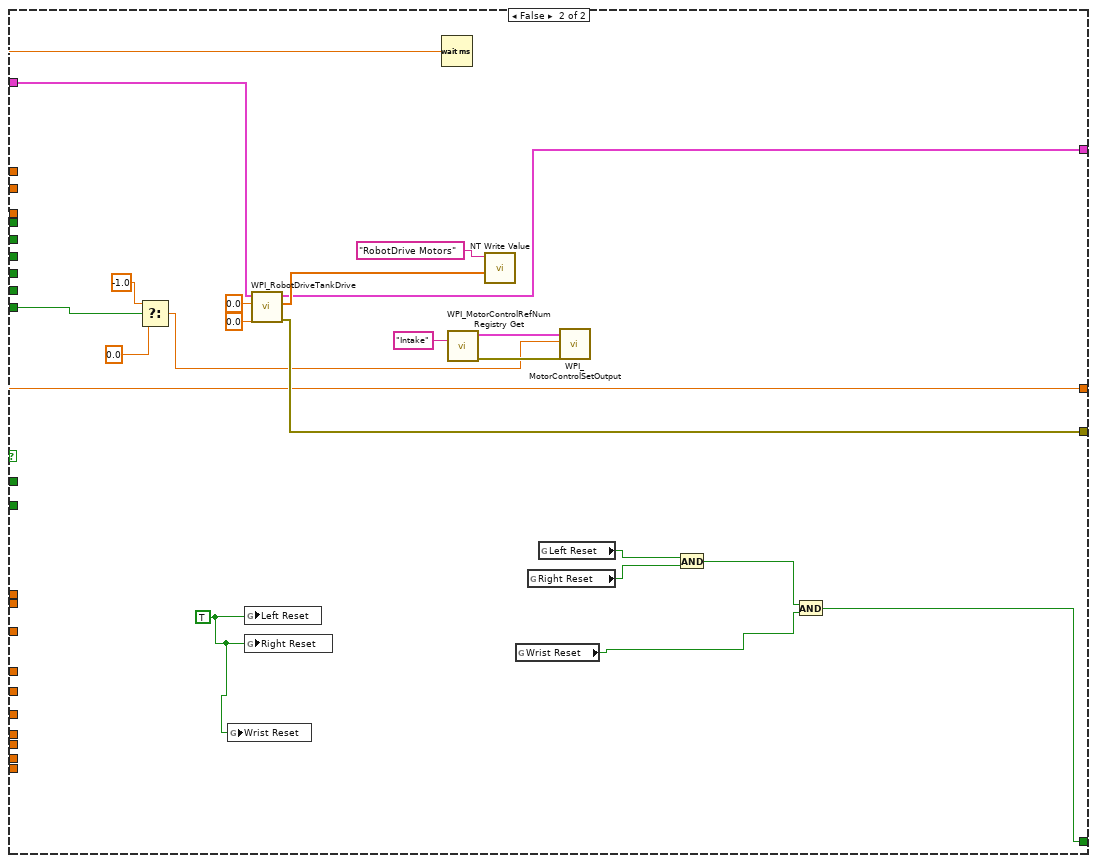
[diagram p8: hidden frame]
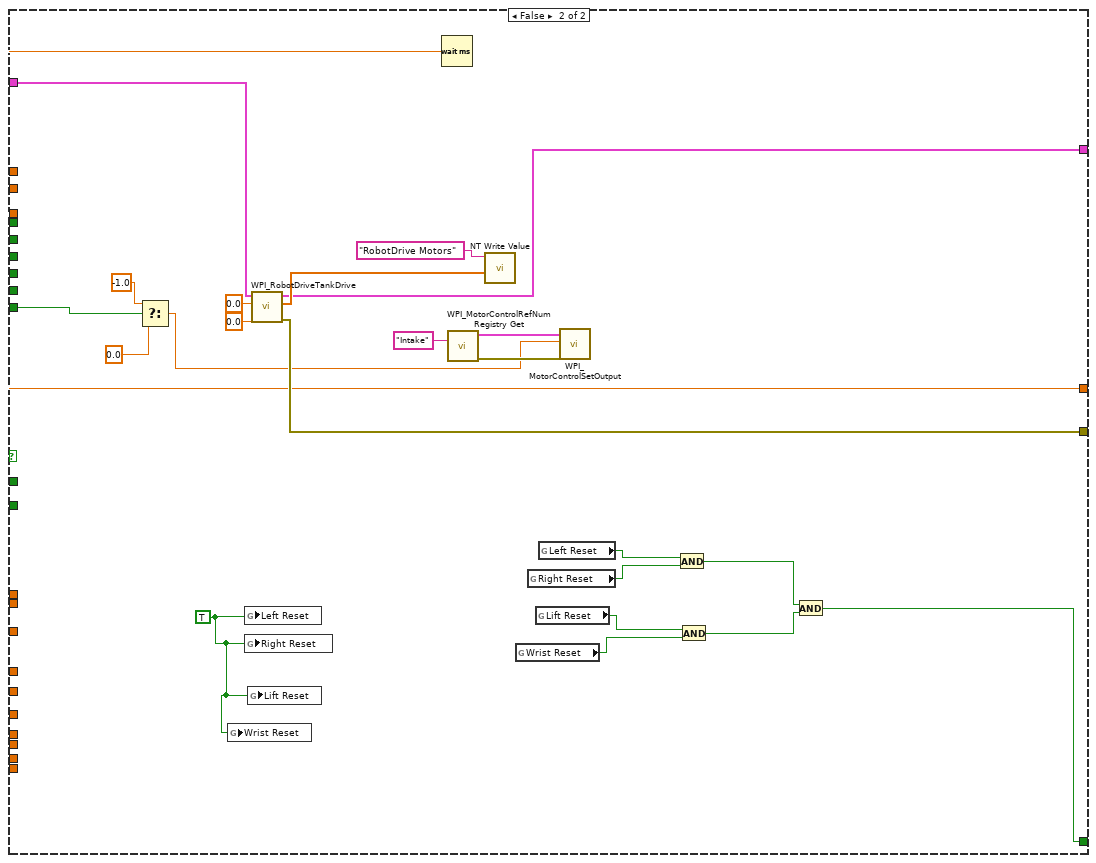
[diagram p9: hidden frame]
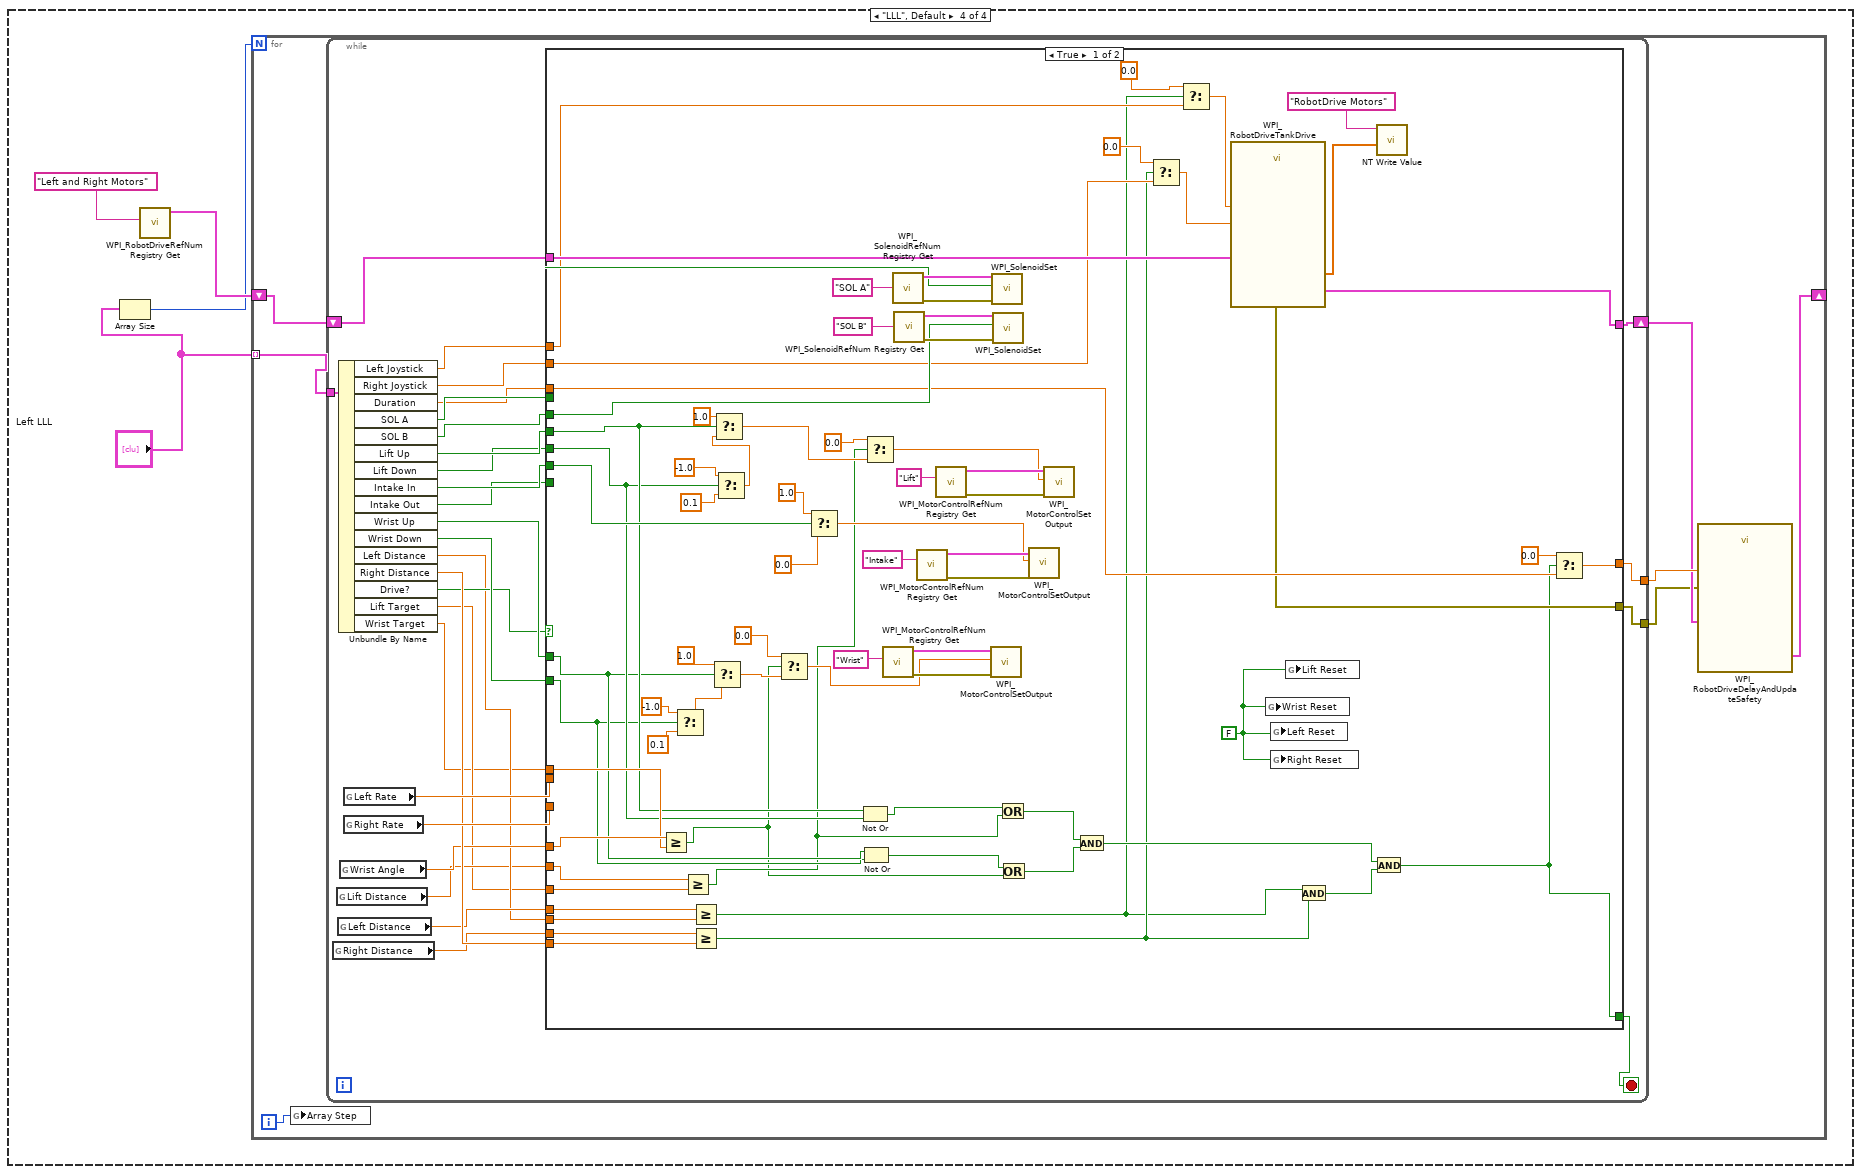
[diagram p10: hidden frame]
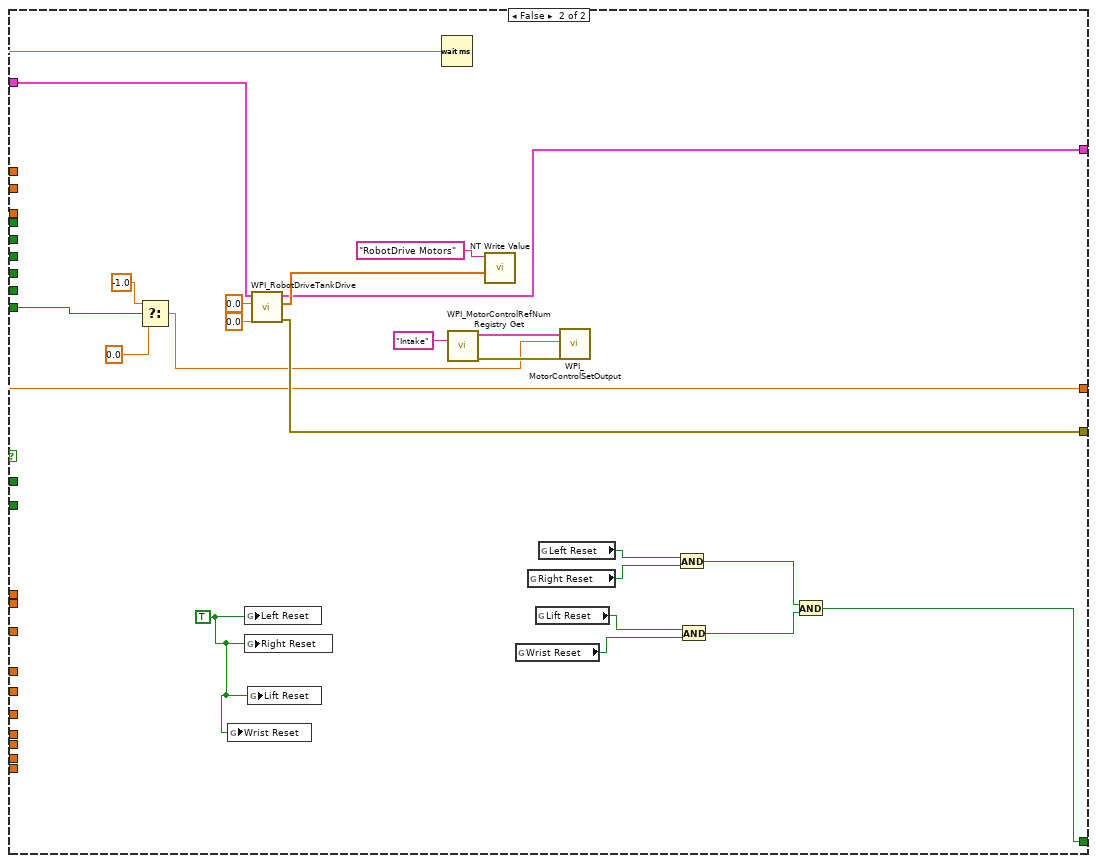
[diagram p11: hidden frame]
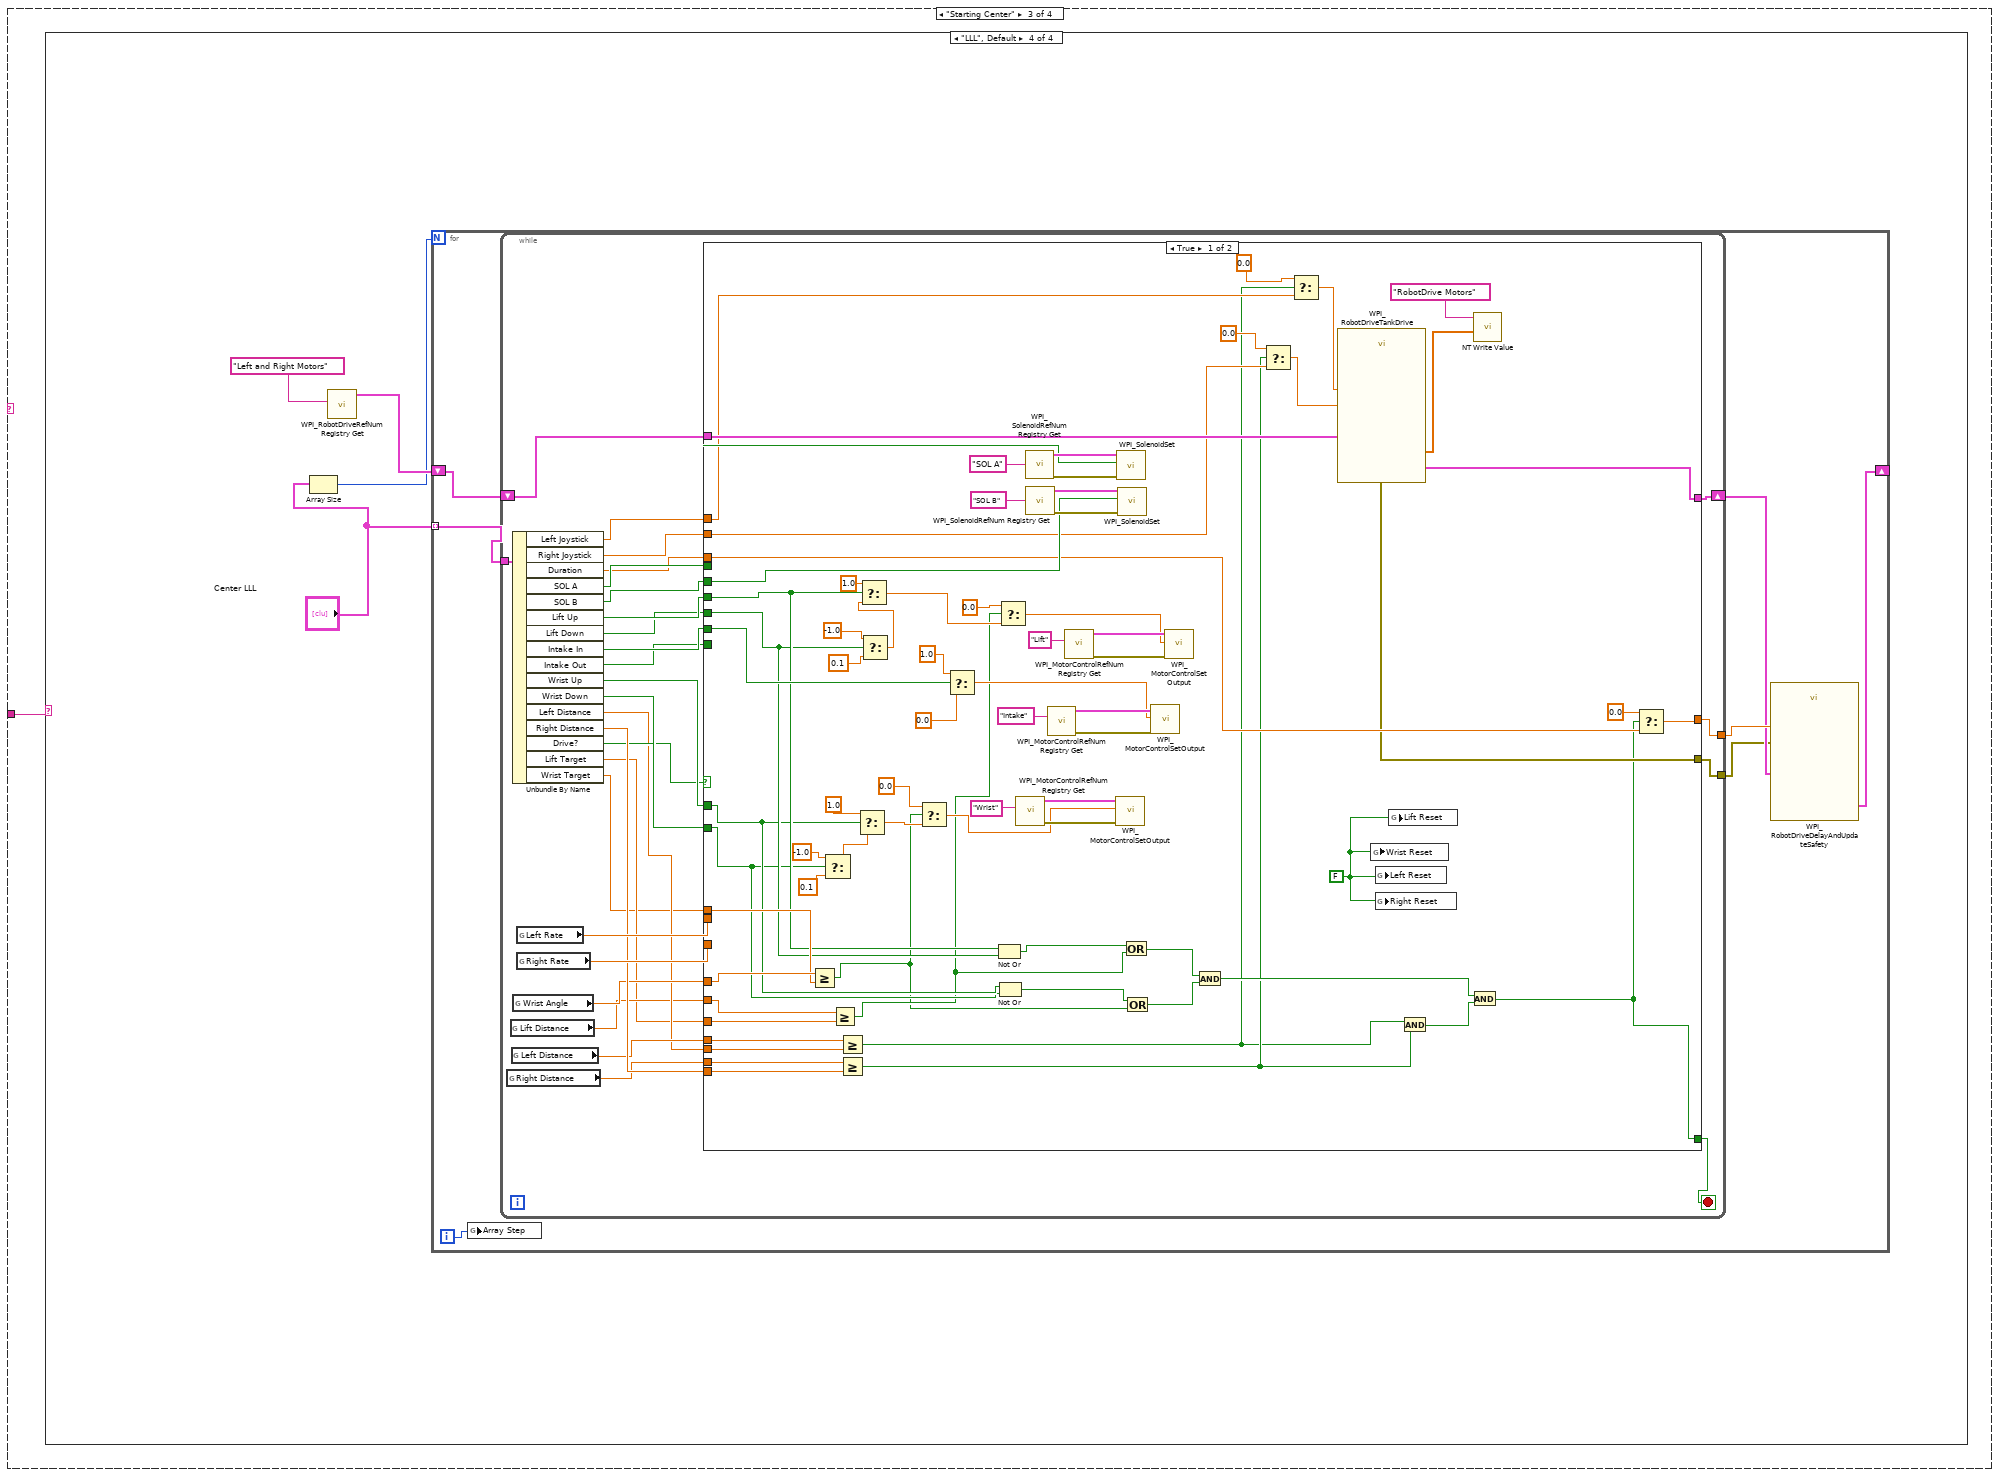
[diagram p12: hidden frame]
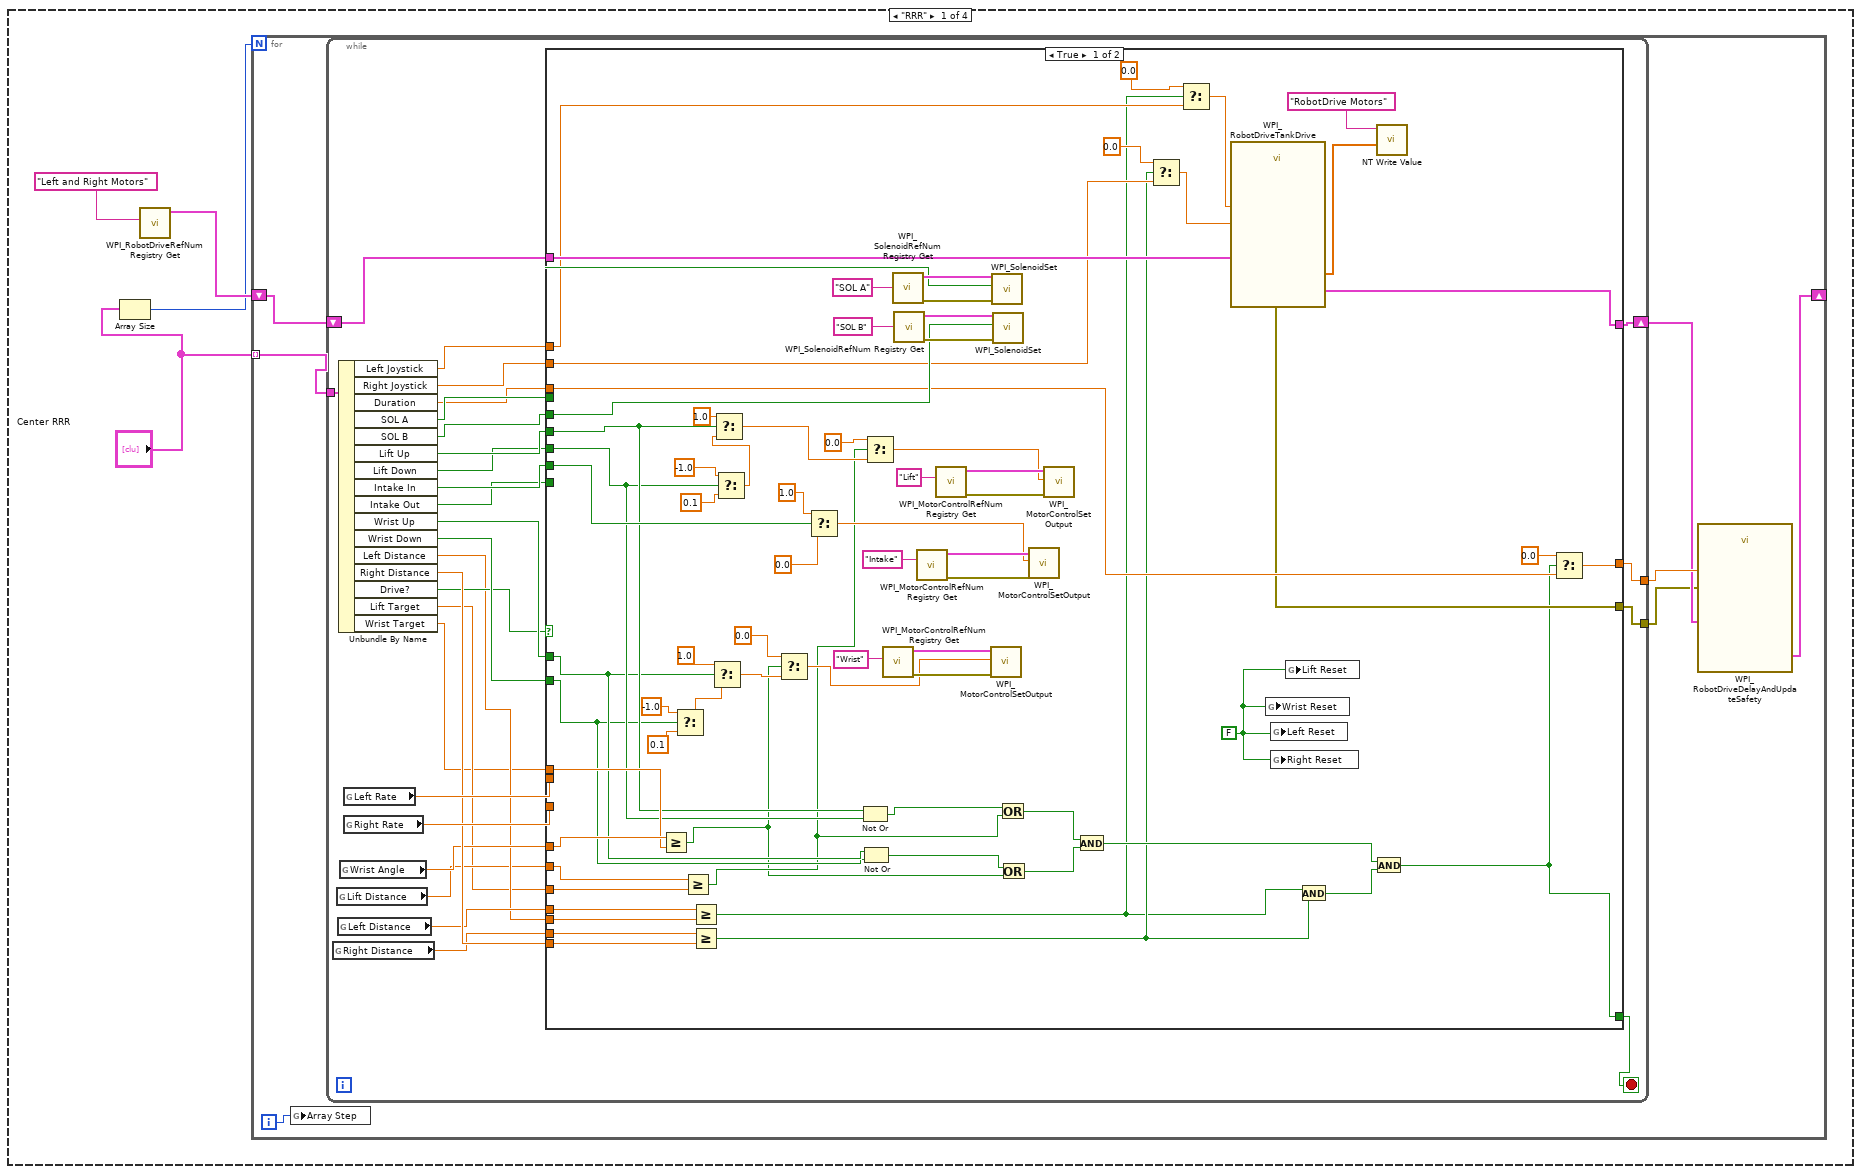
[diagram p13: hidden frame]
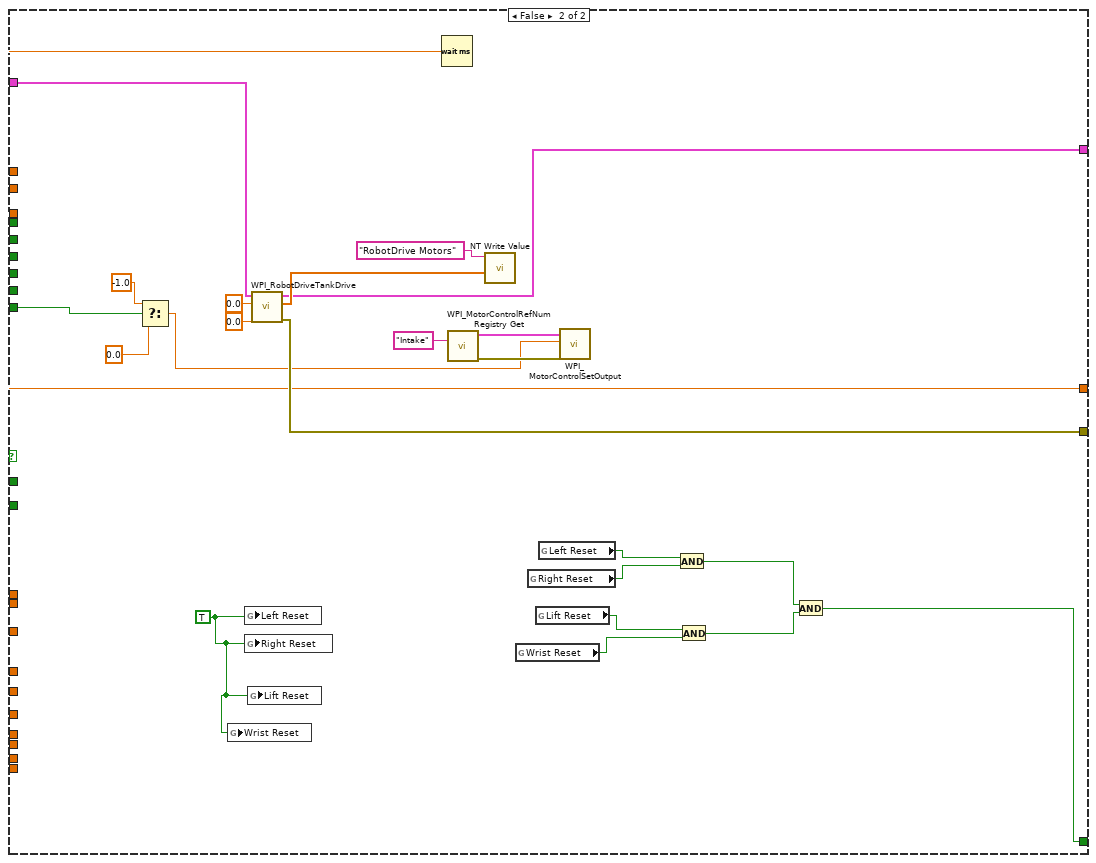
[diagram p14: hidden frame]
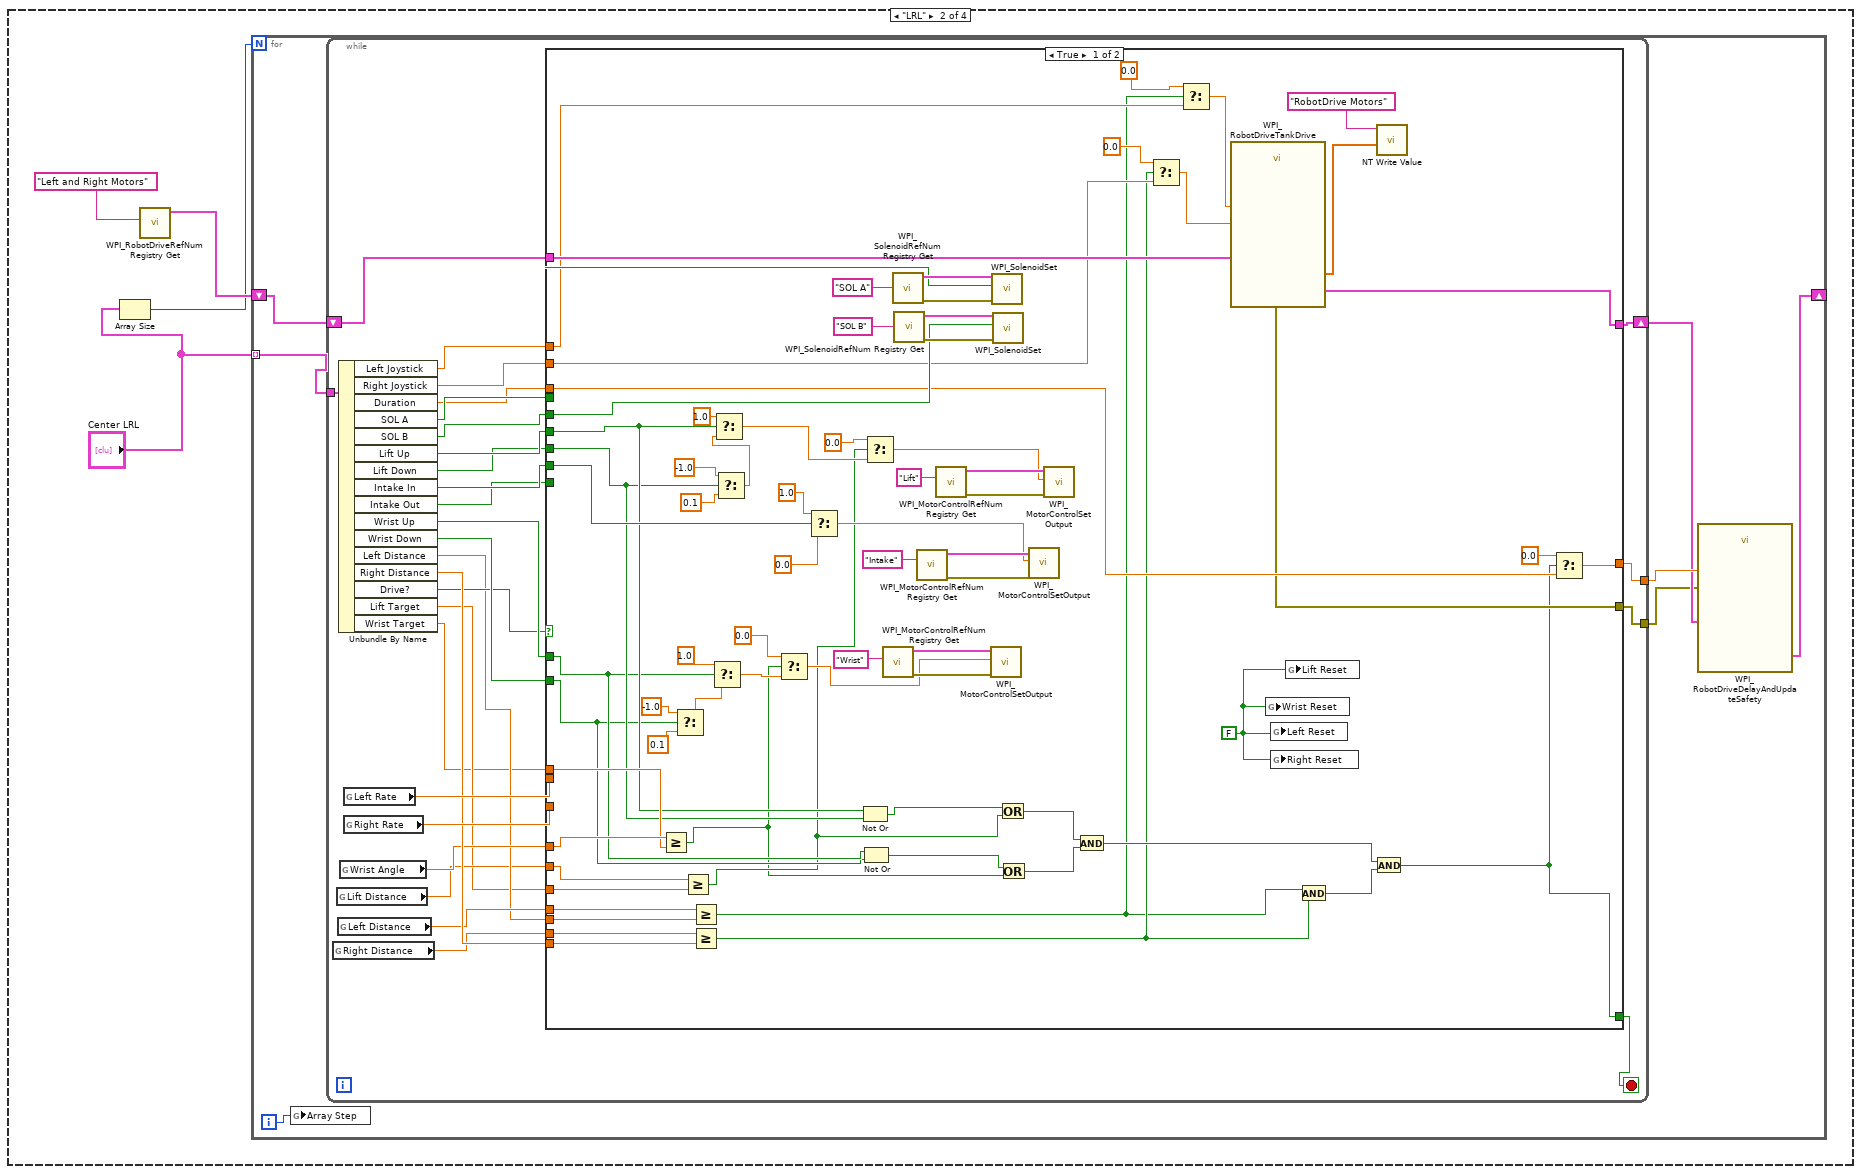
[diagram p15: hidden frame]
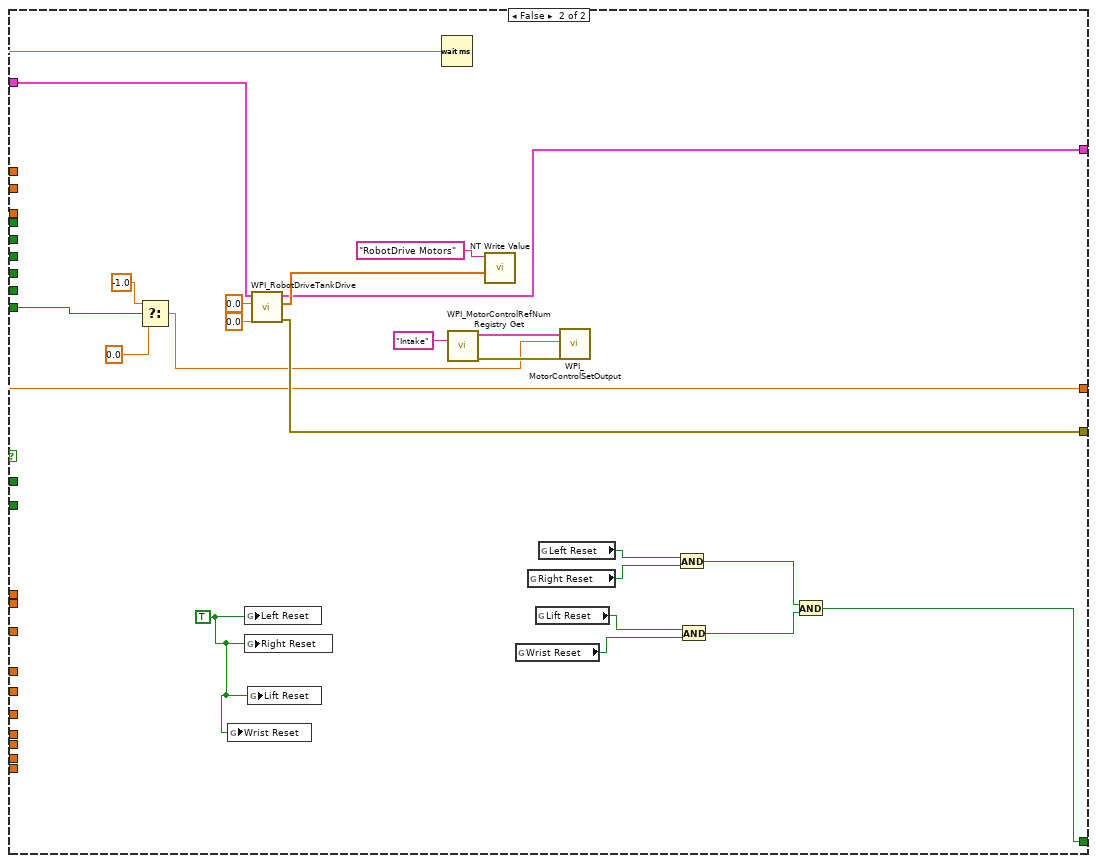
[diagram p16: hidden frame]
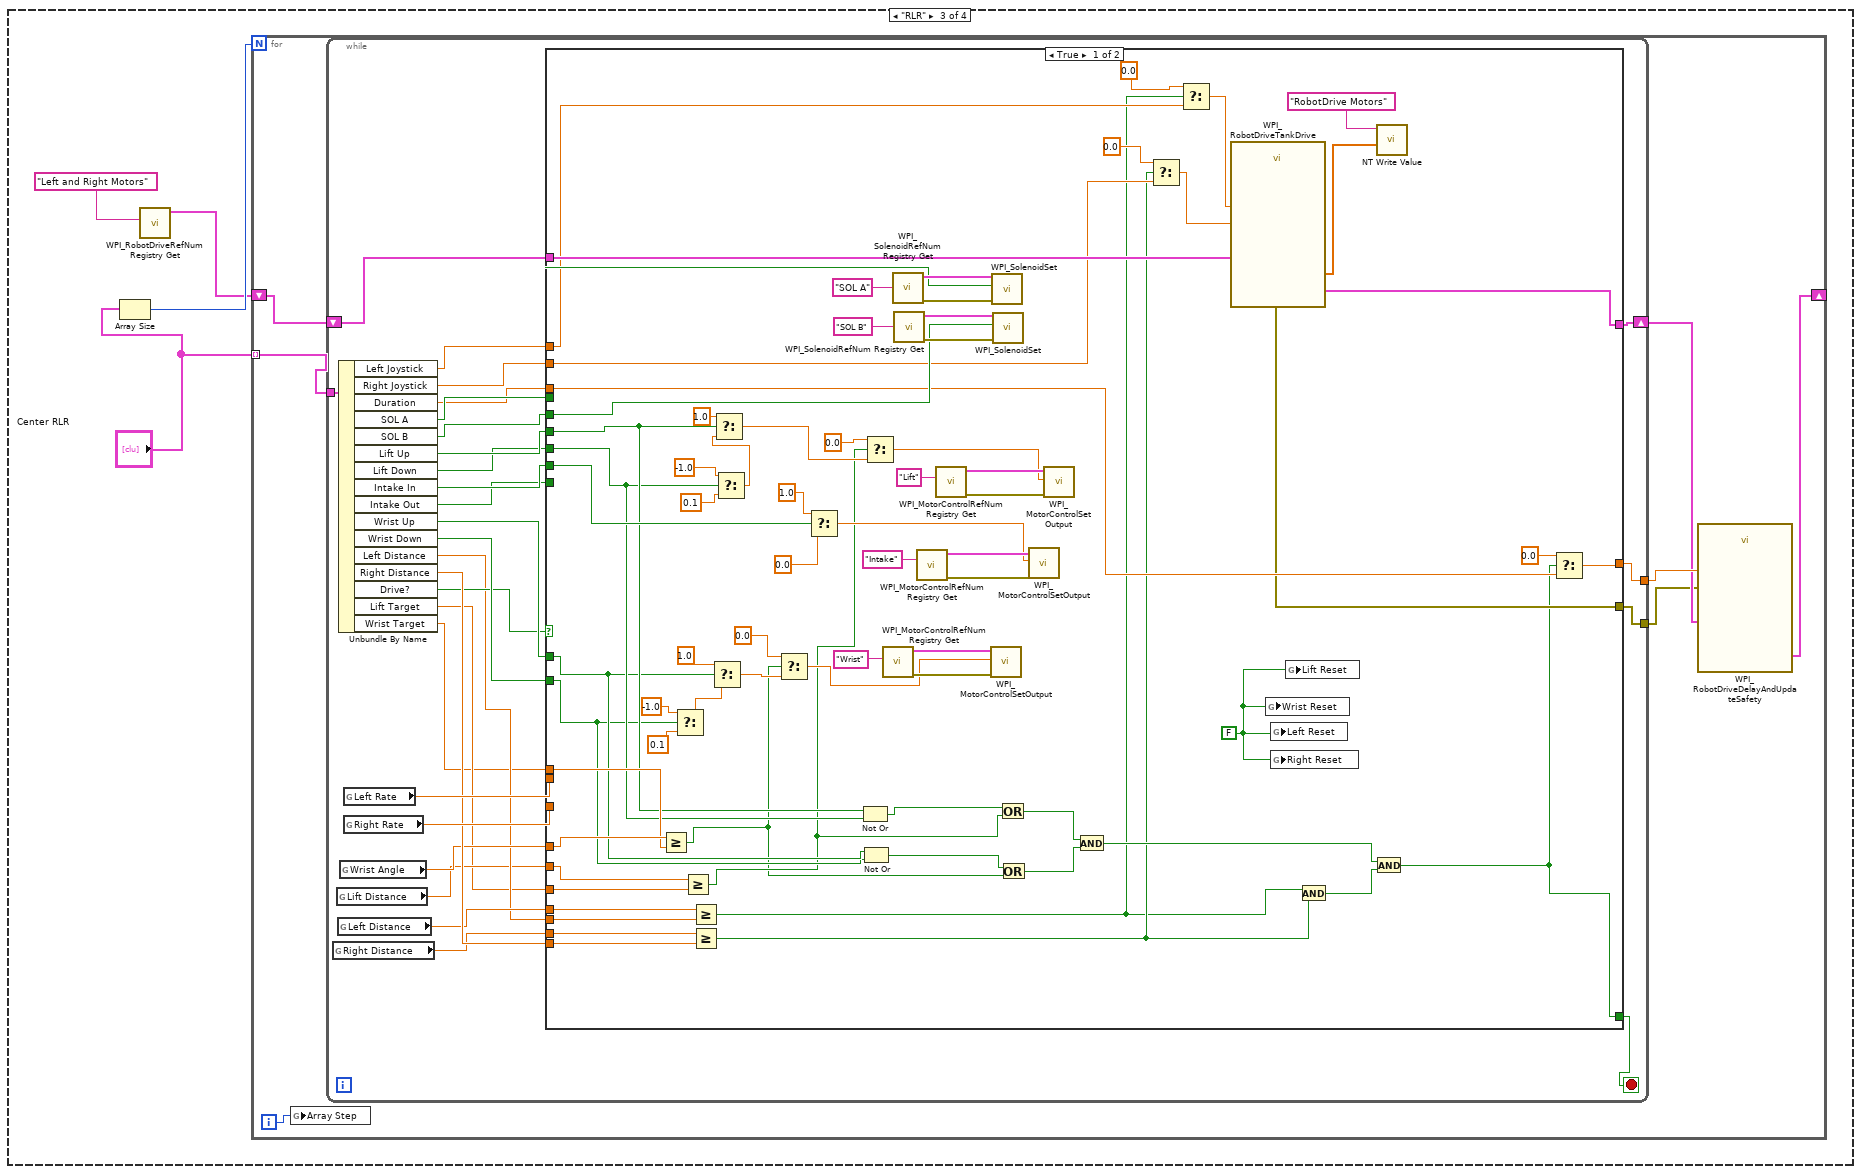
[diagram p17: hidden frame]
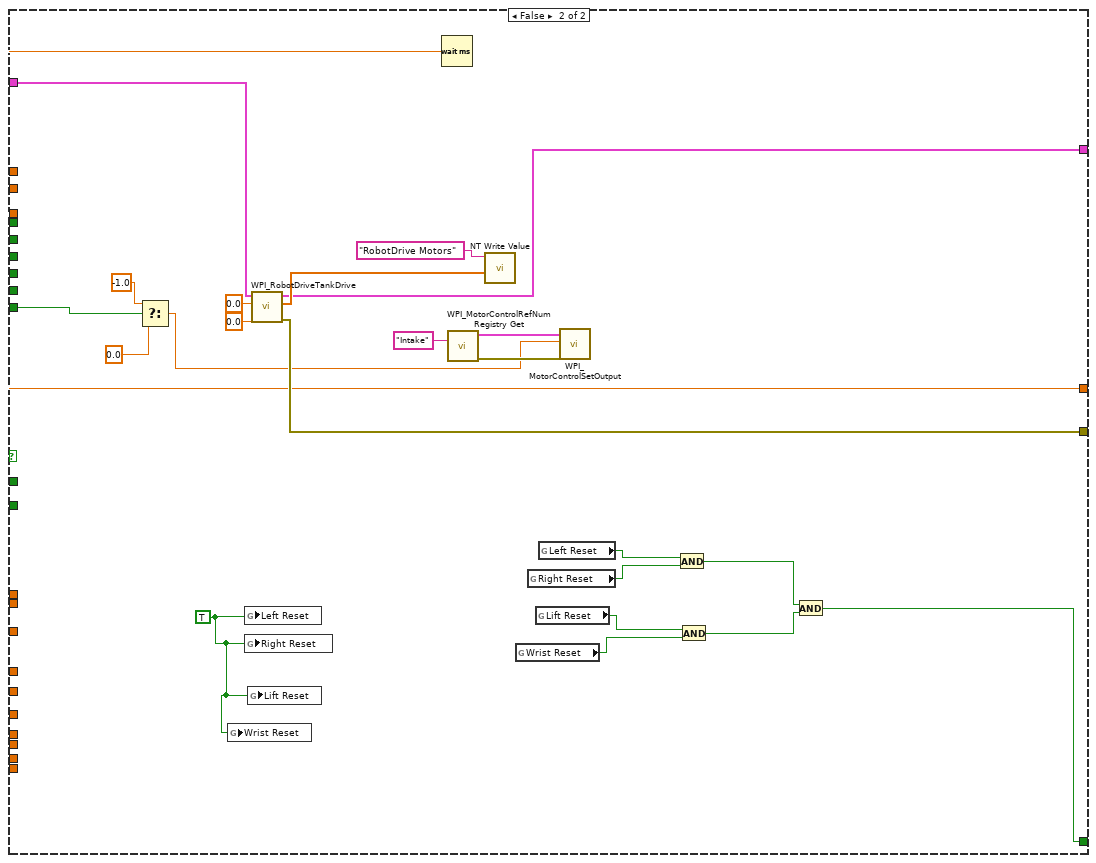
[diagram p18: hidden frame]
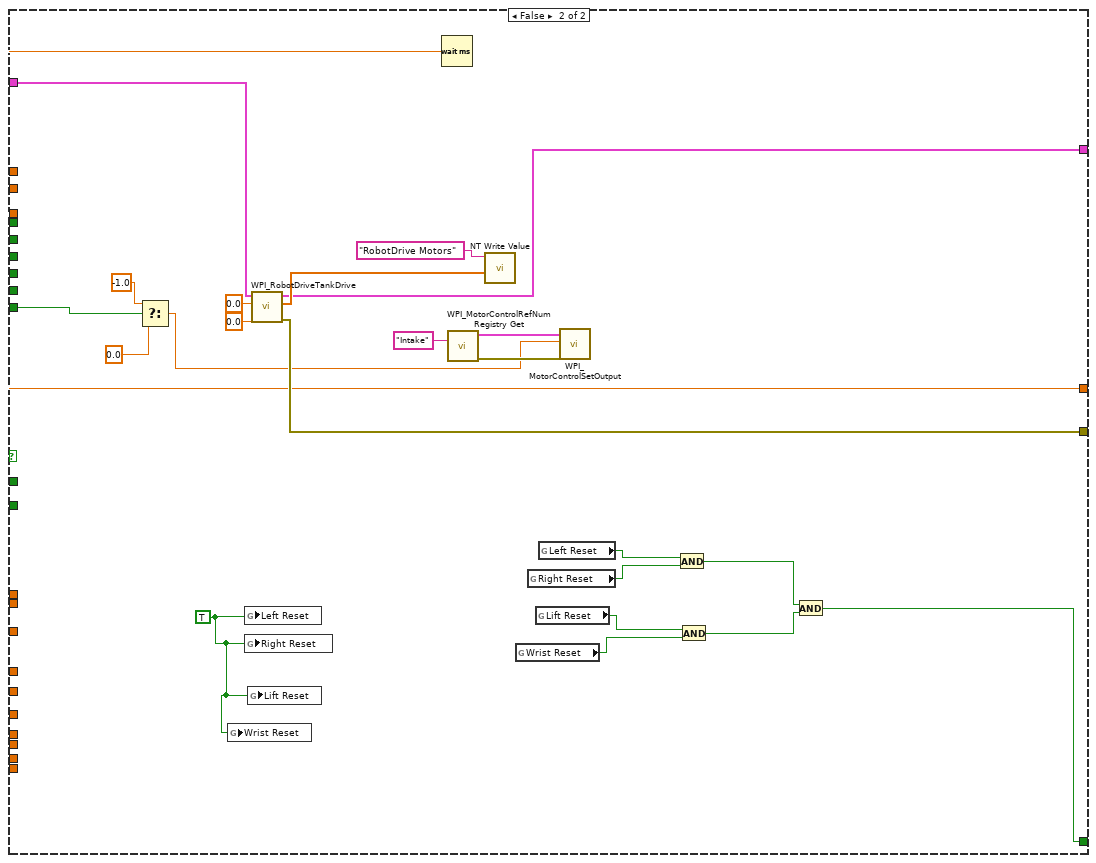
[diagram p19: hidden frame]
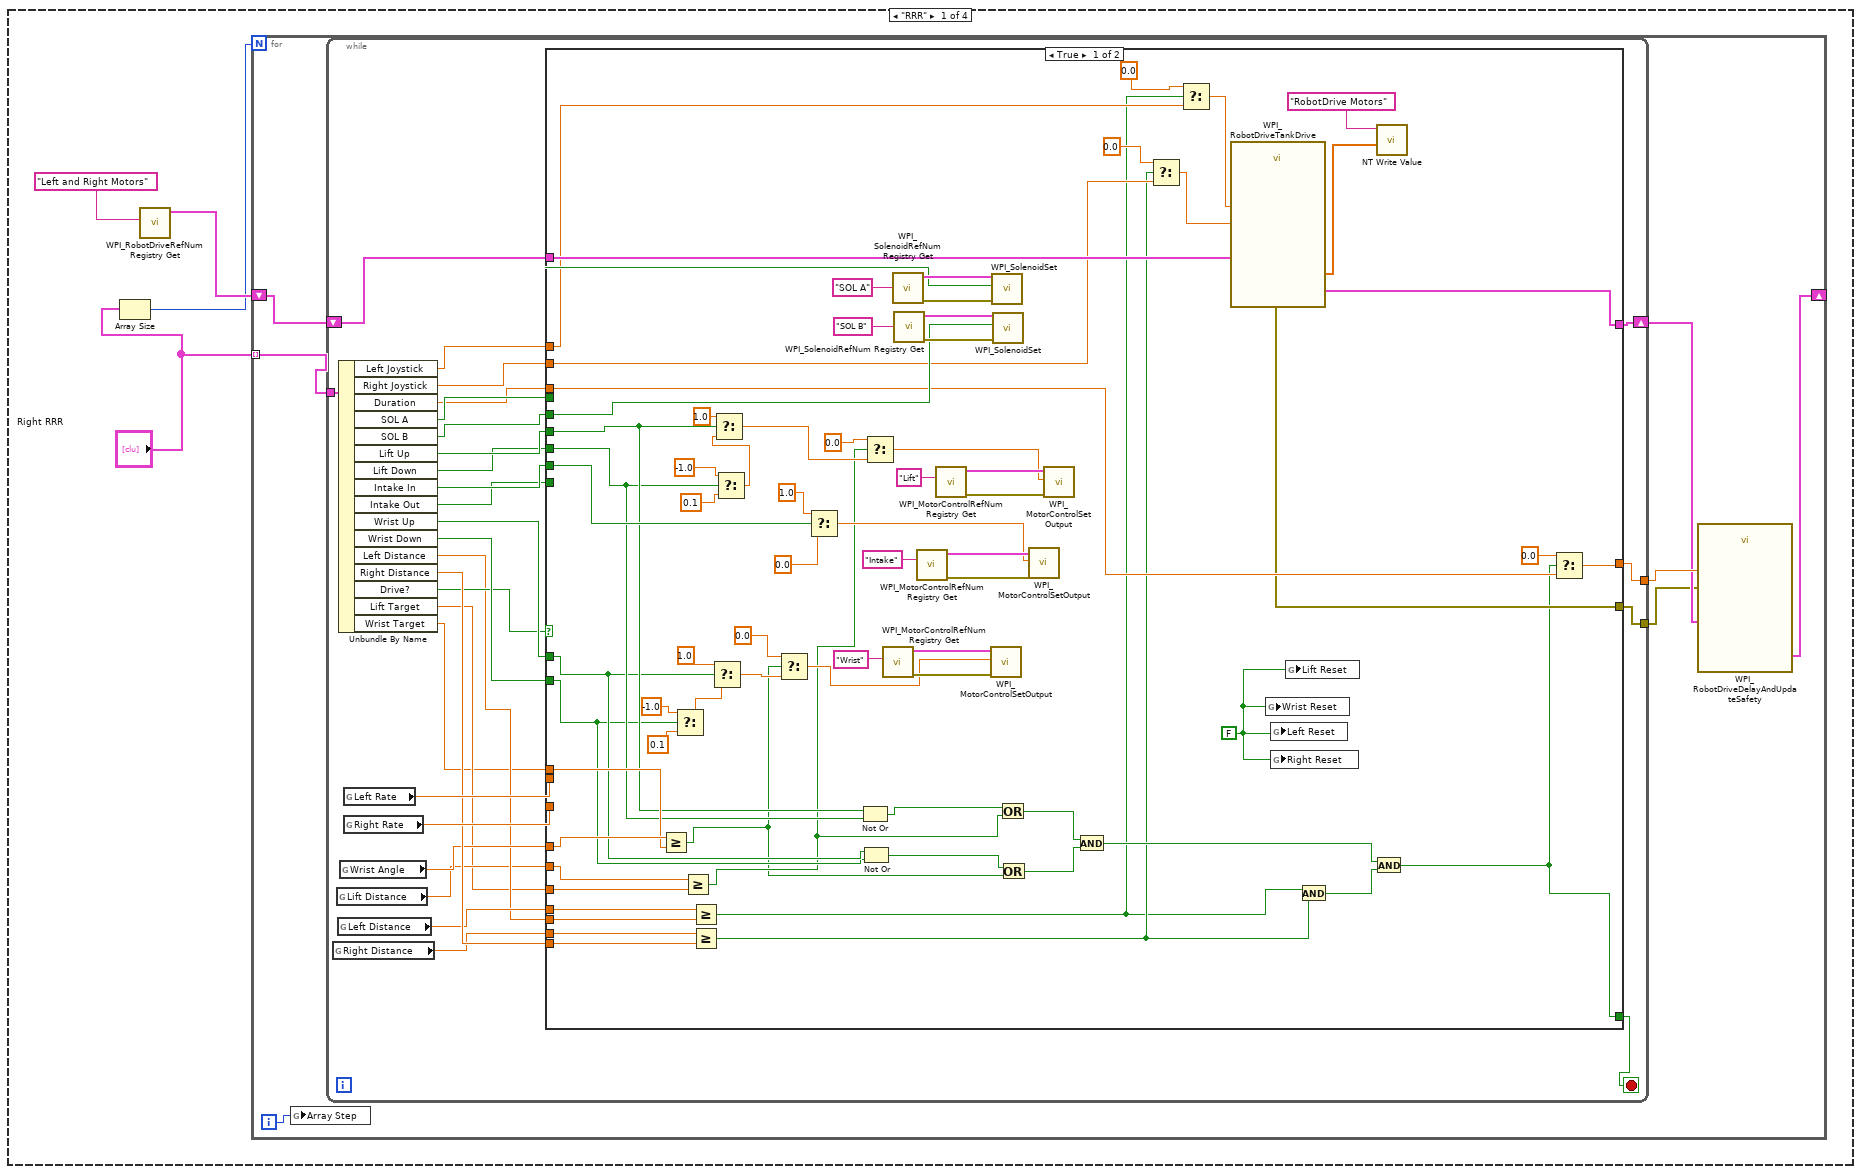
[diagram p20: hidden frame]
diagram:
  (unwired) "This function is run in parallel when the autonomous period begins. It will be terminated automatically when the period ends.\n\nNote that all Driver Station inputs are automatically latched and will not change once auto begins."
  # "This tells you the autonomous selected\nfrom the dashboard"
  # "Every 20ms, report that we are running autonomous\ncode. Loop will abort the same time as the VI."
  # "This gives you the joystick value\nthat is often the throttle"
  # "Use time and/or sensors to control how the robot drives."
  # "This tells you the driver position\nand alliance color"
  n1 = call <vilib>:"WPI_DriverStationGet Alliance Info.vi"() -> ()  [unwired: 12 out]
  n2 = call <vilib>:"WPI_DriverStationGame Specific Data.vi"() -> ("Game Specific Data"=w3:string)  [unwired: 11 in]
  n3 = while {
    stop <- FALSE stop-if-true
    n4 = call <vilib>:"WPI_DriverStationReport Robot Code State.vi"("Autonomous"=TRUE) -> ()  [unwired: 10 in, 1 out]
    n5 = Wait (ms)(milliseconds to wait=u32 20) -> ()  [unwired: 1 out]
  }
  n6 = call <vilib>:"WPI_JoystickRefNum Registry Get.vi"("refnum name"="Left Joystick") -> ("JoystickDevRef"=w14:T2)  [unwired: 1 in, 9 out]
  n7 = call <vilib>:"WPI_JoystickRefNum Registry Get.vi"("refnum name"="Right Joystick") -> ("JoystickDevRef"=w8:T2)  [unwired: 1 in, 9 out]
  n8 = String Subset(string=w3, length (rest)=1 ("length (rest)")) -> (substring=w1:string)  [unwired: 1 in]
  n9 = call <vilib>:"WPI_JoystickGetValues.vi"("JoystickDevRef"=w14) -> ("Axes"=w7:dbl[])  [unwired: 6 in, 4 out]
  n10 = call <vilib>:"WPI_JoystickGetValues.vi"("JoystickDevRef"=w8) -> ("Axes"=w4:dbl[])  [unwired: 6 in, 4 out]
  n11 = call-poly <vilib>:"NT Read Value.vi"("Name"="Auto Selector") -> ("String"=w11:string)  [unwired: 9 in, 1 out]
  n12 = Index Array(array=w4, index=2) -> ()  [unwired: 1 out]
  n13 = call-poly <vilib>:"NT Write Value.vi"("Numeric Array"=w7, "Name"="Left Joystick/Axes") -> ()  [unwired: 9 in, 1 out]
  n14 = Index Array(array=w7, index=2) -> ()  [unwired: 1 out]
  n15 = call-poly <vilib>:"NT Write Value.vi"("Numeric Array"=w4, "Name"="Right Joystick/Axes") -> ()  [unwired: 9 in, 1 out]
  n16 = case shown="\"Starting Right\"" w11 {
    tunnel: w1 -> [_ w152 w689 w1230]
    frame Default {
      n17 = Array Size(array="Testing") -> (size(s)=w20:i32)
      n18 = call <vilib>:"WPI_RobotDriveRefNum Registry Get.vi"("refnum name"="Left and Right Motors") -> ("RobotDriveDevRef"=w21:T4)  [unwired: 1 in, 9 out]
      n19 = for {
        N: w20 -> [_]
        shift-right: [w29] -> _
        shift-left: w21 -> [w28]
        tunnel: "Testing" -> [w27] mode=indexing
        i -> [w23]
        n20 = global write "Robot Global Data.vi" "Array Step"(w23) -> ()
        n21 = while {
          shift-right: [w57] -> w25
          shift-left: w28 -> [w56]
          tunnel: w27 -> [w53]
          tunnel: [w34] -> w26
          tunnel: [w37] -> w24
          stop <- w38 stop-if-true
          n22 = global read "Robot Global Data.vi" "Right Distance"() -> (w41:dbl)
          n23 = global read "Robot Global Data.vi" "Lift Distance"() -> (w32:dbl)
          n24 = global read "Robot Global Data.vi" "Left Distance"() -> (w40:dbl)
          n25 = Unbundle By Name(w53) -> ("Left Joystick"=w52:dbl, "Right Joystick"=w51:dbl, "Duration"=w39:dbl, "SOL A"=w50:bool, "SOL B"=w49:bool, "Lift Up"=w48:bool, "Lift Down"=w47:bool, "Intake In"=w46:bool, "Intake Out"=w45:bool, "Wrist Up"=w44:bool, "Wrist Down"=w43:bool, "Left Distance"=w33:dbl, "Right Distance"=w42:dbl, "Drive?"=w36:bool, "Lift Target"=w31:dbl, "Wrist Target"=w30:dbl)
          n26 = global read "Robot Global Data.vi" "Wrist Angle"() -> (w35:dbl)
          n27 = global read "Robot Global Data.vi" "Left Rate"() -> (w55:dbl)
          n28 = global read "Robot Global Data.vi" "Right Rate"() -> (w54:dbl)
          n29 = case shown="True" w36 {
            tunnel: [w130 w146] -> w57
            tunnel: w56 -> [w129 w147]
            tunnel: w55 -> [_ _]
            tunnel: w54 -> [_ _]
            tunnel: w52 -> [w87 _]
            tunnel: w51 -> [w88 _]
            tunnel: w50 -> [w112 _]
            tunnel: w49 -> [w111 _]
            tunnel: w48 -> [w70 _]
            tunnel: w47 -> [w69 _]
            tunnel: w46 -> [w92 _]
            tunnel: w45 -> [_ w137]
            tunnel: w44 -> [w68 _]
            tunnel: w43 -> [w67 _]
            tunnel: w33 -> [w91 _]
            tunnel: w42 -> [w110 _]
            tunnel: w41 -> [w109 _]
            tunnel: w40 -> [w108 _]
            tunnel: w39 -> [w106 w135]
            tunnel: [w89 w135] -> w34
            tunnel: [w74 w133] -> w38
            tunnel: [w105 w145] -> w37
            tunnel: w35 -> [w81 _]
            tunnel: w32 -> [w82 _]
            tunnel: w31 -> [w86 _]
            tunnel: w30 -> [w80 _]
            frame True {
              w73 = FALSE ("Left Reset")
              n30 = Greater Or Equal?(x=w81, y=w80) -> (x >= y?=w63:bool)
              n31 = Select(t=-1.0, s=w67, f=0.1) -> (s? t:f=w95:dbl)
              n32 = Greater Or Equal?(x=w82, y=w86) -> (x >= y?=w65:bool)
              n33 = Greater Or Equal?(x=w108, y=w91) -> (x >= y?=w58:bool)
              n34 = Greater Or Equal?(x=w109, y=w110) -> (x >= y?=w59:bool)
              n35 = Select(t=1.0, s=w68, f=w95) -> (s? t:f=w78:dbl)
              n36 = Select(t=-1.0, s=w69, f=0.1) -> (s? t:f=w94:dbl)
              n37 = Select(t=1.0, s=w70, f=w94) -> (s? t:f=w84:dbl)
              n38 = Select(t=0.0, s=w63, f=w78) -> (s? t:f=w77:dbl)
              n39 = Select(t=1.0, s=w92, f=0.0) -> (s? t:f=w93:dbl)
              n40 = Not Or(1:w69, 2:w70) -> (0:w66:bool)
              n41 = Not Or(1:w67, 2:w68) -> (0:w64:bool)
              n42 = Select(t=0.0, s=w65, f=w84) -> (s? t:f=w83:dbl)
              n43 = call <vilib>:"WPI_MotorControlRefNum Registry Get.vi"("refnum name"="Wrist") -> ("error out"=w116:errorcluster, "MotorControlDevRef"=w117:T5)  [unwired: 9 in]
              n44 = call <vilib>:"WPI_SolenoidRefNum Registry Get.vi"("refnum name"="SOL A") -> ("error out"=w125:errorcluster, "SolenoidDevRef"=w126:T10)  [unwired: 9 in]
              n45 = call <vilib>:"WPI_SolenoidRefNum Registry Get.vi"("refnum name"="SOL B") -> ("error out"=w122:errorcluster, "SolenoidDevRef"=w123:T10)  [unwired: 9 in]
              n46 = call <vilib>:"WPI_MotorControlRefNum Registry Get.vi"("refnum name"="Intake") -> ("error out"=w118:errorcluster, "MotorControlDevRef"=w119:T5)  [unwired: 9 in]
              n47 = call <vilib>:"WPI_MotorControlRefNum Registry Get.vi"("refnum name"="Lift") -> ("error out"=w120:errorcluster, "MotorControlDevRef"=w121:T5)  [unwired: 9 in]
              n48 = call <vilib>:"WPI_MotorControlSetOutput.vi"("error in (no error)"=w116, "Output"=w77, "MotorControlDevRef"=w117) -> ()  [unwired: 6 in, 3 out]
              n49 = call-poly <vilib>:"WPI_SolenoidSet.vi"("error in (no error)"=w125, "Value"=w112, "SolenoidDevRef"=w126) -> ()  [unwired: 7 in, 2 out]
              n50 = call-poly <vilib>:"WPI_SolenoidSet.vi"("error in (no error)"=w122, "Value"=w111, "SolenoidDevRef"=w123) -> ()  [unwired: 7 in, 2 out]
              n51 = Or(x=w66, y=w65) -> (x .or. y?=w62:bool)
              n52 = Or(x=w64, y=w63) -> (x .or. y?=w61:bool)
              n53 = call <vilib>:"WPI_MotorControlSetOutput.vi"("error in (no error)"=w118, "Output"=w93, "MotorControlDevRef"=w119) -> ()  [unwired: 6 in, 3 out]
              n54 = call <vilib>:"WPI_MotorControlSetOutput.vi"("error in (no error)"=w120, "Output"=w83, "MotorControlDevRef"=w121) -> ()  [unwired: 6 in, 3 out]
              n55 = And(x=w62, y=w61) -> (x .and. y?=w60:bool)
              n56 = Select(t=0.0, s=w59, f=w88) -> (s? t:f=w71:dbl)
              n57 = Select(t=0.0, s=w58, f=w87) -> (s? t:f=w72:dbl)
              n58 = call <vilib>:"WPI_RobotDriveTankDrive.vi"("Right axis value"=w71, "Left axis value"=w72, "RobotDriveDevRef"=w129) -> ("error out"=w105:errorcluster, "Motor Values"=w90:dbl[], "RobotDriveDevRef"=w130:T4)  [unwired: 6 in]
              n59 = global write "Robot Global Data.vi" "Wrist Reset"(w73) -> ()
              n60 = global write "Robot Global Data.vi" "Left Reset"(w73) -> ()
              n61 = global write "Robot Global Data.vi" "Right Reset"(w73) -> ()
              n62 = And(x=w58, y=w59) -> (x .and. y?=w75:bool)
              n63 = And(x=w60, y=w75) -> (x .and. y?=w74:bool)
              n64 = call-poly <vilib>:"NT Write Value.vi"("Numeric Array"=w90, "Name"="RobotDrive Motors") -> ()  [unwired: 9 in, 1 out]
              n65 = Select(t=0.0, s=w74, f=w106) -> (s? t:f=w89:dbl)
            }
            frame False {
              w132 = TRUE ("Left Reset")
              n66 = Select(t=-1.0, s=w137, f=0.0) -> (s? t:f=w136:dbl)
              n67 = global write "Robot Global Data.vi" "Wrist Reset"(w132) -> ()
              n68 = global write "Robot Global Data.vi" "Left Reset"(w132) -> ()
              n69 = global write "Robot Global Data.vi" "Right Reset"(w132) -> ()
              n70 = call <vilib>:"WPI_RobotDriveTankDrive.vi"("Right axis value"=0.0, "Left axis value"=0.0, "RobotDriveDevRef"=w147) -> ("error out"=w145:errorcluster, "Motor Values"=w150:dbl[], "RobotDriveDevRef"=w146:T4)  [unwired: 6 in]
              n71 = Wait (ms)(milliseconds to wait=w135) -> ()  [unwired: 1 out]
              n72 = call <vilib>:"WPI_MotorControlRefNum Registry Get.vi"("refnum name"="Intake") -> ("error out"=w141:errorcluster, "MotorControlDevRef"=w142:T5)  [unwired: 9 in]
              n73 = call-poly <vilib>:"NT Write Value.vi"("Numeric Array"=w150, "Name"="RobotDrive Motors") -> ()  [unwired: 9 in, 1 out]
              n74 = global read "Robot Global Data.vi" "Wrist Reset"() -> (w131:bool)
              n75 = global read "Robot Global Data.vi" "Right Reset"() -> (w143:bool)
              n76 = global read "Robot Global Data.vi" "Left Reset"() -> (w144:bool)
              n77 = call <vilib>:"WPI_MotorControlSetOutput.vi"("error in (no error)"=w141, "Output"=w136, "MotorControlDevRef"=w142) -> ()  [unwired: 6 in, 3 out]
              n78 = And(x=w144, y=w143) -> (x .and. y?=w134:bool)
              n79 = And(x=w134, y=w131) -> (x .and. y?=w133:bool)
            }
          }
        }
        n80 = call <vilib>:"WPI_RobotDriveDelayAndUpdateSafety.vi"("error in (no error)"=w24, "Delay (s)"=w26, "RobotDriveDevRef"=w25) -> ("RobotDriveDevRef 2"=w29:T4)  [unwired: 7 in, 1 out]
      }
    }
    frame "Starting Left" {
      n81 = case shown="\"RLR\"" w152 {
        frame "RRR" {
          n82 = Array Size(array="Left RRR") -> (size(s)=w154:i32)
          n83 = call <vilib>:"WPI_RobotDriveRefNum Registry Get.vi"("refnum name"="Left and Right Motors") -> ("RobotDriveDevRef"=w155:T4)  [unwired: 1 in, 9 out]
          n84 = for {
            N: w154 -> [_]
            shift-right: [w163] -> _
            shift-left: w155 -> [w162]
            tunnel: "Left RRR" -> [w161] mode=indexing
            i -> [w157]
            n85 = global write "Robot Global Data.vi" "Array Step"(w157) -> ()
            n86 = while {
              shift-right: [w191] -> w159
              shift-left: w162 -> [w190]
              tunnel: w161 -> [w187]
              tunnel: [w168] -> w160
              tunnel: [w171] -> w158
              stop <- w172 stop-if-true
              n87 = global read "Robot Global Data.vi" "Right Distance"() -> (w175:dbl)
              n88 = global read "Robot Global Data.vi" "Lift Distance"() -> (w166:dbl)
              n89 = global read "Robot Global Data.vi" "Left Distance"() -> (w174:dbl)
              n90 = Unbundle By Name(w187) -> ("Left Joystick"=w186:dbl, "Right Joystick"=w185:dbl, "Duration"=w173:dbl, "SOL A"=w184:bool, "SOL B"=w183:bool, "Lift Up"=w182:bool, "Lift Down"=w181:bool, "Intake In"=w180:bool, "Intake Out"=w179:bool, "Wrist Up"=w178:bool, "Wrist Down"=w177:bool, "Left Distance"=w167:dbl, "Right Distance"=w176:dbl, "Drive?"=w170:bool, "Lift Target"=w165:dbl, "Wrist Target"=w164:dbl)
              n91 = global read "Robot Global Data.vi" "Wrist Angle"() -> (w169:dbl)
              n92 = global read "Robot Global Data.vi" "Left Rate"() -> (w189:dbl)
              n93 = global read "Robot Global Data.vi" "Right Rate"() -> (w188:dbl)
              n94 = case shown="True" w170 {
                tunnel: [w264 w280] -> w191
                tunnel: w190 -> [w263 w281]
                tunnel: w189 -> [_ _]
                tunnel: w188 -> [_ _]
                tunnel: w186 -> [w221 _]
                tunnel: w185 -> [w222 _]
                tunnel: w184 -> [w246 _]
                tunnel: w183 -> [w245 _]
                tunnel: w182 -> [w204 _]
                tunnel: w181 -> [w203 _]
                tunnel: w180 -> [w226 _]
                tunnel: w179 -> [_ w271]
                tunnel: w178 -> [w202 _]
                tunnel: w177 -> [w201 _]
                tunnel: w167 -> [w225 _]
                tunnel: w176 -> [w244 _]
                tunnel: w175 -> [w243 _]
                tunnel: w174 -> [w242 _]
                tunnel: w173 -> [w240 w269]
                tunnel: [w223 w269] -> w168
                tunnel: [w208 w267] -> w172
                tunnel: [w239 w279] -> w171
                tunnel: w169 -> [w215 _]
                tunnel: w166 -> [w216 _]
                tunnel: w165 -> [w220 _]
                tunnel: w164 -> [w214 _]
                frame True {
                  w207 = FALSE ("Left Reset")
                  n95 = Greater Or Equal?(x=w215, y=w214) -> (x >= y?=w197:bool)
                  n96 = Select(t=-1.0, s=w201, f=0.1) -> (s? t:f=w229:dbl)
                  n97 = Greater Or Equal?(x=w216, y=w220) -> (x >= y?=w199:bool)
                  n98 = Greater Or Equal?(x=w242, y=w225) -> (x >= y?=w192:bool)
                  n99 = Greater Or Equal?(x=w243, y=w244) -> (x >= y?=w193:bool)
                  n100 = Select(t=1.0, s=w202, f=w229) -> (s? t:f=w212:dbl)
                  n101 = Select(t=-1.0, s=w203, f=0.1) -> (s? t:f=w228:dbl)
                  n102 = Select(t=1.0, s=w204, f=w228) -> (s? t:f=w218:dbl)
                  n103 = Select(t=0.0, s=w197, f=w212) -> (s? t:f=w211:dbl)
                  n104 = Select(t=1.0, s=w226, f=0.0) -> (s? t:f=w227:dbl)
                  n105 = Not Or(1:w203, 2:w204) -> (0:w200:bool)
                  n106 = Not Or(1:w201, 2:w202) -> (0:w198:bool)
                  n107 = Select(t=0.0, s=w199, f=w218) -> (s? t:f=w217:dbl)
                  n108 = call <vilib>:"WPI_MotorControlRefNum Registry Get.vi"("refnum name"="Wrist") -> ("error out"=w250:errorcluster, "MotorControlDevRef"=w251:T5)  [unwired: 9 in]
                  n109 = call <vilib>:"WPI_SolenoidRefNum Registry Get.vi"("refnum name"="SOL A") -> ("error out"=w259:errorcluster, "SolenoidDevRef"=w260:T10)  [unwired: 9 in]
                  n110 = call <vilib>:"WPI_SolenoidRefNum Registry Get.vi"("refnum name"="SOL B") -> ("error out"=w256:errorcluster, "SolenoidDevRef"=w257:T10)  [unwired: 9 in]
                  n111 = call <vilib>:"WPI_MotorControlRefNum Registry Get.vi"("refnum name"="Intake") -> ("error out"=w252:errorcluster, "MotorControlDevRef"=w253:T5)  [unwired: 9 in]
                  n112 = call <vilib>:"WPI_MotorControlRefNum Registry Get.vi"("refnum name"="Lift") -> ("error out"=w254:errorcluster, "MotorControlDevRef"=w255:T5)  [unwired: 9 in]
                  n113 = call <vilib>:"WPI_MotorControlSetOutput.vi"("error in (no error)"=w250, "Output"=w211, "MotorControlDevRef"=w251) -> ()  [unwired: 6 in, 3 out]
                  n114 = call-poly <vilib>:"WPI_SolenoidSet.vi"("error in (no error)"=w259, "Value"=w246, "SolenoidDevRef"=w260) -> ()  [unwired: 7 in, 2 out]
                  n115 = call-poly <vilib>:"WPI_SolenoidSet.vi"("error in (no error)"=w256, "Value"=w245, "SolenoidDevRef"=w257) -> ()  [unwired: 7 in, 2 out]
                  n116 = Or(x=w200, y=w199) -> (x .or. y?=w196:bool)
                  n117 = Or(x=w198, y=w197) -> (x .or. y?=w195:bool)
                  n118 = call <vilib>:"WPI_MotorControlSetOutput.vi"("error in (no error)"=w252, "Output"=w227, "MotorControlDevRef"=w253) -> ()  [unwired: 6 in, 3 out]
                  n119 = call <vilib>:"WPI_MotorControlSetOutput.vi"("error in (no error)"=w254, "Output"=w217, "MotorControlDevRef"=w255) -> ()  [unwired: 6 in, 3 out]
                  n120 = And(x=w196, y=w195) -> (x .and. y?=w194:bool)
                  n121 = Select(t=0.0, s=w193, f=w222) -> (s? t:f=w205:dbl)
                  n122 = Select(t=0.0, s=w192, f=w221) -> (s? t:f=w206:dbl)
                  n123 = call <vilib>:"WPI_RobotDriveTankDrive.vi"("Right axis value"=w205, "Left axis value"=w206, "RobotDriveDevRef"=w263) -> ("error out"=w239:errorcluster, "Motor Values"=w224:dbl[], "RobotDriveDevRef"=w264:T4)  [unwired: 6 in]
                  n124 = global write "Robot Global Data.vi" "Wrist Reset"(w207) -> ()
                  n125 = global write "Robot Global Data.vi" "Left Reset"(w207) -> ()
                  n126 = global write "Robot Global Data.vi" "Right Reset"(w207) -> ()
                  n127 = And(x=w192, y=w193) -> (x .and. y?=w209:bool)
                  n128 = And(x=w194, y=w209) -> (x .and. y?=w208:bool)
                  n129 = call-poly <vilib>:"NT Write Value.vi"("Numeric Array"=w224, "Name"="RobotDrive Motors") -> ()  [unwired: 9 in, 1 out]
                  n130 = Select(t=0.0, s=w208, f=w240) -> (s? t:f=w223:dbl)
                }
                frame False {
                  w266 = TRUE ("Left Reset")
                  n131 = Select(t=-1.0, s=w271, f=0.0) -> (s? t:f=w270:dbl)
                  n132 = global write "Robot Global Data.vi" "Wrist Reset"(w266) -> ()
                  n133 = global write "Robot Global Data.vi" "Left Reset"(w266) -> ()
                  n134 = global write "Robot Global Data.vi" "Right Reset"(w266) -> ()
                  n135 = call <vilib>:"WPI_RobotDriveTankDrive.vi"("Right axis value"=0.0, "Left axis value"=0.0, "RobotDriveDevRef"=w281) -> ("error out"=w279:errorcluster, "Motor Values"=w284:dbl[], "RobotDriveDevRef"=w280:T4)  [unwired: 6 in]
                  n136 = Wait (ms)(milliseconds to wait=w269) -> ()  [unwired: 1 out]
                  n137 = call <vilib>:"WPI_MotorControlRefNum Registry Get.vi"("refnum name"="Intake") -> ("error out"=w275:errorcluster, "MotorControlDevRef"=w276:T5)  [unwired: 9 in]
                  n138 = call-poly <vilib>:"NT Write Value.vi"("Numeric Array"=w284, "Name"="RobotDrive Motors") -> ()  [unwired: 9 in, 1 out]
                  n139 = global read "Robot Global Data.vi" "Wrist Reset"() -> (w265:bool)
                  n140 = global read "Robot Global Data.vi" "Right Reset"() -> (w277:bool)
                  n141 = global read "Robot Global Data.vi" "Left Reset"() -> (w278:bool)
                  n142 = call <vilib>:"WPI_MotorControlSetOutput.vi"("error in (no error)"=w275, "Output"=w270, "MotorControlDevRef"=w276) -> ()  [unwired: 6 in, 3 out]
                  n143 = And(x=w278, y=w277) -> (x .and. y?=w268:bool)
                  n144 = And(x=w268, y=w265) -> (x .and. y?=w267:bool)
                }
              }
            }
            n145 = call <vilib>:"WPI_RobotDriveDelayAndUpdateSafety.vi"("error in (no error)"=w158, "Delay (s)"=w160, "RobotDriveDevRef"=w159) -> ("RobotDriveDevRef 2"=w163:T4)  [unwired: 7 in, 1 out]
          }
        }
        frame "LRL" {
          n146 = Array Size(array="Left LRL") -> (size(s)=w287:i32)
          n147 = call <vilib>:"WPI_RobotDriveRefNum Registry Get.vi"("refnum name"="Left and Right Motors") -> ("RobotDriveDevRef"=w288:T4)  [unwired: 1 in, 9 out]
          n148 = for {
            N: w287 -> [_]
            shift-right: [w296] -> _
            shift-left: w288 -> [w295]
            tunnel: "Left LRL" -> [w294] mode=indexing
            i -> [w290]
            n149 = global write "Robot Global Data.vi" "Array Step"(w290) -> ()
            n150 = while {
              shift-right: [w324] -> w292
              shift-left: w295 -> [w323]
              tunnel: w294 -> [w320]
              tunnel: [w301] -> w293
              tunnel: [w304] -> w291
              stop <- w305 stop-if-true
              n151 = global read "Robot Global Data.vi" "Right Distance"() -> (w308:dbl)
              n152 = global read "Robot Global Data.vi" "Lift Distance"() -> (w299:dbl)
              n153 = global read "Robot Global Data.vi" "Left Distance"() -> (w307:dbl)
              n154 = Unbundle By Name(w320) -> ("Left Joystick"=w319:dbl, "Right Joystick"=w318:dbl, "Duration"=w306:dbl, "SOL A"=w317:bool, "SOL B"=w316:bool, "Lift Up"=w315:bool, "Lift Down"=w314:bool, "Intake In"=w313:bool, "Intake Out"=w312:bool, "Wrist Up"=w311:bool, "Wrist Down"=w310:bool, "Left Distance"=w300:dbl, "Right Distance"=w309:dbl, "Drive?"=w303:bool, "Lift Target"=w298:dbl, "Wrist Target"=w297:dbl)
              n155 = global read "Robot Global Data.vi" "Wrist Angle"() -> (w302:dbl)
              n156 = global read "Robot Global Data.vi" "Left Rate"() -> (w322:dbl)
              n157 = global read "Robot Global Data.vi" "Right Rate"() -> (w321:dbl)
              n158 = case shown="True" w303 {
                tunnel: [w397 w413] -> w324
                tunnel: w323 -> [w396 w414]
                tunnel: w322 -> [_ _]
                tunnel: w321 -> [_ _]
                tunnel: w319 -> [w354 _]
                tunnel: w318 -> [w355 _]
                tunnel: w317 -> [w379 _]
                tunnel: w316 -> [w378 _]
                tunnel: w315 -> [w337 _]
                tunnel: w314 -> [w336 _]
                tunnel: w313 -> [w359 _]
                tunnel: w312 -> [_ w404]
                tunnel: w311 -> [w335 _]
                tunnel: w310 -> [w334 _]
                tunnel: w300 -> [w358 _]
                tunnel: w309 -> [w377 _]
                tunnel: w308 -> [w376 _]
                tunnel: w307 -> [w375 _]
                tunnel: w306 -> [w373 w402]
                tunnel: [w356 w402] -> w301
                tunnel: [w341 w400] -> w305
                tunnel: [w372 w412] -> w304
                tunnel: w302 -> [w348 _]
                tunnel: w299 -> [w349 _]
                tunnel: w298 -> [w353 _]
                tunnel: w297 -> [w347 _]
                frame True {
                  w340 = FALSE ("Left Reset")
                  n159 = Greater Or Equal?(x=w348, y=w347) -> (x >= y?=w330:bool)
                  n160 = Select(t=-1.0, s=w334, f=0.1) -> (s? t:f=w362:dbl)
                  n161 = Greater Or Equal?(x=w349, y=w353) -> (x >= y?=w332:bool)
                  n162 = Greater Or Equal?(x=w375, y=w358) -> (x >= y?=w325:bool)
                  n163 = Greater Or Equal?(x=w376, y=w377) -> (x >= y?=w326:bool)
                  n164 = Select(t=1.0, s=w335, f=w362) -> (s? t:f=w345:dbl)
                  n165 = Select(t=-1.0, s=w336, f=0.1) -> (s? t:f=w361:dbl)
                  n166 = Select(t=1.0, s=w337, f=w361) -> (s? t:f=w351:dbl)
                  n167 = Select(t=0.0, s=w330, f=w345) -> (s? t:f=w344:dbl)
                  n168 = Select(t=1.0, s=w359, f=0.0) -> (s? t:f=w360:dbl)
                  n169 = Not Or(1:w336, 2:w337) -> (0:w333:bool)
                  n170 = Not Or(1:w334, 2:w335) -> (0:w331:bool)
                  n171 = Select(t=0.0, s=w332, f=w351) -> (s? t:f=w350:dbl)
                  n172 = call <vilib>:"WPI_MotorControlRefNum Registry Get.vi"("refnum name"="Wrist") -> ("error out"=w383:errorcluster, "MotorControlDevRef"=w384:T5)  [unwired: 9 in]
                  n173 = call <vilib>:"WPI_SolenoidRefNum Registry Get.vi"("refnum name"="SOL A") -> ("error out"=w392:errorcluster, "SolenoidDevRef"=w393:T10)  [unwired: 9 in]
                  n174 = call <vilib>:"WPI_SolenoidRefNum Registry Get.vi"("refnum name"="SOL B") -> ("error out"=w389:errorcluster, "SolenoidDevRef"=w390:T10)  [unwired: 9 in]
                  n175 = call <vilib>:"WPI_MotorControlRefNum Registry Get.vi"("refnum name"="Intake") -> ("error out"=w385:errorcluster, "MotorControlDevRef"=w386:T5)  [unwired: 9 in]
                  n176 = call <vilib>:"WPI_MotorControlRefNum Registry Get.vi"("refnum name"="Lift") -> ("error out"=w387:errorcluster, "MotorControlDevRef"=w388:T5)  [unwired: 9 in]
                  n177 = call <vilib>:"WPI_MotorControlSetOutput.vi"("error in (no error)"=w383, "Output"=w344, "MotorControlDevRef"=w384) -> ()  [unwired: 6 in, 3 out]
                  n178 = call-poly <vilib>:"WPI_SolenoidSet.vi"("error in (no error)"=w392, "Value"=w379, "SolenoidDevRef"=w393) -> ()  [unwired: 7 in, 2 out]
                  n179 = call-poly <vilib>:"WPI_SolenoidSet.vi"("error in (no error)"=w389, "Value"=w378, "SolenoidDevRef"=w390) -> ()  [unwired: 7 in, 2 out]
                  n180 = Or(x=w333, y=w332) -> (x .or. y?=w329:bool)
                  n181 = Or(x=w331, y=w330) -> (x .or. y?=w328:bool)
                  n182 = call <vilib>:"WPI_MotorControlSetOutput.vi"("error in (no error)"=w385, "Output"=w360, "MotorControlDevRef"=w386) -> ()  [unwired: 6 in, 3 out]
                  n183 = call <vilib>:"WPI_MotorControlSetOutput.vi"("error in (no error)"=w387, "Output"=w350, "MotorControlDevRef"=w388) -> ()  [unwired: 6 in, 3 out]
                  n184 = And(x=w329, y=w328) -> (x .and. y?=w327:bool)
                  n185 = Select(t=0.0, s=w326, f=w355) -> (s? t:f=w338:dbl)
                  n186 = Select(t=0.0, s=w325, f=w354) -> (s? t:f=w339:dbl)
                  n187 = call <vilib>:"WPI_RobotDriveTankDrive.vi"("Right axis value"=w338, "Left axis value"=w339, "RobotDriveDevRef"=w396) -> ("error out"=w372:errorcluster, "Motor Values"=w357:dbl[], "RobotDriveDevRef"=w397:T4)  [unwired: 6 in]
                  n188 = global write "Robot Global Data.vi" "Wrist Reset"(w340) -> ()
                  n189 = global write "Robot Global Data.vi" "Left Reset"(w340) -> ()
                  n190 = global write "Robot Global Data.vi" "Right Reset"(w340) -> ()
                  n191 = And(x=w325, y=w326) -> (x .and. y?=w342:bool)
                  n192 = And(x=w327, y=w342) -> (x .and. y?=w341:bool)
                  n193 = call-poly <vilib>:"NT Write Value.vi"("Numeric Array"=w357, "Name"="RobotDrive Motors") -> ()  [unwired: 9 in, 1 out]
                  n194 = Select(t=0.0, s=w341, f=w373) -> (s? t:f=w356:dbl)
                }
                frame False {
                  w399 = TRUE ("Left Reset")
                  n195 = Select(t=-1.0, s=w404, f=0.0) -> (s? t:f=w403:dbl)
                  n196 = global write "Robot Global Data.vi" "Wrist Reset"(w399) -> ()
                  n197 = global write "Robot Global Data.vi" "Left Reset"(w399) -> ()
                  n198 = global write "Robot Global Data.vi" "Right Reset"(w399) -> ()
                  n199 = call <vilib>:"WPI_RobotDriveTankDrive.vi"("Right axis value"=0.0, "Left axis value"=0.0, "RobotDriveDevRef"=w414) -> ("error out"=w412:errorcluster, "Motor Values"=w417:dbl[], "RobotDriveDevRef"=w413:T4)  [unwired: 6 in]
                  n200 = Wait (ms)(milliseconds to wait=w402) -> ()  [unwired: 1 out]
                  n201 = call <vilib>:"WPI_MotorControlRefNum Registry Get.vi"("refnum name"="Intake") -> ("error out"=w408:errorcluster, "MotorControlDevRef"=w409:T5)  [unwired: 9 in]
                  n202 = call-poly <vilib>:"NT Write Value.vi"("Numeric Array"=w417, "Name"="RobotDrive Motors") -> ()  [unwired: 9 in, 1 out]
                  n203 = global read "Robot Global Data.vi" "Wrist Reset"() -> (w398:bool)
                  n204 = global read "Robot Global Data.vi" "Right Reset"() -> (w410:bool)
                  n205 = global read "Robot Global Data.vi" "Left Reset"() -> (w411:bool)
                  n206 = call <vilib>:"WPI_MotorControlSetOutput.vi"("error in (no error)"=w408, "Output"=w403, "MotorControlDevRef"=w409) -> ()  [unwired: 6 in, 3 out]
                  n207 = And(x=w411, y=w410) -> (x .and. y?=w401:bool)
                  n208 = And(x=w401, y=w398) -> (x .and. y?=w400:bool)
                }
              }
            }
            n209 = call <vilib>:"WPI_RobotDriveDelayAndUpdateSafety.vi"("error in (no error)"=w291, "Delay (s)"=w293, "RobotDriveDevRef"=w292) -> ("RobotDriveDevRef 2"=w296:T4)  [unwired: 7 in, 1 out]
          }
        }
        frame "RLR" {
          n210 = Array Size(array="Left RLR") -> (size(s)=w420:i32)
          n211 = call <vilib>:"WPI_RobotDriveRefNum Registry Get.vi"("refnum name"="Left and Right Motors") -> ("RobotDriveDevRef"=w421:T4)  [unwired: 1 in, 9 out]
          n212 = for {
            N: w420 -> [_]
            shift-right: [w429] -> _
            shift-left: w421 -> [w428]
            tunnel: "Left RLR" -> [w427] mode=indexing
            i -> [w423]
            n213 = global write "Robot Global Data.vi" "Array Step"(w423) -> ()
            n214 = while {
              shift-right: [w457] -> w425
              shift-left: w428 -> [w456]
              tunnel: w427 -> [w453]
              tunnel: [w434] -> w426
              tunnel: [w437] -> w424
              stop <- w438 stop-if-true
              n215 = global read "Robot Global Data.vi" "Right Distance"() -> (w441:dbl)
              n216 = global read "Robot Global Data.vi" "Lift Distance"() -> (w432:dbl)
              n217 = global read "Robot Global Data.vi" "Left Distance"() -> (w440:dbl)
              n218 = Unbundle By Name(w453) -> ("Left Joystick"=w452:dbl, "Right Joystick"=w451:dbl, "Duration"=w439:dbl, "SOL A"=w450:bool, "SOL B"=w449:bool, "Lift Up"=w448:bool, "Lift Down"=w447:bool, "Intake In"=w446:bool, "Intake Out"=w445:bool, "Wrist Up"=w444:bool, "Wrist Down"=w443:bool, "Left Distance"=w433:dbl, "Right Distance"=w442:dbl, "Drive?"=w436:bool, "Lift Target"=w431:dbl, "Wrist Target"=w430:dbl)
              n219 = global read "Robot Global Data.vi" "Wrist Angle"() -> (w435:dbl)
              n220 = global read "Robot Global Data.vi" "Left Rate"() -> (w455:dbl)
              n221 = global read "Robot Global Data.vi" "Right Rate"() -> (w454:dbl)
              n222 = case shown="True" w436 {
                tunnel: [w530 w548] -> w457
                tunnel: w456 -> [w529 w549]
                tunnel: w455 -> [_ _]
                tunnel: w454 -> [_ _]
                tunnel: w452 -> [w487 _]
                tunnel: w451 -> [w488 _]
                tunnel: w450 -> [w512 _]
                tunnel: w449 -> [w511 _]
                tunnel: w448 -> [w470 _]
                tunnel: w447 -> [w469 _]
                tunnel: w446 -> [w492 _]
                tunnel: w445 -> [_ w539]
                tunnel: w444 -> [w468 _]
                tunnel: w443 -> [w467 _]
                tunnel: w433 -> [w491 _]
                tunnel: w442 -> [w510 _]
                tunnel: w441 -> [w509 _]
                tunnel: w440 -> [w508 _]
                tunnel: w439 -> [w506 w537]
                tunnel: [w489 w537] -> w434
                tunnel: [w474 w532] -> w438
                tunnel: [w505 w547] -> w437
                tunnel: w435 -> [w481 _]
                tunnel: w432 -> [w482 _]
                tunnel: w431 -> [w486 _]
                tunnel: w430 -> [w480 _]
                frame True {
                  w473 = FALSE ("Left Reset")
                  n223 = Greater Or Equal?(x=w481, y=w480) -> (x >= y?=w463:bool)
                  n224 = Select(t=-1.0, s=w467, f=0.1) -> (s? t:f=w495:dbl)
                  n225 = Greater Or Equal?(x=w482, y=w486) -> (x >= y?=w465:bool)
                  n226 = Greater Or Equal?(x=w508, y=w491) -> (x >= y?=w458:bool)
                  n227 = Greater Or Equal?(x=w509, y=w510) -> (x >= y?=w459:bool)
                  n228 = Select(t=1.0, s=w468, f=w495) -> (s? t:f=w478:dbl)
                  n229 = Select(t=-1.0, s=w469, f=0.1) -> (s? t:f=w494:dbl)
                  n230 = Select(t=1.0, s=w470, f=w494) -> (s? t:f=w484:dbl)
                  n231 = Select(t=0.0, s=w463, f=w478) -> (s? t:f=w477:dbl)
                  n232 = Select(t=1.0, s=w492, f=0.0) -> (s? t:f=w493:dbl)
                  n233 = Not Or(1:w469, 2:w470) -> (0:w466:bool)
                  n234 = Not Or(1:w467, 2:w468) -> (0:w464:bool)
                  n235 = Select(t=0.0, s=w465, f=w484) -> (s? t:f=w483:dbl)
                  n236 = call <vilib>:"WPI_MotorControlRefNum Registry Get.vi"("refnum name"="Wrist") -> ("error out"=w516:errorcluster, "MotorControlDevRef"=w517:T5)  [unwired: 9 in]
                  n237 = call <vilib>:"WPI_SolenoidRefNum Registry Get.vi"("refnum name"="SOL A") -> ("error out"=w525:errorcluster, "SolenoidDevRef"=w526:T10)  [unwired: 9 in]
                  n238 = call <vilib>:"WPI_SolenoidRefNum Registry Get.vi"("refnum name"="SOL B") -> ("error out"=w522:errorcluster, "SolenoidDevRef"=w523:T10)  [unwired: 9 in]
                  n239 = call <vilib>:"WPI_MotorControlRefNum Registry Get.vi"("refnum name"="Intake") -> ("error out"=w518:errorcluster, "MotorControlDevRef"=w519:T5)  [unwired: 9 in]
                  n240 = call <vilib>:"WPI_MotorControlRefNum Registry Get.vi"("refnum name"="Lift") -> ("error out"=w520:errorcluster, "MotorControlDevRef"=w521:T5)  [unwired: 9 in]
                  n241 = call <vilib>:"WPI_MotorControlSetOutput.vi"("error in (no error)"=w516, "Output"=w477, "MotorControlDevRef"=w517) -> ()  [unwired: 6 in, 3 out]
                  n242 = call-poly <vilib>:"WPI_SolenoidSet.vi"("error in (no error)"=w525, "Value"=w512, "SolenoidDevRef"=w526) -> ()  [unwired: 7 in, 2 out]
                  n243 = call-poly <vilib>:"WPI_SolenoidSet.vi"("error in (no error)"=w522, "Value"=w511, "SolenoidDevRef"=w523) -> ()  [unwired: 7 in, 2 out]
                  n244 = Or(x=w466, y=w465) -> (x .or. y?=w462:bool)
                  n245 = Or(x=w464, y=w463) -> (x .or. y?=w461:bool)
                  n246 = call <vilib>:"WPI_MotorControlSetOutput.vi"("error in (no error)"=w518, "Output"=w493, "MotorControlDevRef"=w519) -> ()  [unwired: 6 in, 3 out]
                  n247 = call <vilib>:"WPI_MotorControlSetOutput.vi"("error in (no error)"=w520, "Output"=w483, "MotorControlDevRef"=w521) -> ()  [unwired: 6 in, 3 out]
                  n248 = And(x=w462, y=w461) -> (x .and. y?=w460:bool)
                  n249 = Select(t=0.0, s=w459, f=w488) -> (s? t:f=w471:dbl)
                  n250 = Select(t=0.0, s=w458, f=w487) -> (s? t:f=w472:dbl)
                  n251 = call <vilib>:"WPI_RobotDriveTankDrive.vi"("Right axis value"=w471, "Left axis value"=w472, "RobotDriveDevRef"=w529) -> ("error out"=w505:errorcluster, "Motor Values"=w490:dbl[], "RobotDriveDevRef"=w530:T4)  [unwired: 6 in]
                  n252 = global write "Robot Global Data.vi" "Wrist Reset"(w473) -> ()
                  n253 = global write "Robot Global Data.vi" "Left Reset"(w473) -> ()
                  n254 = global write "Robot Global Data.vi" "Right Reset"(w473) -> ()
                  n255 = global write "Robot Global Data.vi" "Lift Reset"(w473) -> ()
                  n256 = And(x=w458, y=w459) -> (x .and. y?=w475:bool)
                  n257 = And(x=w460, y=w475) -> (x .and. y?=w474:bool)
                  n258 = call-poly <vilib>:"NT Write Value.vi"("Numeric Array"=w490, "Name"="RobotDrive Motors") -> ()  [unwired: 9 in, 1 out]
                  n259 = Select(t=0.0, s=w474, f=w506) -> (s? t:f=w489:dbl)
                }
                frame False {
                  w531 = TRUE ("Left Reset")
                  n260 = Select(t=-1.0, s=w539, f=0.0) -> (s? t:f=w538:dbl)
                  n261 = global write "Robot Global Data.vi" "Wrist Reset"(w531) -> ()
                  n262 = global write "Robot Global Data.vi" "Left Reset"(w531) -> ()
                  n263 = global write "Robot Global Data.vi" "Right Reset"(w531) -> ()
                  n264 = global write "Robot Global Data.vi" "Lift Reset"(w531) -> ()
                  n265 = call <vilib>:"WPI_RobotDriveTankDrive.vi"("Right axis value"=0.0, "Left axis value"=0.0, "RobotDriveDevRef"=w549) -> ("error out"=w547:errorcluster, "Motor Values"=w552:dbl[], "RobotDriveDevRef"=w548:T4)  [unwired: 6 in]
                  n266 = Wait (ms)(milliseconds to wait=w537) -> ()  [unwired: 1 out]
                  n267 = call <vilib>:"WPI_MotorControlRefNum Registry Get.vi"("refnum name"="Intake") -> ("error out"=w543:errorcluster, "MotorControlDevRef"=w544:T5)  [unwired: 9 in]
                  n268 = call-poly <vilib>:"NT Write Value.vi"("Numeric Array"=w552, "Name"="RobotDrive Motors") -> ()  [unwired: 9 in, 1 out]
                  n269 = global read "Robot Global Data.vi" "Wrist Reset"() -> (w535:bool)
                  n270 = global read "Robot Global Data.vi" "Right Reset"() -> (w545:bool)
                  n271 = global read "Robot Global Data.vi" "Lift Reset"() -> (w536:bool)
                  n272 = global read "Robot Global Data.vi" "Left Reset"() -> (w546:bool)
                  n273 = call <vilib>:"WPI_MotorControlSetOutput.vi"("error in (no error)"=w543, "Output"=w538, "MotorControlDevRef"=w544) -> ()  [unwired: 6 in, 3 out]
                  n274 = And(x=w546, y=w545) -> (x .and. y?=w533:bool)
                  n275 = And(x=w536, y=w535) -> (x .and. y?=w534:bool)
                  n276 = And(x=w533, y=w534) -> (x .and. y?=w532:bool)
                }
              }
            }
            n277 = call <vilib>:"WPI_RobotDriveDelayAndUpdateSafety.vi"("error in (no error)"=w424, "Delay (s)"=w426, "RobotDriveDevRef"=w425) -> ("RobotDriveDevRef 2"=w429:T4)  [unwired: 7 in, 1 out]
          }
        }
        frame "LLL", Default {
          n278 = Array Size(array="Left LLL") -> (size(s)=w555:i32)
          n279 = call <vilib>:"WPI_RobotDriveRefNum Registry Get.vi"("refnum name"="Left and Right Motors") -> ("RobotDriveDevRef"=w556:T4)  [unwired: 1 in, 9 out]
          n280 = for {
            N: w555 -> [_]
            shift-right: [w564] -> _
            shift-left: w556 -> [w563]
            tunnel: "Left LLL" -> [w562] mode=indexing
            i -> [w558]
            n281 = global write "Robot Global Data.vi" "Array Step"(w558) -> ()
            n282 = while {
              shift-right: [w592] -> w560
              shift-left: w563 -> [w591]
              tunnel: w562 -> [w588]
              tunnel: [w569] -> w561
              tunnel: [w572] -> w559
              stop <- w573 stop-if-true
              n283 = global read "Robot Global Data.vi" "Right Distance"() -> (w576:dbl)
              n284 = global read "Robot Global Data.vi" "Lift Distance"() -> (w567:dbl)
              n285 = global read "Robot Global Data.vi" "Left Distance"() -> (w575:dbl)
              n286 = Unbundle By Name(w588) -> ("Left Joystick"=w587:dbl, "Right Joystick"=w586:dbl, "Duration"=w574:dbl, "SOL A"=w585:bool, "SOL B"=w584:bool, "Lift Up"=w583:bool, "Lift Down"=w582:bool, "Intake In"=w581:bool, "Intake Out"=w580:bool, "Wrist Up"=w579:bool, "Wrist Down"=w578:bool, "Left Distance"=w568:dbl, "Right Distance"=w577:dbl, "Drive?"=w571:bool, "Lift Target"=w566:dbl, "Wrist Target"=w565:dbl)
              n287 = global read "Robot Global Data.vi" "Wrist Angle"() -> (w570:dbl)
              n288 = global read "Robot Global Data.vi" "Left Rate"() -> (w590:dbl)
              n289 = global read "Robot Global Data.vi" "Right Rate"() -> (w589:dbl)
              n290 = case shown="True" w571 {
                tunnel: [w665 w683] -> w592
                tunnel: w591 -> [w664 w684]
                tunnel: w590 -> [_ _]
                tunnel: w589 -> [_ _]
                tunnel: w587 -> [w622 _]
                tunnel: w586 -> [w623 _]
                tunnel: w585 -> [w647 _]
                tunnel: w584 -> [w646 _]
                tunnel: w583 -> [w605 _]
                tunnel: w582 -> [w604 _]
                tunnel: w581 -> [w627 _]
                tunnel: w580 -> [_ w674]
                tunnel: w579 -> [w603 _]
                tunnel: w578 -> [w602 _]
                tunnel: w568 -> [w626 _]
                tunnel: w577 -> [w645 _]
                tunnel: w576 -> [w644 _]
                tunnel: w575 -> [w643 _]
                tunnel: w574 -> [w641 w672]
                tunnel: [w624 w672] -> w569
                tunnel: [w609 w667] -> w573
                tunnel: [w640 w682] -> w572
                tunnel: w570 -> [w616 _]
                tunnel: w567 -> [w617 _]
                tunnel: w566 -> [w621 _]
                tunnel: w565 -> [w615 _]
                frame True {
                  w608 = FALSE ("Left Reset")
                  n291 = Greater Or Equal?(x=w616, y=w615) -> (x >= y?=w598:bool)
                  n292 = Select(t=-1.0, s=w602, f=0.1) -> (s? t:f=w630:dbl)
                  n293 = Greater Or Equal?(x=w617, y=w621) -> (x >= y?=w600:bool)
                  n294 = Greater Or Equal?(x=w643, y=w626) -> (x >= y?=w593:bool)
                  n295 = Greater Or Equal?(x=w644, y=w645) -> (x >= y?=w594:bool)
                  n296 = Select(t=1.0, s=w603, f=w630) -> (s? t:f=w613:dbl)
                  n297 = Select(t=-1.0, s=w604, f=0.1) -> (s? t:f=w629:dbl)
                  n298 = Select(t=1.0, s=w605, f=w629) -> (s? t:f=w619:dbl)
                  n299 = Select(t=0.0, s=w598, f=w613) -> (s? t:f=w612:dbl)
                  n300 = Select(t=1.0, s=w627, f=0.0) -> (s? t:f=w628:dbl)
                  n301 = Not Or(1:w604, 2:w605) -> (0:w601:bool)
                  n302 = Not Or(1:w602, 2:w603) -> (0:w599:bool)
                  n303 = Select(t=0.0, s=w600, f=w619) -> (s? t:f=w618:dbl)
                  n304 = call <vilib>:"WPI_MotorControlRefNum Registry Get.vi"("refnum name"="Wrist") -> ("error out"=w651:errorcluster, "MotorControlDevRef"=w652:T5)  [unwired: 9 in]
                  n305 = call <vilib>:"WPI_SolenoidRefNum Registry Get.vi"("refnum name"="SOL A") -> ("error out"=w660:errorcluster, "SolenoidDevRef"=w661:T10)  [unwired: 9 in]
                  n306 = call <vilib>:"WPI_SolenoidRefNum Registry Get.vi"("refnum name"="SOL B") -> ("error out"=w657:errorcluster, "SolenoidDevRef"=w658:T10)  [unwired: 9 in]
                  n307 = call <vilib>:"WPI_MotorControlRefNum Registry Get.vi"("refnum name"="Intake") -> ("error out"=w653:errorcluster, "MotorControlDevRef"=w654:T5)  [unwired: 9 in]
                  n308 = call <vilib>:"WPI_MotorControlRefNum Registry Get.vi"("refnum name"="Lift") -> ("error out"=w655:errorcluster, "MotorControlDevRef"=w656:T5)  [unwired: 9 in]
                  n309 = call <vilib>:"WPI_MotorControlSetOutput.vi"("error in (no error)"=w651, "Output"=w612, "MotorControlDevRef"=w652) -> ()  [unwired: 6 in, 3 out]
                  n310 = call-poly <vilib>:"WPI_SolenoidSet.vi"("error in (no error)"=w660, "Value"=w647, "SolenoidDevRef"=w661) -> ()  [unwired: 7 in, 2 out]
                  n311 = call-poly <vilib>:"WPI_SolenoidSet.vi"("error in (no error)"=w657, "Value"=w646, "SolenoidDevRef"=w658) -> ()  [unwired: 7 in, 2 out]
                  n312 = Or(x=w601, y=w600) -> (x .or. y?=w597:bool)
                  n313 = Or(x=w599, y=w598) -> (x .or. y?=w596:bool)
                  n314 = call <vilib>:"WPI_MotorControlSetOutput.vi"("error in (no error)"=w653, "Output"=w628, "MotorControlDevRef"=w654) -> ()  [unwired: 6 in, 3 out]
                  n315 = call <vilib>:"WPI_MotorControlSetOutput.vi"("error in (no error)"=w655, "Output"=w618, "MotorControlDevRef"=w656) -> ()  [unwired: 6 in, 3 out]
                  n316 = And(x=w597, y=w596) -> (x .and. y?=w595:bool)
                  n317 = Select(t=0.0, s=w594, f=w623) -> (s? t:f=w606:dbl)
                  n318 = Select(t=0.0, s=w593, f=w622) -> (s? t:f=w607:dbl)
                  n319 = call <vilib>:"WPI_RobotDriveTankDrive.vi"("Right axis value"=w606, "Left axis value"=w607, "RobotDriveDevRef"=w664) -> ("error out"=w640:errorcluster, "Motor Values"=w625:dbl[], "RobotDriveDevRef"=w665:T4)  [unwired: 6 in]
                  n320 = global write "Robot Global Data.vi" "Wrist Reset"(w608) -> ()
                  n321 = global write "Robot Global Data.vi" "Left Reset"(w608) -> ()
                  n322 = global write "Robot Global Data.vi" "Right Reset"(w608) -> ()
                  n323 = global write "Robot Global Data.vi" "Lift Reset"(w608) -> ()
                  n324 = And(x=w593, y=w594) -> (x .and. y?=w610:bool)
                  n325 = And(x=w595, y=w610) -> (x .and. y?=w609:bool)
                  n326 = call-poly <vilib>:"NT Write Value.vi"("Numeric Array"=w625, "Name"="RobotDrive Motors") -> ()  [unwired: 9 in, 1 out]
                  n327 = Select(t=0.0, s=w609, f=w641) -> (s? t:f=w624:dbl)
                }
                frame False {
                  w666 = TRUE ("Left Reset")
                  n328 = Select(t=-1.0, s=w674, f=0.0) -> (s? t:f=w673:dbl)
                  n329 = global write "Robot Global Data.vi" "Wrist Reset"(w666) -> ()
                  n330 = global write "Robot Global Data.vi" "Left Reset"(w666) -> ()
                  n331 = global write "Robot Global Data.vi" "Right Reset"(w666) -> ()
                  n332 = global write "Robot Global Data.vi" "Lift Reset"(w666) -> ()
                  n333 = call <vilib>:"WPI_RobotDriveTankDrive.vi"("Right axis value"=0.0, "Left axis value"=0.0, "RobotDriveDevRef"=w684) -> ("error out"=w682:errorcluster, "Motor Values"=w687:dbl[], "RobotDriveDevRef"=w683:T4)  [unwired: 6 in]
                  n334 = Wait (ms)(milliseconds to wait=w672) -> ()  [unwired: 1 out]
                  n335 = call <vilib>:"WPI_MotorControlRefNum Registry Get.vi"("refnum name"="Intake") -> ("error out"=w678:errorcluster, "MotorControlDevRef"=w679:T5)  [unwired: 9 in]
                  n336 = call-poly <vilib>:"NT Write Value.vi"("Numeric Array"=w687, "Name"="RobotDrive Motors") -> ()  [unwired: 9 in, 1 out]
                  n337 = global read "Robot Global Data.vi" "Wrist Reset"() -> (w670:bool)
                  n338 = global read "Robot Global Data.vi" "Right Reset"() -> (w680:bool)
                  n339 = global read "Robot Global Data.vi" "Lift Reset"() -> (w671:bool)
                  n340 = global read "Robot Global Data.vi" "Left Reset"() -> (w681:bool)
                  n341 = call <vilib>:"WPI_MotorControlSetOutput.vi"("error in (no error)"=w678, "Output"=w673, "MotorControlDevRef"=w679) -> ()  [unwired: 6 in, 3 out]
                  n342 = And(x=w681, y=w680) -> (x .and. y?=w668:bool)
                  n343 = And(x=w671, y=w670) -> (x .and. y?=w669:bool)
                  n344 = And(x=w668, y=w669) -> (x .and. y?=w667:bool)
                }
              }
            }
            n345 = call <vilib>:"WPI_RobotDriveDelayAndUpdateSafety.vi"("error in (no error)"=w559, "Delay (s)"=w561, "RobotDriveDevRef"=w560) -> ("RobotDriveDevRef 2"=w564:T4)  [unwired: 7 in, 1 out]
          }
        }
      }
    }
    frame "Starting Center" {
      n346 = case shown="\"LLL\", Default" w689 {
        frame "RRR" {
          n347 = Array Size(array="Center RRR") -> (size(s)=w691:i32)
          n348 = call <vilib>:"WPI_RobotDriveRefNum Registry Get.vi"("refnum name"="Left and Right Motors") -> ("RobotDriveDevRef"=w692:T4)  [unwired: 1 in, 9 out]
          n349 = for {
            N: w691 -> [_]
            shift-right: [w700] -> _
            shift-left: w692 -> [w699]
            tunnel: "Center RRR" -> [w698] mode=indexing
            i -> [w694]
            n350 = global write "Robot Global Data.vi" "Array Step"(w694) -> ()
            n351 = while {
              shift-right: [w728] -> w696
              shift-left: w699 -> [w727]
              tunnel: w698 -> [w724]
              tunnel: [w705] -> w697
              tunnel: [w708] -> w695
              stop <- w709 stop-if-true
              n352 = global read "Robot Global Data.vi" "Right Distance"() -> (w712:dbl)
              n353 = global read "Robot Global Data.vi" "Lift Distance"() -> (w703:dbl)
              n354 = global read "Robot Global Data.vi" "Left Distance"() -> (w711:dbl)
              n355 = Unbundle By Name(w724) -> ("Left Joystick"=w723:dbl, "Right Joystick"=w722:dbl, "Duration"=w710:dbl, "SOL A"=w721:bool, "SOL B"=w720:bool, "Lift Up"=w719:bool, "Lift Down"=w718:bool, "Intake In"=w717:bool, "Intake Out"=w716:bool, "Wrist Up"=w715:bool, "Wrist Down"=w714:bool, "Left Distance"=w704:dbl, "Right Distance"=w713:dbl, "Drive?"=w707:bool, "Lift Target"=w702:dbl, "Wrist Target"=w701:dbl)
              n356 = global read "Robot Global Data.vi" "Wrist Angle"() -> (w706:dbl)
              n357 = global read "Robot Global Data.vi" "Left Rate"() -> (w726:dbl)
              n358 = global read "Robot Global Data.vi" "Right Rate"() -> (w725:dbl)
              n359 = case shown="True" w707 {
                tunnel: [w801 w819] -> w728
                tunnel: w727 -> [w800 w820]
                tunnel: w726 -> [_ _]
                tunnel: w725 -> [_ _]
                tunnel: w723 -> [w758 _]
                tunnel: w722 -> [w759 _]
                tunnel: w721 -> [w783 _]
                tunnel: w720 -> [w782 _]
                tunnel: w719 -> [w741 _]
                tunnel: w718 -> [w740 _]
                tunnel: w717 -> [w763 _]
                tunnel: w716 -> [_ w810]
                tunnel: w715 -> [w739 _]
                tunnel: w714 -> [w738 _]
                tunnel: w704 -> [w762 _]
                tunnel: w713 -> [w781 _]
                tunnel: w712 -> [w780 _]
                tunnel: w711 -> [w779 _]
                tunnel: w710 -> [w777 w808]
                tunnel: [w760 w808] -> w705
                tunnel: [w745 w803] -> w709
                tunnel: [w776 w818] -> w708
                tunnel: w706 -> [w752 _]
                tunnel: w703 -> [w753 _]
                tunnel: w702 -> [w757 _]
                tunnel: w701 -> [w751 _]
                frame True {
                  w744 = FALSE ("Left Reset")
                  n360 = Greater Or Equal?(x=w752, y=w751) -> (x >= y?=w734:bool)
                  n361 = Select(t=-1.0, s=w738, f=0.1) -> (s? t:f=w766:dbl)
                  n362 = Greater Or Equal?(x=w753, y=w757) -> (x >= y?=w736:bool)
                  n363 = Greater Or Equal?(x=w779, y=w762) -> (x >= y?=w729:bool)
                  n364 = Greater Or Equal?(x=w780, y=w781) -> (x >= y?=w730:bool)
                  n365 = Select(t=1.0, s=w739, f=w766) -> (s? t:f=w749:dbl)
                  n366 = Select(t=-1.0, s=w740, f=0.1) -> (s? t:f=w765:dbl)
                  n367 = Select(t=1.0, s=w741, f=w765) -> (s? t:f=w755:dbl)
                  n368 = Select(t=0.0, s=w734, f=w749) -> (s? t:f=w748:dbl)
                  n369 = Select(t=1.0, s=w763, f=0.0) -> (s? t:f=w764:dbl)
                  n370 = Not Or(1:w740, 2:w741) -> (0:w737:bool)
                  n371 = Not Or(1:w738, 2:w739) -> (0:w735:bool)
                  n372 = Select(t=0.0, s=w736, f=w755) -> (s? t:f=w754:dbl)
                  n373 = call <vilib>:"WPI_MotorControlRefNum Registry Get.vi"("refnum name"="Wrist") -> ("error out"=w787:errorcluster, "MotorControlDevRef"=w788:T5)  [unwired: 9 in]
                  n374 = call <vilib>:"WPI_SolenoidRefNum Registry Get.vi"("refnum name"="SOL A") -> ("error out"=w796:errorcluster, "SolenoidDevRef"=w797:T10)  [unwired: 9 in]
                  n375 = call <vilib>:"WPI_SolenoidRefNum Registry Get.vi"("refnum name"="SOL B") -> ("error out"=w793:errorcluster, "SolenoidDevRef"=w794:T10)  [unwired: 9 in]
                  n376 = call <vilib>:"WPI_MotorControlRefNum Registry Get.vi"("refnum name"="Intake") -> ("error out"=w789:errorcluster, "MotorControlDevRef"=w790:T5)  [unwired: 9 in]
                  n377 = call <vilib>:"WPI_MotorControlRefNum Registry Get.vi"("refnum name"="Lift") -> ("error out"=w791:errorcluster, "MotorControlDevRef"=w792:T5)  [unwired: 9 in]
                  n378 = call <vilib>:"WPI_MotorControlSetOutput.vi"("error in (no error)"=w787, "Output"=w748, "MotorControlDevRef"=w788) -> ()  [unwired: 6 in, 3 out]
                  n379 = call-poly <vilib>:"WPI_SolenoidSet.vi"("error in (no error)"=w796, "Value"=w783, "SolenoidDevRef"=w797) -> ()  [unwired: 7 in, 2 out]
                  n380 = call-poly <vilib>:"WPI_SolenoidSet.vi"("error in (no error)"=w793, "Value"=w782, "SolenoidDevRef"=w794) -> ()  [unwired: 7 in, 2 out]
                  n381 = Or(x=w737, y=w736) -> (x .or. y?=w733:bool)
                  n382 = Or(x=w735, y=w734) -> (x .or. y?=w732:bool)
                  n383 = call <vilib>:"WPI_MotorControlSetOutput.vi"("error in (no error)"=w789, "Output"=w764, "MotorControlDevRef"=w790) -> ()  [unwired: 6 in, 3 out]
                  n384 = call <vilib>:"WPI_MotorControlSetOutput.vi"("error in (no error)"=w791, "Output"=w754, "MotorControlDevRef"=w792) -> ()  [unwired: 6 in, 3 out]
                  n385 = And(x=w733, y=w732) -> (x .and. y?=w731:bool)
                  n386 = Select(t=0.0, s=w730, f=w759) -> (s? t:f=w742:dbl)
                  n387 = Select(t=0.0, s=w729, f=w758) -> (s? t:f=w743:dbl)
                  n388 = call <vilib>:"WPI_RobotDriveTankDrive.vi"("Right axis value"=w742, "Left axis value"=w743, "RobotDriveDevRef"=w800) -> ("error out"=w776:errorcluster, "Motor Values"=w761:dbl[], "RobotDriveDevRef"=w801:T4)  [unwired: 6 in]
                  n389 = global write "Robot Global Data.vi" "Wrist Reset"(w744) -> ()
                  n390 = global write "Robot Global Data.vi" "Left Reset"(w744) -> ()
                  n391 = global write "Robot Global Data.vi" "Right Reset"(w744) -> ()
                  n392 = global write "Robot Global Data.vi" "Lift Reset"(w744) -> ()
                  n393 = And(x=w729, y=w730) -> (x .and. y?=w746:bool)
                  n394 = And(x=w731, y=w746) -> (x .and. y?=w745:bool)
                  n395 = call-poly <vilib>:"NT Write Value.vi"("Numeric Array"=w761, "Name"="RobotDrive Motors") -> ()  [unwired: 9 in, 1 out]
                  n396 = Select(t=0.0, s=w745, f=w777) -> (s? t:f=w760:dbl)
                }
                frame False {
                  w802 = TRUE ("Left Reset")
                  n397 = Select(t=-1.0, s=w810, f=0.0) -> (s? t:f=w809:dbl)
                  n398 = global write "Robot Global Data.vi" "Wrist Reset"(w802) -> ()
                  n399 = global write "Robot Global Data.vi" "Left Reset"(w802) -> ()
                  n400 = global write "Robot Global Data.vi" "Right Reset"(w802) -> ()
                  n401 = global write "Robot Global Data.vi" "Lift Reset"(w802) -> ()
                  n402 = call <vilib>:"WPI_RobotDriveTankDrive.vi"("Right axis value"=0.0, "Left axis value"=0.0, "RobotDriveDevRef"=w820) -> ("error out"=w818:errorcluster, "Motor Values"=w823:dbl[], "RobotDriveDevRef"=w819:T4)  [unwired: 6 in]
                  n403 = Wait (ms)(milliseconds to wait=w808) -> ()  [unwired: 1 out]
                  n404 = call <vilib>:"WPI_MotorControlRefNum Registry Get.vi"("refnum name"="Intake") -> ("error out"=w814:errorcluster, "MotorControlDevRef"=w815:T5)  [unwired: 9 in]
                  n405 = call-poly <vilib>:"NT Write Value.vi"("Numeric Array"=w823, "Name"="RobotDrive Motors") -> ()  [unwired: 9 in, 1 out]
                  n406 = global read "Robot Global Data.vi" "Wrist Reset"() -> (w806:bool)
                  n407 = global read "Robot Global Data.vi" "Right Reset"() -> (w816:bool)
                  n408 = global read "Robot Global Data.vi" "Lift Reset"() -> (w807:bool)
                  n409 = global read "Robot Global Data.vi" "Left Reset"() -> (w817:bool)
                  n410 = call <vilib>:"WPI_MotorControlSetOutput.vi"("error in (no error)"=w814, "Output"=w809, "MotorControlDevRef"=w815) -> ()  [unwired: 6 in, 3 out]
                  n411 = And(x=w817, y=w816) -> (x .and. y?=w804:bool)
                  n412 = And(x=w807, y=w806) -> (x .and. y?=w805:bool)
                  n413 = And(x=w804, y=w805) -> (x .and. y?=w803:bool)
                }
              }
            }
            n414 = call <vilib>:"WPI_RobotDriveDelayAndUpdateSafety.vi"("error in (no error)"=w695, "Delay (s)"=w697, "RobotDriveDevRef"=w696) -> ("RobotDriveDevRef 2"=w700:T4)  [unwired: 7 in, 1 out]
          }
        }
        frame "LRL" {
          n415 = Array Size(array="Center LRL") -> (size(s)=w826:i32)
          n416 = call <vilib>:"WPI_RobotDriveRefNum Registry Get.vi"("refnum name"="Left and Right Motors") -> ("RobotDriveDevRef"=w827:T4)  [unwired: 1 in, 9 out]
          n417 = for {
            N: w826 -> [_]
            shift-right: [w835] -> _
            shift-left: w827 -> [w834]
            tunnel: "Center LRL" -> [w833] mode=indexing
            i -> [w829]
            n418 = global write "Robot Global Data.vi" "Array Step"(w829) -> ()
            n419 = while {
              shift-right: [w863] -> w831
              shift-left: w834 -> [w862]
              tunnel: w833 -> [w859]
              tunnel: [w840] -> w832
              tunnel: [w843] -> w830
              stop <- w844 stop-if-true
              n420 = global read "Robot Global Data.vi" "Right Distance"() -> (w847:dbl)
              n421 = global read "Robot Global Data.vi" "Lift Distance"() -> (w838:dbl)
              n422 = global read "Robot Global Data.vi" "Left Distance"() -> (w846:dbl)
              n423 = Unbundle By Name(w859) -> ("Left Joystick"=w858:dbl, "Right Joystick"=w857:dbl, "Duration"=w845:dbl, "SOL A"=w856:bool, "SOL B"=w855:bool, "Lift Up"=w854:bool, "Lift Down"=w853:bool, "Intake In"=w852:bool, "Intake Out"=w851:bool, "Wrist Up"=w850:bool, "Wrist Down"=w849:bool, "Left Distance"=w839:dbl, "Right Distance"=w848:dbl, "Drive?"=w842:bool, "Lift Target"=w837:dbl, "Wrist Target"=w836:dbl)
              n424 = global read "Robot Global Data.vi" "Wrist Angle"() -> (w841:dbl)
              n425 = global read "Robot Global Data.vi" "Left Rate"() -> (w861:dbl)
              n426 = global read "Robot Global Data.vi" "Right Rate"() -> (w860:dbl)
              n427 = case shown="True" w842 {
                tunnel: [w936 w954] -> w863
                tunnel: w862 -> [w935 w955]
                tunnel: w861 -> [_ _]
                tunnel: w860 -> [_ _]
                tunnel: w858 -> [w893 _]
                tunnel: w857 -> [w894 _]
                tunnel: w856 -> [w918 _]
                tunnel: w855 -> [w917 _]
                tunnel: w854 -> [w876 _]
                tunnel: w853 -> [w875 _]
                tunnel: w852 -> [w898 _]
                tunnel: w851 -> [_ w945]
                tunnel: w850 -> [w874 _]
                tunnel: w849 -> [w873 _]
                tunnel: w839 -> [w897 _]
                tunnel: w848 -> [w916 _]
                tunnel: w847 -> [w915 _]
                tunnel: w846 -> [w914 _]
                tunnel: w845 -> [w912 w943]
                tunnel: [w895 w943] -> w840
                tunnel: [w880 w938] -> w844
                tunnel: [w911 w953] -> w843
                tunnel: w841 -> [w887 _]
                tunnel: w838 -> [w888 _]
                tunnel: w837 -> [w892 _]
                tunnel: w836 -> [w886 _]
                frame True {
                  w879 = FALSE ("Left Reset")
                  n428 = Greater Or Equal?(x=w887, y=w886) -> (x >= y?=w869:bool)
                  n429 = Select(t=-1.0, s=w873, f=0.1) -> (s? t:f=w901:dbl)
                  n430 = Greater Or Equal?(x=w888, y=w892) -> (x >= y?=w871:bool)
                  n431 = Greater Or Equal?(x=w914, y=w897) -> (x >= y?=w864:bool)
                  n432 = Greater Or Equal?(x=w915, y=w916) -> (x >= y?=w865:bool)
                  n433 = Select(t=1.0, s=w874, f=w901) -> (s? t:f=w884:dbl)
                  n434 = Select(t=-1.0, s=w875, f=0.1) -> (s? t:f=w900:dbl)
                  n435 = Select(t=1.0, s=w876, f=w900) -> (s? t:f=w890:dbl)
                  n436 = Select(t=0.0, s=w869, f=w884) -> (s? t:f=w883:dbl)
                  n437 = Select(t=1.0, s=w898, f=0.0) -> (s? t:f=w899:dbl)
                  n438 = Not Or(1:w875, 2:w876) -> (0:w872:bool)
                  n439 = Not Or(1:w873, 2:w874) -> (0:w870:bool)
                  n440 = Select(t=0.0, s=w871, f=w890) -> (s? t:f=w889:dbl)
                  n441 = call <vilib>:"WPI_MotorControlRefNum Registry Get.vi"("refnum name"="Wrist") -> ("error out"=w922:errorcluster, "MotorControlDevRef"=w923:T5)  [unwired: 9 in]
                  n442 = call <vilib>:"WPI_SolenoidRefNum Registry Get.vi"("refnum name"="SOL A") -> ("error out"=w931:errorcluster, "SolenoidDevRef"=w932:T10)  [unwired: 9 in]
                  n443 = call <vilib>:"WPI_SolenoidRefNum Registry Get.vi"("refnum name"="SOL B") -> ("error out"=w928:errorcluster, "SolenoidDevRef"=w929:T10)  [unwired: 9 in]
                  n444 = call <vilib>:"WPI_MotorControlRefNum Registry Get.vi"("refnum name"="Intake") -> ("error out"=w924:errorcluster, "MotorControlDevRef"=w925:T5)  [unwired: 9 in]
                  n445 = call <vilib>:"WPI_MotorControlRefNum Registry Get.vi"("refnum name"="Lift") -> ("error out"=w926:errorcluster, "MotorControlDevRef"=w927:T5)  [unwired: 9 in]
                  n446 = call <vilib>:"WPI_MotorControlSetOutput.vi"("error in (no error)"=w922, "Output"=w883, "MotorControlDevRef"=w923) -> ()  [unwired: 6 in, 3 out]
                  n447 = call-poly <vilib>:"WPI_SolenoidSet.vi"("error in (no error)"=w931, "Value"=w918, "SolenoidDevRef"=w932) -> ()  [unwired: 7 in, 2 out]
                  n448 = call-poly <vilib>:"WPI_SolenoidSet.vi"("error in (no error)"=w928, "Value"=w917, "SolenoidDevRef"=w929) -> ()  [unwired: 7 in, 2 out]
                  n449 = Or(x=w872, y=w871) -> (x .or. y?=w868:bool)
                  n450 = Or(x=w870, y=w869) -> (x .or. y?=w867:bool)
                  n451 = call <vilib>:"WPI_MotorControlSetOutput.vi"("error in (no error)"=w924, "Output"=w899, "MotorControlDevRef"=w925) -> ()  [unwired: 6 in, 3 out]
                  n452 = call <vilib>:"WPI_MotorControlSetOutput.vi"("error in (no error)"=w926, "Output"=w889, "MotorControlDevRef"=w927) -> ()  [unwired: 6 in, 3 out]
                  n453 = And(x=w868, y=w867) -> (x .and. y?=w866:bool)
                  n454 = Select(t=0.0, s=w865, f=w894) -> (s? t:f=w877:dbl)
                  n455 = Select(t=0.0, s=w864, f=w893) -> (s? t:f=w878:dbl)
                  n456 = call <vilib>:"WPI_RobotDriveTankDrive.vi"("Right axis value"=w877, "Left axis value"=w878, "RobotDriveDevRef"=w935) -> ("error out"=w911:errorcluster, "Motor Values"=w896:dbl[], "RobotDriveDevRef"=w936:T4)  [unwired: 6 in]
                  n457 = global write "Robot Global Data.vi" "Wrist Reset"(w879) -> ()
                  n458 = global write "Robot Global Data.vi" "Left Reset"(w879) -> ()
                  n459 = global write "Robot Global Data.vi" "Right Reset"(w879) -> ()
                  n460 = global write "Robot Global Data.vi" "Lift Reset"(w879) -> ()
                  n461 = And(x=w864, y=w865) -> (x .and. y?=w881:bool)
                  n462 = And(x=w866, y=w881) -> (x .and. y?=w880:bool)
                  n463 = call-poly <vilib>:"NT Write Value.vi"("Numeric Array"=w896, "Name"="RobotDrive Motors") -> ()  [unwired: 9 in, 1 out]
                  n464 = Select(t=0.0, s=w880, f=w912) -> (s? t:f=w895:dbl)
                }
                frame False {
                  w937 = TRUE ("Left Reset")
                  n465 = Select(t=-1.0, s=w945, f=0.0) -> (s? t:f=w944:dbl)
                  n466 = global write "Robot Global Data.vi" "Wrist Reset"(w937) -> ()
                  n467 = global write "Robot Global Data.vi" "Left Reset"(w937) -> ()
                  n468 = global write "Robot Global Data.vi" "Right Reset"(w937) -> ()
                  n469 = global write "Robot Global Data.vi" "Lift Reset"(w937) -> ()
                  n470 = call <vilib>:"WPI_RobotDriveTankDrive.vi"("Right axis value"=0.0, "Left axis value"=0.0, "RobotDriveDevRef"=w955) -> ("error out"=w953:errorcluster, "Motor Values"=w958:dbl[], "RobotDriveDevRef"=w954:T4)  [unwired: 6 in]
                  n471 = Wait (ms)(milliseconds to wait=w943) -> ()  [unwired: 1 out]
                  n472 = call <vilib>:"WPI_MotorControlRefNum Registry Get.vi"("refnum name"="Intake") -> ("error out"=w949:errorcluster, "MotorControlDevRef"=w950:T5)  [unwired: 9 in]
                  n473 = call-poly <vilib>:"NT Write Value.vi"("Numeric Array"=w958, "Name"="RobotDrive Motors") -> ()  [unwired: 9 in, 1 out]
                  n474 = global read "Robot Global Data.vi" "Wrist Reset"() -> (w941:bool)
                  n475 = global read "Robot Global Data.vi" "Right Reset"() -> (w951:bool)
                  n476 = global read "Robot Global Data.vi" "Lift Reset"() -> (w942:bool)
                  n477 = global read "Robot Global Data.vi" "Left Reset"() -> (w952:bool)
                  n478 = call <vilib>:"WPI_MotorControlSetOutput.vi"("error in (no error)"=w949, "Output"=w944, "MotorControlDevRef"=w950) -> ()  [unwired: 6 in, 3 out]
                  n479 = And(x=w952, y=w951) -> (x .and. y?=w939:bool)
                  n480 = And(x=w942, y=w941) -> (x .and. y?=w940:bool)
                  n481 = And(x=w939, y=w940) -> (x .and. y?=w938:bool)
                }
              }
            }
            n482 = call <vilib>:"WPI_RobotDriveDelayAndUpdateSafety.vi"("error in (no error)"=w830, "Delay (s)"=w832, "RobotDriveDevRef"=w831) -> ("RobotDriveDevRef 2"=w835:T4)  [unwired: 7 in, 1 out]
          }
        }
        frame "RLR" {
          n483 = Array Size(array="Center RLR") -> (size(s)=w962:i32)
          n484 = call <vilib>:"WPI_RobotDriveRefNum Registry Get.vi"("refnum name"="Left and Right Motors") -> ("RobotDriveDevRef"=w961:T4)  [unwired: 1 in, 9 out]
          n485 = for {
            N: w962 -> [_]
            shift-right: [w970] -> _
            shift-left: w961 -> [w969]
            tunnel: "Center RLR" -> [w968] mode=indexing
            i -> [w964]
            n486 = global write "Robot Global Data.vi" "Array Step"(w964) -> ()
            n487 = while {
              shift-right: [w998] -> w966
              shift-left: w969 -> [w997]
              tunnel: w968 -> [w994]
              tunnel: [w975] -> w967
              tunnel: [w978] -> w965
              stop <- w979 stop-if-true
              n488 = global read "Robot Global Data.vi" "Right Distance"() -> (w982:dbl)
              n489 = global read "Robot Global Data.vi" "Lift Distance"() -> (w973:dbl)
              n490 = global read "Robot Global Data.vi" "Left Distance"() -> (w981:dbl)
              n491 = Unbundle By Name(w994) -> ("Left Joystick"=w993:dbl, "Right Joystick"=w992:dbl, "Duration"=w980:dbl, "SOL A"=w991:bool, "SOL B"=w990:bool, "Lift Up"=w989:bool, "Lift Down"=w988:bool, "Intake In"=w987:bool, "Intake Out"=w986:bool, "Wrist Up"=w985:bool, "Wrist Down"=w984:bool, "Left Distance"=w974:dbl, "Right Distance"=w983:dbl, "Drive?"=w977:bool, "Lift Target"=w972:dbl, "Wrist Target"=w971:dbl)
              n492 = global read "Robot Global Data.vi" "Wrist Angle"() -> (w976:dbl)
              n493 = global read "Robot Global Data.vi" "Left Rate"() -> (w996:dbl)
              n494 = global read "Robot Global Data.vi" "Right Rate"() -> (w995:dbl)
              n495 = case shown="True" w977 {
                tunnel: [w1071 w1089] -> w998
                tunnel: w997 -> [w1070 w1090]
                tunnel: w996 -> [_ _]
                tunnel: w995 -> [_ _]
                tunnel: w993 -> [w1028 _]
                tunnel: w992 -> [w1029 _]
                tunnel: w991 -> [w1053 _]
                tunnel: w990 -> [w1052 _]
                tunnel: w989 -> [w1011 _]
                tunnel: w988 -> [w1010 _]
                tunnel: w987 -> [w1033 _]
                tunnel: w986 -> [_ w1080]
                tunnel: w985 -> [w1009 _]
                tunnel: w984 -> [w1008 _]
                tunnel: w974 -> [w1032 _]
                tunnel: w983 -> [w1051 _]
                tunnel: w982 -> [w1050 _]
                tunnel: w981 -> [w1049 _]
                tunnel: w980 -> [w1047 w1078]
                tunnel: [w1030 w1078] -> w975
                tunnel: [w1015 w1073] -> w979
                tunnel: [w1046 w1088] -> w978
                tunnel: w976 -> [w1022 _]
                tunnel: w973 -> [w1023 _]
                tunnel: w972 -> [w1027 _]
                tunnel: w971 -> [w1021 _]
                frame True {
                  w1014 = FALSE ("Left Reset")
                  n496 = Greater Or Equal?(x=w1022, y=w1021) -> (x >= y?=w1004:bool)
                  n497 = Select(t=-1.0, s=w1008, f=0.1) -> (s? t:f=w1036:dbl)
                  n498 = Greater Or Equal?(x=w1023, y=w1027) -> (x >= y?=w1006:bool)
                  n499 = Greater Or Equal?(x=w1049, y=w1032) -> (x >= y?=w999:bool)
                  n500 = Greater Or Equal?(x=w1050, y=w1051) -> (x >= y?=w1000:bool)
                  n501 = Select(t=1.0, s=w1009, f=w1036) -> (s? t:f=w1019:dbl)
                  n502 = Select(t=-1.0, s=w1010, f=0.1) -> (s? t:f=w1035:dbl)
                  n503 = Select(t=1.0, s=w1011, f=w1035) -> (s? t:f=w1025:dbl)
                  n504 = Select(t=0.0, s=w1004, f=w1019) -> (s? t:f=w1018:dbl)
                  n505 = Select(t=1.0, s=w1033, f=0.0) -> (s? t:f=w1034:dbl)
                  n506 = Not Or(1:w1010, 2:w1011) -> (0:w1007:bool)
                  n507 = Not Or(1:w1008, 2:w1009) -> (0:w1005:bool)
                  n508 = Select(t=0.0, s=w1006, f=w1025) -> (s? t:f=w1024:dbl)
                  n509 = call <vilib>:"WPI_MotorControlRefNum Registry Get.vi"("refnum name"="Wrist") -> ("error out"=w1057:errorcluster, "MotorControlDevRef"=w1058:T5)  [unwired: 9 in]
                  n510 = call <vilib>:"WPI_SolenoidRefNum Registry Get.vi"("refnum name"="SOL A") -> ("error out"=w1066:errorcluster, "SolenoidDevRef"=w1067:T10)  [unwired: 9 in]
                  n511 = call <vilib>:"WPI_SolenoidRefNum Registry Get.vi"("refnum name"="SOL B") -> ("error out"=w1063:errorcluster, "SolenoidDevRef"=w1064:T10)  [unwired: 9 in]
                  n512 = call <vilib>:"WPI_MotorControlRefNum Registry Get.vi"("refnum name"="Intake") -> ("error out"=w1059:errorcluster, "MotorControlDevRef"=w1060:T5)  [unwired: 9 in]
                  n513 = call <vilib>:"WPI_MotorControlRefNum Registry Get.vi"("refnum name"="Lift") -> ("error out"=w1061:errorcluster, "MotorControlDevRef"=w1062:T5)  [unwired: 9 in]
                  n514 = call <vilib>:"WPI_MotorControlSetOutput.vi"("error in (no error)"=w1057, "Output"=w1018, "MotorControlDevRef"=w1058) -> ()  [unwired: 6 in, 3 out]
                  n515 = call-poly <vilib>:"WPI_SolenoidSet.vi"("error in (no error)"=w1066, "Value"=w1053, "SolenoidDevRef"=w1067) -> ()  [unwired: 7 in, 2 out]
                  n516 = call-poly <vilib>:"WPI_SolenoidSet.vi"("error in (no error)"=w1063, "Value"=w1052, "SolenoidDevRef"=w1064) -> ()  [unwired: 7 in, 2 out]
                  n517 = Or(x=w1007, y=w1006) -> (x .or. y?=w1003:bool)
                  n518 = Or(x=w1005, y=w1004) -> (x .or. y?=w1002:bool)
                  n519 = call <vilib>:"WPI_MotorControlSetOutput.vi"("error in (no error)"=w1059, "Output"=w1034, "MotorControlDevRef"=w1060) -> ()  [unwired: 6 in, 3 out]
                  n520 = call <vilib>:"WPI_MotorControlSetOutput.vi"("error in (no error)"=w1061, "Output"=w1024, "MotorControlDevRef"=w1062) -> ()  [unwired: 6 in, 3 out]
                  n521 = And(x=w1003, y=w1002) -> (x .and. y?=w1001:bool)
                  n522 = Select(t=0.0, s=w1000, f=w1029) -> (s? t:f=w1012:dbl)
                  n523 = Select(t=0.0, s=w999, f=w1028) -> (s? t:f=w1013:dbl)
                  n524 = call <vilib>:"WPI_RobotDriveTankDrive.vi"("Right axis value"=w1012, "Left axis value"=w1013, "RobotDriveDevRef"=w1070) -> ("error out"=w1046:errorcluster, "Motor Values"=w1031:dbl[], "RobotDriveDevRef"=w1071:T4)  [unwired: 6 in]
                  n525 = global write "Robot Global Data.vi" "Wrist Reset"(w1014) -> ()
                  n526 = global write "Robot Global Data.vi" "Left Reset"(w1014) -> ()
                  n527 = global write "Robot Global Data.vi" "Right Reset"(w1014) -> ()
                  n528 = global write "Robot Global Data.vi" "Lift Reset"(w1014) -> ()
                  n529 = And(x=w999, y=w1000) -> (x .and. y?=w1016:bool)
                  n530 = And(x=w1001, y=w1016) -> (x .and. y?=w1015:bool)
                  n531 = call-poly <vilib>:"NT Write Value.vi"("Numeric Array"=w1031, "Name"="RobotDrive Motors") -> ()  [unwired: 9 in, 1 out]
                  n532 = Select(t=0.0, s=w1015, f=w1047) -> (s? t:f=w1030:dbl)
                }
                frame False {
                  w1072 = TRUE ("Left Reset")
                  n533 = Select(t=-1.0, s=w1080, f=0.0) -> (s? t:f=w1079:dbl)
                  n534 = global write "Robot Global Data.vi" "Wrist Reset"(w1072) -> ()
                  n535 = global write "Robot Global Data.vi" "Left Reset"(w1072) -> ()
                  n536 = global write "Robot Global Data.vi" "Right Reset"(w1072) -> ()
                  n537 = global write "Robot Global Data.vi" "Lift Reset"(w1072) -> ()
                  n538 = call <vilib>:"WPI_RobotDriveTankDrive.vi"("Right axis value"=0.0, "Left axis value"=0.0, "RobotDriveDevRef"=w1090) -> ("error out"=w1088:errorcluster, "Motor Values"=w1093:dbl[], "RobotDriveDevRef"=w1089:T4)  [unwired: 6 in]
                  n539 = Wait (ms)(milliseconds to wait=w1078) -> ()  [unwired: 1 out]
                  n540 = call <vilib>:"WPI_MotorControlRefNum Registry Get.vi"("refnum name"="Intake") -> ("error out"=w1084:errorcluster, "MotorControlDevRef"=w1085:T5)  [unwired: 9 in]
                  n541 = call-poly <vilib>:"NT Write Value.vi"("Numeric Array"=w1093, "Name"="RobotDrive Motors") -> ()  [unwired: 9 in, 1 out]
                  n542 = global read "Robot Global Data.vi" "Wrist Reset"() -> (w1076:bool)
                  n543 = global read "Robot Global Data.vi" "Right Reset"() -> (w1086:bool)
                  n544 = global read "Robot Global Data.vi" "Lift Reset"() -> (w1077:bool)
                  n545 = global read "Robot Global Data.vi" "Left Reset"() -> (w1087:bool)
                  n546 = call <vilib>:"WPI_MotorControlSetOutput.vi"("error in (no error)"=w1084, "Output"=w1079, "MotorControlDevRef"=w1085) -> ()  [unwired: 6 in, 3 out]
                  n547 = And(x=w1087, y=w1086) -> (x .and. y?=w1074:bool)
                  n548 = And(x=w1077, y=w1076) -> (x .and. y?=w1075:bool)
                  n549 = And(x=w1074, y=w1075) -> (x .and. y?=w1073:bool)
                }
              }
            }
            n550 = call <vilib>:"WPI_RobotDriveDelayAndUpdateSafety.vi"("error in (no error)"=w965, "Delay (s)"=w967, "RobotDriveDevRef"=w966) -> ("RobotDriveDevRef 2"=w970:T4)  [unwired: 7 in, 1 out]
          }
        }
        frame "LLL", Default {
          n551 = Array Size(array="Center LLL") -> (size(s)=w1096:i32)
          n552 = call <vilib>:"WPI_RobotDriveRefNum Registry Get.vi"("refnum name"="Left and Right Motors") -> ("RobotDriveDevRef"=w1097:T4)  [unwired: 1 in, 9 out]
          n553 = for {
            N: w1096 -> [_]
            shift-right: [w1105] -> _
            shift-left: w1097 -> [w1104]
            tunnel: "Center LLL" -> [w1103] mode=indexing
            i -> [w1099]
            n554 = global write "Robot Global Data.vi" "Array Step"(w1099) -> ()
            n555 = while {
              shift-right: [w1133] -> w1101
              shift-left: w1104 -> [w1132]
              tunnel: w1103 -> [w1129]
              tunnel: [w1110] -> w1102
              tunnel: [w1113] -> w1100
              stop <- w1114 stop-if-true
              n556 = global read "Robot Global Data.vi" "Right Distance"() -> (w1117:dbl)
              n557 = global read "Robot Global Data.vi" "Lift Distance"() -> (w1108:dbl)
              n558 = global read "Robot Global Data.vi" "Left Distance"() -> (w1116:dbl)
              n559 = Unbundle By Name(w1129) -> ("Left Joystick"=w1128:dbl, "Right Joystick"=w1127:dbl, "Duration"=w1115:dbl, "SOL A"=w1126:bool, "SOL B"=w1125:bool, "Lift Up"=w1124:bool, "Lift Down"=w1123:bool, "Intake In"=w1122:bool, "Intake Out"=w1121:bool, "Wrist Up"=w1120:bool, "Wrist Down"=w1119:bool, "Left Distance"=w1109:dbl, "Right Distance"=w1118:dbl, "Drive?"=w1112:bool, "Lift Target"=w1107:dbl, "Wrist Target"=w1106:dbl)
              n560 = global read "Robot Global Data.vi" "Wrist Angle"() -> (w1111:dbl)
              n561 = global read "Robot Global Data.vi" "Left Rate"() -> (w1131:dbl)
              n562 = global read "Robot Global Data.vi" "Right Rate"() -> (w1130:dbl)
              n563 = case shown="True" w1112 {
                tunnel: [w1206 w1224] -> w1133
                tunnel: w1132 -> [w1205 w1225]
                tunnel: w1131 -> [_ _]
                tunnel: w1130 -> [_ _]
                tunnel: w1128 -> [w1163 _]
                tunnel: w1127 -> [w1164 _]
                tunnel: w1126 -> [w1188 _]
                tunnel: w1125 -> [w1187 _]
                tunnel: w1124 -> [w1146 _]
                tunnel: w1123 -> [w1145 _]
                tunnel: w1122 -> [w1168 _]
                tunnel: w1121 -> [_ w1215]
                tunnel: w1120 -> [w1144 _]
                tunnel: w1119 -> [w1143 _]
                tunnel: w1109 -> [w1167 _]
                tunnel: w1118 -> [w1186 _]
                tunnel: w1117 -> [w1185 _]
                tunnel: w1116 -> [w1184 _]
                tunnel: w1115 -> [w1182 w1213]
                tunnel: [w1165 w1213] -> w1110
                tunnel: [w1150 w1208] -> w1114
                tunnel: [w1181 w1223] -> w1113
                tunnel: w1111 -> [w1157 _]
                tunnel: w1108 -> [w1158 _]
                tunnel: w1107 -> [w1162 _]
                tunnel: w1106 -> [w1156 _]
                frame True {
                  w1149 = FALSE ("Left Reset")
                  n564 = Greater Or Equal?(x=w1157, y=w1156) -> (x >= y?=w1139:bool)
                  n565 = Select(t=-1.0, s=w1143, f=0.1) -> (s? t:f=w1171:dbl)
                  n566 = Greater Or Equal?(x=w1158, y=w1162) -> (x >= y?=w1141:bool)
                  n567 = Greater Or Equal?(x=w1184, y=w1167) -> (x >= y?=w1134:bool)
                  n568 = Greater Or Equal?(x=w1185, y=w1186) -> (x >= y?=w1135:bool)
                  n569 = Select(t=1.0, s=w1144, f=w1171) -> (s? t:f=w1154:dbl)
                  n570 = Select(t=-1.0, s=w1145, f=0.1) -> (s? t:f=w1170:dbl)
                  n571 = Select(t=1.0, s=w1146, f=w1170) -> (s? t:f=w1160:dbl)
                  n572 = Select(t=0.0, s=w1139, f=w1154) -> (s? t:f=w1153:dbl)
                  n573 = Select(t=1.0, s=w1168, f=0.0) -> (s? t:f=w1169:dbl)
                  n574 = Not Or(1:w1145, 2:w1146) -> (0:w1142:bool)
                  n575 = Not Or(1:w1143, 2:w1144) -> (0:w1140:bool)
                  n576 = Select(t=0.0, s=w1141, f=w1160) -> (s? t:f=w1159:dbl)
                  n577 = call <vilib>:"WPI_MotorControlRefNum Registry Get.vi"("refnum name"="Wrist") -> ("error out"=w1192:errorcluster, "MotorControlDevRef"=w1193:T5)  [unwired: 9 in]
                  n578 = call <vilib>:"WPI_SolenoidRefNum Registry Get.vi"("refnum name"="SOL A") -> ("error out"=w1201:errorcluster, "SolenoidDevRef"=w1202:T10)  [unwired: 9 in]
                  n579 = call <vilib>:"WPI_SolenoidRefNum Registry Get.vi"("refnum name"="SOL B") -> ("error out"=w1198:errorcluster, "SolenoidDevRef"=w1199:T10)  [unwired: 9 in]
                  n580 = call <vilib>:"WPI_MotorControlRefNum Registry Get.vi"("refnum name"="Intake") -> ("error out"=w1194:errorcluster, "MotorControlDevRef"=w1195:T5)  [unwired: 9 in]
                  n581 = call <vilib>:"WPI_MotorControlRefNum Registry Get.vi"("refnum name"="Lift") -> ("error out"=w1196:errorcluster, "MotorControlDevRef"=w1197:T5)  [unwired: 9 in]
                  n582 = call <vilib>:"WPI_MotorControlSetOutput.vi"("error in (no error)"=w1192, "Output"=w1153, "MotorControlDevRef"=w1193) -> ()  [unwired: 6 in, 3 out]
                  n583 = call-poly <vilib>:"WPI_SolenoidSet.vi"("error in (no error)"=w1201, "Value"=w1188, "SolenoidDevRef"=w1202) -> ()  [unwired: 7 in, 2 out]
                  n584 = call-poly <vilib>:"WPI_SolenoidSet.vi"("error in (no error)"=w1198, "Value"=w1187, "SolenoidDevRef"=w1199) -> ()  [unwired: 7 in, 2 out]
                  n585 = Or(x=w1142, y=w1141) -> (x .or. y?=w1138:bool)
                  n586 = Or(x=w1140, y=w1139) -> (x .or. y?=w1137:bool)
                  n587 = call <vilib>:"WPI_MotorControlSetOutput.vi"("error in (no error)"=w1194, "Output"=w1169, "MotorControlDevRef"=w1195) -> ()  [unwired: 6 in, 3 out]
                  n588 = call <vilib>:"WPI_MotorControlSetOutput.vi"("error in (no error)"=w1196, "Output"=w1159, "MotorControlDevRef"=w1197) -> ()  [unwired: 6 in, 3 out]
                  n589 = And(x=w1138, y=w1137) -> (x .and. y?=w1136:bool)
                  n590 = Select(t=0.0, s=w1135, f=w1164) -> (s? t:f=w1147:dbl)
                  n591 = Select(t=0.0, s=w1134, f=w1163) -> (s? t:f=w1148:dbl)
                  n592 = call <vilib>:"WPI_RobotDriveTankDrive.vi"("Right axis value"=w1147, "Left axis value"=w1148, "RobotDriveDevRef"=w1205) -> ("error out"=w1181:errorcluster, "Motor Values"=w1166:dbl[], "RobotDriveDevRef"=w1206:T4)  [unwired: 6 in]
                  n593 = global write "Robot Global Data.vi" "Wrist Reset"(w1149) -> ()
                  n594 = global write "Robot Global Data.vi" "Left Reset"(w1149) -> ()
                  n595 = global write "Robot Global Data.vi" "Right Reset"(w1149) -> ()
                  n596 = global write "Robot Global Data.vi" "Lift Reset"(w1149) -> ()
                  n597 = And(x=w1134, y=w1135) -> (x .and. y?=w1151:bool)
                  n598 = And(x=w1136, y=w1151) -> (x .and. y?=w1150:bool)
                  n599 = call-poly <vilib>:"NT Write Value.vi"("Numeric Array"=w1166, "Name"="RobotDrive Motors") -> ()  [unwired: 9 in, 1 out]
                  n600 = Select(t=0.0, s=w1150, f=w1182) -> (s? t:f=w1165:dbl)
                }
                frame False {
                  w1207 = TRUE ("Left Reset")
                  n601 = Select(t=-1.0, s=w1215, f=0.0) -> (s? t:f=w1214:dbl)
                  n602 = global write "Robot Global Data.vi" "Wrist Reset"(w1207) -> ()
                  n603 = global write "Robot Global Data.vi" "Left Reset"(w1207) -> ()
                  n604 = global write "Robot Global Data.vi" "Right Reset"(w1207) -> ()
                  n605 = global write "Robot Global Data.vi" "Lift Reset"(w1207) -> ()
                  n606 = call <vilib>:"WPI_RobotDriveTankDrive.vi"("Right axis value"=0.0, "Left axis value"=0.0, "RobotDriveDevRef"=w1225) -> ("error out"=w1223:errorcluster, "Motor Values"=w1228:dbl[], "RobotDriveDevRef"=w1224:T4)  [unwired: 6 in]
                  n607 = Wait (ms)(milliseconds to wait=w1213) -> ()  [unwired: 1 out]
                  n608 = call <vilib>:"WPI_MotorControlRefNum Registry Get.vi"("refnum name"="Intake") -> ("error out"=w1219:errorcluster, "MotorControlDevRef"=w1220:T5)  [unwired: 9 in]
                  n609 = call-poly <vilib>:"NT Write Value.vi"("Numeric Array"=w1228, "Name"="RobotDrive Motors") -> ()  [unwired: 9 in, 1 out]
                  n610 = global read "Robot Global Data.vi" "Wrist Reset"() -> (w1211:bool)
                  n611 = global read "Robot Global Data.vi" "Right Reset"() -> (w1221:bool)
                  n612 = global read "Robot Global Data.vi" "Lift Reset"() -> (w1212:bool)
                  n613 = global read "Robot Global Data.vi" "Left Reset"() -> (w1222:bool)
                  n614 = call <vilib>:"WPI_MotorControlSetOutput.vi"("error in (no error)"=w1219, "Output"=w1214, "MotorControlDevRef"=w1220) -> ()  [unwired: 6 in, 3 out]
                  n615 = And(x=w1222, y=w1221) -> (x .and. y?=w1209:bool)
                  n616 = And(x=w1212, y=w1211) -> (x .and. y?=w1210:bool)
                  n617 = And(x=w1209, y=w1210) -> (x .and. y?=w1208:bool)
                }
              }
            }
            n618 = call <vilib>:"WPI_RobotDriveDelayAndUpdateSafety.vi"("error in (no error)"=w1100, "Delay (s)"=w1102, "RobotDriveDevRef"=w1101) -> ("RobotDriveDevRef 2"=w1105:T4)  [unwired: 7 in, 1 out]
          }
        }
      }
    }
    frame "Starting Right" {
      n619 = case shown="\"LRL\"" w1230 {
        frame "RRR" {
          n620 = Array Size(array="Right RRR") -> (size(s)=w1232:i32)
          n621 = call <vilib>:"WPI_RobotDriveRefNum Registry Get.vi"("refnum name"="Left and Right Motors") -> ("RobotDriveDevRef"=w1233:T4)  [unwired: 1 in, 9 out]
          n622 = for {
            N: w1232 -> [_]
            shift-right: [w1241] -> _
            shift-left: w1233 -> [w1240]
            tunnel: "Right RRR" -> [w1239] mode=indexing
            i -> [w1235]
            n623 = global write "Robot Global Data.vi" "Array Step"(w1235) -> ()
            n624 = while {
              shift-right: [w1269] -> w1237
              shift-left: w1240 -> [w1268]
              tunnel: w1239 -> [w1265]
              tunnel: [w1246] -> w1238
              tunnel: [w1249] -> w1236
              stop <- w1250 stop-if-true
              n625 = global read "Robot Global Data.vi" "Right Distance"() -> (w1253:dbl)
              n626 = global read "Robot Global Data.vi" "Lift Distance"() -> (w1244:dbl)
              n627 = global read "Robot Global Data.vi" "Left Distance"() -> (w1252:dbl)
              n628 = Unbundle By Name(w1265) -> ("Left Joystick"=w1264:dbl, "Right Joystick"=w1263:dbl, "Duration"=w1251:dbl, "SOL A"=w1262:bool, "SOL B"=w1261:bool, "Lift Up"=w1260:bool, "Lift Down"=w1259:bool, "Intake In"=w1258:bool, "Intake Out"=w1257:bool, "Wrist Up"=w1256:bool, "Wrist Down"=w1255:bool, "Left Distance"=w1245:dbl, "Right Distance"=w1254:dbl, "Drive?"=w1248:bool, "Lift Target"=w1243:dbl, "Wrist Target"=w1242:dbl)
              n629 = global read "Robot Global Data.vi" "Wrist Angle"() -> (w1247:dbl)
              n630 = global read "Robot Global Data.vi" "Left Rate"() -> (w1267:dbl)
              n631 = global read "Robot Global Data.vi" "Right Rate"() -> (w1266:dbl)
              n632 = case shown="True" w1248 {
                tunnel: [w1342 w1360] -> w1269
                tunnel: w1268 -> [w1341 w1361]
                tunnel: w1267 -> [_ _]
                tunnel: w1266 -> [_ _]
                tunnel: w1264 -> [w1299 _]
                tunnel: w1263 -> [w1300 _]
                tunnel: w1262 -> [w1324 _]
                tunnel: w1261 -> [w1323 _]
                tunnel: w1260 -> [w1282 _]
                tunnel: w1259 -> [w1281 _]
                tunnel: w1258 -> [w1304 _]
                tunnel: w1257 -> [_ w1351]
                tunnel: w1256 -> [w1280 _]
                tunnel: w1255 -> [w1279 _]
                tunnel: w1245 -> [w1303 _]
                tunnel: w1254 -> [w1322 _]
                tunnel: w1253 -> [w1321 _]
                tunnel: w1252 -> [w1320 _]
                tunnel: w1251 -> [w1318 w1349]
                tunnel: [w1301 w1349] -> w1246
                tunnel: [w1286 w1344] -> w1250
                tunnel: [w1317 w1359] -> w1249
                tunnel: w1247 -> [w1293 _]
                tunnel: w1244 -> [w1294 _]
                tunnel: w1243 -> [w1298 _]
                tunnel: w1242 -> [w1292 _]
                frame True {
                  w1285 = FALSE ("Left Reset")
                  n633 = Greater Or Equal?(x=w1293, y=w1292) -> (x >= y?=w1275:bool)
                  n634 = Select(t=-1.0, s=w1279, f=0.1) -> (s? t:f=w1307:dbl)
                  n635 = Greater Or Equal?(x=w1294, y=w1298) -> (x >= y?=w1277:bool)
                  n636 = Greater Or Equal?(x=w1320, y=w1303) -> (x >= y?=w1270:bool)
                  n637 = Greater Or Equal?(x=w1321, y=w1322) -> (x >= y?=w1271:bool)
                  n638 = Select(t=1.0, s=w1280, f=w1307) -> (s? t:f=w1290:dbl)
                  n639 = Select(t=-1.0, s=w1281, f=0.1) -> (s? t:f=w1306:dbl)
                  n640 = Select(t=1.0, s=w1282, f=w1306) -> (s? t:f=w1296:dbl)
                  n641 = Select(t=0.0, s=w1275, f=w1290) -> (s? t:f=w1289:dbl)
                  n642 = Select(t=1.0, s=w1304, f=0.0) -> (s? t:f=w1305:dbl)
                  n643 = Not Or(1:w1281, 2:w1282) -> (0:w1278:bool)
                  n644 = Not Or(1:w1279, 2:w1280) -> (0:w1276:bool)
                  n645 = Select(t=0.0, s=w1277, f=w1296) -> (s? t:f=w1295:dbl)
                  n646 = call <vilib>:"WPI_MotorControlRefNum Registry Get.vi"("refnum name"="Wrist") -> ("error out"=w1328:errorcluster, "MotorControlDevRef"=w1329:T5)  [unwired: 9 in]
                  n647 = call <vilib>:"WPI_SolenoidRefNum Registry Get.vi"("refnum name"="SOL A") -> ("error out"=w1337:errorcluster, "SolenoidDevRef"=w1338:T10)  [unwired: 9 in]
                  n648 = call <vilib>:"WPI_SolenoidRefNum Registry Get.vi"("refnum name"="SOL B") -> ("error out"=w1334:errorcluster, "SolenoidDevRef"=w1335:T10)  [unwired: 9 in]
                  n649 = call <vilib>:"WPI_MotorControlRefNum Registry Get.vi"("refnum name"="Intake") -> ("error out"=w1330:errorcluster, "MotorControlDevRef"=w1331:T5)  [unwired: 9 in]
                  n650 = call <vilib>:"WPI_MotorControlRefNum Registry Get.vi"("refnum name"="Lift") -> ("error out"=w1332:errorcluster, "MotorControlDevRef"=w1333:T5)  [unwired: 9 in]
                  n651 = call <vilib>:"WPI_MotorControlSetOutput.vi"("error in (no error)"=w1328, "Output"=w1289, "MotorControlDevRef"=w1329) -> ()  [unwired: 6 in, 3 out]
                  n652 = call-poly <vilib>:"WPI_SolenoidSet.vi"("error in (no error)"=w1337, "Value"=w1324, "SolenoidDevRef"=w1338) -> ()  [unwired: 7 in, 2 out]
                  n653 = call-poly <vilib>:"WPI_SolenoidSet.vi"("error in (no error)"=w1334, "Value"=w1323, "SolenoidDevRef"=w1335) -> ()  [unwired: 7 in, 2 out]
                  n654 = Or(x=w1278, y=w1277) -> (x .or. y?=w1274:bool)
                  n655 = Or(x=w1276, y=w1275) -> (x .or. y?=w1273:bool)
                  n656 = call <vilib>:"WPI_MotorControlSetOutput.vi"("error in (no error)"=w1330, "Output"=w1305, "MotorControlDevRef"=w1331) -> ()  [unwired: 6 in, 3 out]
                  n657 = call <vilib>:"WPI_MotorControlSetOutput.vi"("error in (no error)"=w1332, "Output"=w1295, "MotorControlDevRef"=w1333) -> ()  [unwired: 6 in, 3 out]
                  n658 = And(x=w1274, y=w1273) -> (x .and. y?=w1272:bool)
                  n659 = Select(t=0.0, s=w1271, f=w1300) -> (s? t:f=w1283:dbl)
                  n660 = Select(t=0.0, s=w1270, f=w1299) -> (s? t:f=w1284:dbl)
                  n661 = call <vilib>:"WPI_RobotDriveTankDrive.vi"("Right axis value"=w1283, "Left axis value"=w1284, "RobotDriveDevRef"=w1341) -> ("error out"=w1317:errorcluster, "Motor Values"=w1302:dbl[], "RobotDriveDevRef"=w1342:T4)  [unwired: 6 in]
                  n662 = global write "Robot Global Data.vi" "Wrist Reset"(w1285) -> ()
                  n663 = global write "Robot Global Data.vi" "Left Reset"(w1285) -> ()
                  n664 = global write "Robot Global Data.vi" "Right Reset"(w1285) -> ()
                  n665 = global write "Robot Global Data.vi" "Lift Reset"(w1285) -> ()
                  n666 = And(x=w1270, y=w1271) -> (x .and. y?=w1287:bool)
                  n667 = And(x=w1272, y=w1287) -> (x .and. y?=w1286:bool)
                  n668 = call-poly <vilib>:"NT Write Value.vi"("Numeric Array"=w1302, "Name"="RobotDrive Motors") -> ()  [unwired: 9 in, 1 out]
                  n669 = Select(t=0.0, s=w1286, f=w1318) -> (s? t:f=w1301:dbl)
                }
                frame False {
                  w1343 = TRUE ("Left Reset")
                  n670 = Select(t=-1.0, s=w1351, f=0.0) -> (s? t:f=w1350:dbl)
                  n671 = global write "Robot Global Data.vi" "Wrist Reset"(w1343) -> ()
                  n672 = global write "Robot Global Data.vi" "Left Reset"(w1343) -> ()
                  n673 = global write "Robot Global Data.vi" "Right Reset"(w1343) -> ()
                  n674 = global write "Robot Global Data.vi" "Lift Reset"(w1343) -> ()
                  n675 = call <vilib>:"WPI_RobotDriveTankDrive.vi"("Right axis value"=0.0, "Left axis value"=0.0, "RobotDriveDevRef"=w1361) -> ("error out"=w1359:errorcluster, "Motor Values"=w1364:dbl[], "RobotDriveDevRef"=w1360:T4)  [unwired: 6 in]
                  n676 = Wait (ms)(milliseconds to wait=w1349) -> ()  [unwired: 1 out]
                  n677 = call <vilib>:"WPI_MotorControlRefNum Registry Get.vi"("refnum name"="Intake") -> ("error out"=w1355:errorcluster, "MotorControlDevRef"=w1356:T5)  [unwired: 9 in]
                  n678 = call-poly <vilib>:"NT Write Value.vi"("Numeric Array"=w1364, "Name"="RobotDrive Motors") -> ()  [unwired: 9 in, 1 out]
                  n679 = global read "Robot Global Data.vi" "Wrist Reset"() -> (w1347:bool)
                  n680 = global read "Robot Global Data.vi" "Right Reset"() -> (w1357:bool)
                  n681 = global read "Robot Global Data.vi" "Lift Reset"() -> (w1348:bool)
                  n682 = global read "Robot Global Data.vi" "Left Reset"() -> (w1358:bool)
                  n683 = call <vilib>:"WPI_MotorControlSetOutput.vi"("error in (no error)"=w1355, "Output"=w1350, "MotorControlDevRef"=w1356) -> ()  [unwired: 6 in, 3 out]
                  n684 = And(x=w1358, y=w1357) -> (x .and. y?=w1345:bool)
                  n685 = And(x=w1348, y=w1347) -> (x .and. y?=w1346:bool)
                  n686 = And(x=w1345, y=w1346) -> (x .and. y?=w1344:bool)
                }
              }
            }
            n687 = call <vilib>:"WPI_RobotDriveDelayAndUpdateSafety.vi"("error in (no error)"=w1236, "Delay (s)"=w1238, "RobotDriveDevRef"=w1237) -> ("RobotDriveDevRef 2"=w1241:T4)  [unwired: 7 in, 1 out]
          }
        }
        frame "LRL" {
          n688 = Array Size(array="Right LRL") -> (size(s)=w1367:i32)
          n689 = call <vilib>:"WPI_RobotDriveRefNum Registry Get.vi"("refnum name"="Left and Right Motors") -> ("RobotDriveDevRef"=w1368:T4)  [unwired: 1 in, 9 out]
          n690 = for {
            N: w1367 -> [_]
            shift-right: [w1376] -> _
            shift-left: w1368 -> [w1375]
            tunnel: "Right LRL" -> [w1374] mode=indexing
            i -> [w1370]
            n691 = global write "Robot Global Data.vi" "Array Step"(w1370) -> ()
            n692 = while {
              shift-right: [w1404] -> w1372
              shift-left: w1375 -> [w1403]
              tunnel: w1374 -> [w1400]
              tunnel: [w1381] -> w1373
              tunnel: [w1384] -> w1371
              stop <- w1385 stop-if-true
              n693 = global read "Robot Global Data.vi" "Right Distance"() -> (w1388:dbl)
              n694 = global read "Robot Global Data.vi" "Lift Distance"() -> (w1379:dbl)
              n695 = global read "Robot Global Data.vi" "Left Distance"() -> (w1387:dbl)
              n696 = Unbundle By Name(w1400) -> ("Left Joystick"=w1399:dbl, "Right Joystick"=w1398:dbl, "Duration"=w1386:dbl, "SOL A"=w1397:bool, "SOL B"=w1396:bool, "Lift Up"=w1395:bool, "Lift Down"=w1394:bool, "Intake In"=w1393:bool, "Intake Out"=w1392:bool, "Wrist Up"=w1391:bool, "Wrist Down"=w1390:bool, "Left Distance"=w1380:dbl, "Right Distance"=w1389:dbl, "Drive?"=w1383:bool, "Lift Target"=w1378:dbl, "Wrist Target"=w1377:dbl)
              n697 = global read "Robot Global Data.vi" "Wrist Angle"() -> (w1382:dbl)
              n698 = global read "Robot Global Data.vi" "Left Rate"() -> (w1402:dbl)
              n699 = global read "Robot Global Data.vi" "Right Rate"() -> (w1401:dbl)
              n700 = case shown="True" w1383 {
                tunnel: [w1477 w1495] -> w1404
                tunnel: w1403 -> [w1476 w1496]
                tunnel: w1402 -> [_ _]
                tunnel: w1401 -> [_ _]
                tunnel: w1399 -> [w1434 _]
                tunnel: w1398 -> [w1435 _]
                tunnel: w1397 -> [w1459 _]
                tunnel: w1396 -> [w1458 _]
                tunnel: w1395 -> [w1417 _]
                tunnel: w1394 -> [w1416 _]
                tunnel: w1393 -> [w1439 _]
                tunnel: w1392 -> [_ w1486]
                tunnel: w1391 -> [w1415 _]
                tunnel: w1390 -> [w1414 _]
                tunnel: w1380 -> [w1438 _]
                tunnel: w1389 -> [w1457 _]
                tunnel: w1388 -> [w1456 _]
                tunnel: w1387 -> [w1455 _]
                tunnel: w1386 -> [w1453 w1484]
                tunnel: [w1436 w1484] -> w1381
                tunnel: [w1421 w1479] -> w1385
                tunnel: [w1452 w1494] -> w1384
                tunnel: w1382 -> [w1428 _]
                tunnel: w1379 -> [w1429 _]
                tunnel: w1378 -> [w1433 _]
                tunnel: w1377 -> [w1427 _]
                frame True {
                  w1420 = FALSE ("Left Reset")
                  n701 = Greater Or Equal?(x=w1428, y=w1427) -> (x >= y?=w1410:bool)
                  n702 = Select(t=-1.0, s=w1414, f=0.1) -> (s? t:f=w1442:dbl)
                  n703 = Greater Or Equal?(x=w1429, y=w1433) -> (x >= y?=w1412:bool)
                  n704 = Greater Or Equal?(x=w1455, y=w1438) -> (x >= y?=w1405:bool)
                  n705 = Greater Or Equal?(x=w1456, y=w1457) -> (x >= y?=w1406:bool)
                  n706 = Select(t=1.0, s=w1415, f=w1442) -> (s? t:f=w1425:dbl)
                  n707 = Select(t=-1.0, s=w1416, f=0.1) -> (s? t:f=w1441:dbl)
                  n708 = Select(t=1.0, s=w1417, f=w1441) -> (s? t:f=w1431:dbl)
                  n709 = Select(t=0.0, s=w1410, f=w1425) -> (s? t:f=w1424:dbl)
                  n710 = Select(t=1.0, s=w1439, f=0.0) -> (s? t:f=w1440:dbl)
                  n711 = Not Or(1:w1416, 2:w1417) -> (0:w1413:bool)
                  n712 = Not Or(1:w1414, 2:w1415) -> (0:w1411:bool)
                  n713 = Select(t=0.0, s=w1412, f=w1431) -> (s? t:f=w1430:dbl)
                  n714 = call <vilib>:"WPI_MotorControlRefNum Registry Get.vi"("refnum name"="Wrist") -> ("error out"=w1463:errorcluster, "MotorControlDevRef"=w1464:T5)  [unwired: 9 in]
                  n715 = call <vilib>:"WPI_SolenoidRefNum Registry Get.vi"("refnum name"="SOL A") -> ("error out"=w1472:errorcluster, "SolenoidDevRef"=w1473:T10)  [unwired: 9 in]
                  n716 = call <vilib>:"WPI_SolenoidRefNum Registry Get.vi"("refnum name"="SOL B") -> ("error out"=w1469:errorcluster, "SolenoidDevRef"=w1470:T10)  [unwired: 9 in]
                  n717 = call <vilib>:"WPI_MotorControlRefNum Registry Get.vi"("refnum name"="Intake") -> ("error out"=w1465:errorcluster, "MotorControlDevRef"=w1466:T5)  [unwired: 9 in]
                  n718 = call <vilib>:"WPI_MotorControlRefNum Registry Get.vi"("refnum name"="Lift") -> ("error out"=w1467:errorcluster, "MotorControlDevRef"=w1468:T5)  [unwired: 9 in]
                  n719 = call <vilib>:"WPI_MotorControlSetOutput.vi"("error in (no error)"=w1463, "Output"=w1424, "MotorControlDevRef"=w1464) -> ()  [unwired: 6 in, 3 out]
                  n720 = call-poly <vilib>:"WPI_SolenoidSet.vi"("error in (no error)"=w1472, "Value"=w1459, "SolenoidDevRef"=w1473) -> ()  [unwired: 7 in, 2 out]
                  n721 = call-poly <vilib>:"WPI_SolenoidSet.vi"("error in (no error)"=w1469, "Value"=w1458, "SolenoidDevRef"=w1470) -> ()  [unwired: 7 in, 2 out]
                  n722 = Or(x=w1413, y=w1412) -> (x .or. y?=w1409:bool)
                  n723 = Or(x=w1411, y=w1410) -> (x .or. y?=w1408:bool)
                  n724 = call <vilib>:"WPI_MotorControlSetOutput.vi"("error in (no error)"=w1465, "Output"=w1440, "MotorControlDevRef"=w1466) -> ()  [unwired: 6 in, 3 out]
                  n725 = call <vilib>:"WPI_MotorControlSetOutput.vi"("error in (no error)"=w1467, "Output"=w1430, "MotorControlDevRef"=w1468) -> ()  [unwired: 6 in, 3 out]
                  n726 = And(x=w1409, y=w1408) -> (x .and. y?=w1407:bool)
                  n727 = Select(t=0.0, s=w1406, f=w1435) -> (s? t:f=w1418:dbl)
                  n728 = Select(t=0.0, s=w1405, f=w1434) -> (s? t:f=w1419:dbl)
                  n729 = call <vilib>:"WPI_RobotDriveTankDrive.vi"("Right axis value"=w1418, "Left axis value"=w1419, "RobotDriveDevRef"=w1476) -> ("error out"=w1452:errorcluster, "Motor Values"=w1437:dbl[], "RobotDriveDevRef"=w1477:T4)  [unwired: 6 in]
                  n730 = global write "Robot Global Data.vi" "Wrist Reset"(w1420) -> ()
                  n731 = global write "Robot Global Data.vi" "Left Reset"(w1420) -> ()
                  n732 = global write "Robot Global Data.vi" "Right Reset"(w1420) -> ()
                  n733 = global write "Robot Global Data.vi" "Lift Reset"(w1420) -> ()
                  n734 = And(x=w1405, y=w1406) -> (x .and. y?=w1422:bool)
                  n735 = And(x=w1407, y=w1422) -> (x .and. y?=w1421:bool)
                  n736 = call-poly <vilib>:"NT Write Value.vi"("Numeric Array"=w1437, "Name"="RobotDrive Motors") -> ()  [unwired: 9 in, 1 out]
                  n737 = Select(t=0.0, s=w1421, f=w1453) -> (s? t:f=w1436:dbl)
                }
                frame False {
                  w1478 = TRUE ("Left Reset")
                  n738 = Select(t=-1.0, s=w1486, f=0.0) -> (s? t:f=w1485:dbl)
                  n739 = global write "Robot Global Data.vi" "Wrist Reset"(w1478) -> ()
                  n740 = global write "Robot Global Data.vi" "Left Reset"(w1478) -> ()
                  n741 = global write "Robot Global Data.vi" "Right Reset"(w1478) -> ()
                  n742 = global write "Robot Global Data.vi" "Lift Reset"(w1478) -> ()
                  n743 = call <vilib>:"WPI_RobotDriveTankDrive.vi"("Right axis value"=0.0, "Left axis value"=0.0, "RobotDriveDevRef"=w1496) -> ("error out"=w1494:errorcluster, "Motor Values"=w1499:dbl[], "RobotDriveDevRef"=w1495:T4)  [unwired: 6 in]
                  n744 = Wait (ms)(milliseconds to wait=w1484) -> ()  [unwired: 1 out]
                  n745 = call <vilib>:"WPI_MotorControlRefNum Registry Get.vi"("refnum name"="Intake") -> ("error out"=w1490:errorcluster, "MotorControlDevRef"=w1491:T5)  [unwired: 9 in]
                  n746 = call-poly <vilib>:"NT Write Value.vi"("Numeric Array"=w1499, "Name"="RobotDrive Motors") -> ()  [unwired: 9 in, 1 out]
                  n747 = global read "Robot Global Data.vi" "Wrist Reset"() -> (w1482:bool)
                  n748 = global read "Robot Global Data.vi" "Right Reset"() -> (w1492:bool)
                  n749 = global read "Robot Global Data.vi" "Lift Reset"() -> (w1483:bool)
                  n750 = global read "Robot Global Data.vi" "Left Reset"() -> (w1493:bool)
                  n751 = call <vilib>:"WPI_MotorControlSetOutput.vi"("error in (no error)"=w1490, "Output"=w1485, "MotorControlDevRef"=w1491) -> ()  [unwired: 6 in, 3 out]
                  n752 = And(x=w1493, y=w1492) -> (x .and. y?=w1480:bool)
                  n753 = And(x=w1483, y=w1482) -> (x .and. y?=w1481:bool)
                  n754 = And(x=w1480, y=w1481) -> (x .and. y?=w1479:bool)
                }
              }
            }
            n755 = call <vilib>:"WPI_RobotDriveDelayAndUpdateSafety.vi"("error in (no error)"=w1371, "Delay (s)"=w1373, "RobotDriveDevRef"=w1372) -> ("RobotDriveDevRef 2"=w1376:T4)  [unwired: 7 in, 1 out]
          }
        }
        frame "RLR" {
          n756 = Array Size(array="Right RLR") -> (size(s)=w1502:i32)
          n757 = call <vilib>:"WPI_RobotDriveRefNum Registry Get.vi"("refnum name"="Left and Right Motors") -> ("RobotDriveDevRef"=w1503:T4)  [unwired: 1 in, 9 out]
          n758 = for {
            N: w1502 -> [_]
            shift-right: [w1511] -> _
            shift-left: w1503 -> [w1510]
            tunnel: "Right RLR" -> [w1509] mode=indexing
            i -> [w1505]
            n759 = global write "Robot Global Data.vi" "Array Step"(w1505) -> ()
            n760 = while {
              shift-right: [w1539] -> w1507
              shift-left: w1510 -> [w1538]
              tunnel: w1509 -> [w1535]
              tunnel: [w1516] -> w1508
              tunnel: [w1519] -> w1506
              stop <- w1520 stop-if-true
              n761 = global read "Robot Global Data.vi" "Right Distance"() -> (w1523:dbl)
              n762 = global read "Robot Global Data.vi" "Lift Distance"() -> (w1514:dbl)
              n763 = global read "Robot Global Data.vi" "Left Distance"() -> (w1522:dbl)
              n764 = Unbundle By Name(w1535) -> ("Left Joystick"=w1534:dbl, "Right Joystick"=w1533:dbl, "Duration"=w1521:dbl, "SOL A"=w1532:bool, "SOL B"=w1531:bool, "Lift Up"=w1530:bool, "Lift Down"=w1529:bool, "Intake In"=w1528:bool, "Intake Out"=w1527:bool, "Wrist Up"=w1526:bool, "Wrist Down"=w1525:bool, "Left Distance"=w1515:dbl, "Right Distance"=w1524:dbl, "Drive?"=w1518:bool, "Lift Target"=w1513:dbl, "Wrist Target"=w1512:dbl)
              n765 = global read "Robot Global Data.vi" "Wrist Angle"() -> (w1517:dbl)
              n766 = global read "Robot Global Data.vi" "Left Rate"() -> (w1537:dbl)
              n767 = global read "Robot Global Data.vi" "Right Rate"() -> (w1536:dbl)
              n768 = case shown="True" w1518 {
                tunnel: [w1612 w1630] -> w1539
                tunnel: w1538 -> [w1611 w1631]
                tunnel: w1537 -> [_ _]
                tunnel: w1536 -> [_ _]
                tunnel: w1534 -> [w1569 _]
                tunnel: w1533 -> [w1570 _]
                tunnel: w1532 -> [w1594 _]
                tunnel: w1531 -> [w1593 _]
                tunnel: w1530 -> [w1552 _]
                tunnel: w1529 -> [w1551 _]
                tunnel: w1528 -> [w1574 _]
                tunnel: w1527 -> [_ w1621]
                tunnel: w1526 -> [w1550 _]
                tunnel: w1525 -> [w1549 _]
                tunnel: w1515 -> [w1573 _]
                tunnel: w1524 -> [w1592 _]
                tunnel: w1523 -> [w1591 _]
                tunnel: w1522 -> [w1590 _]
                tunnel: w1521 -> [w1588 w1619]
                tunnel: [w1571 w1619] -> w1516
                tunnel: [w1556 w1614] -> w1520
                tunnel: [w1587 w1629] -> w1519
                tunnel: w1517 -> [w1563 _]
                tunnel: w1514 -> [w1564 _]
                tunnel: w1513 -> [w1568 _]
                tunnel: w1512 -> [w1562 _]
                frame True {
                  w1555 = FALSE ("Left Reset")
                  n769 = Greater Or Equal?(x=w1563, y=w1562) -> (x >= y?=w1545:bool)
                  n770 = Select(t=-1.0, s=w1549, f=0.1) -> (s? t:f=w1577:dbl)
                  n771 = Greater Or Equal?(x=w1564, y=w1568) -> (x >= y?=w1547:bool)
                  n772 = Greater Or Equal?(x=w1590, y=w1573) -> (x >= y?=w1540:bool)
                  n773 = Greater Or Equal?(x=w1591, y=w1592) -> (x >= y?=w1541:bool)
                  n774 = Select(t=1.0, s=w1550, f=w1577) -> (s? t:f=w1560:dbl)
                  n775 = Select(t=-1.0, s=w1551, f=0.1) -> (s? t:f=w1576:dbl)
                  n776 = Select(t=1.0, s=w1552, f=w1576) -> (s? t:f=w1566:dbl)
                  n777 = Select(t=0.0, s=w1545, f=w1560) -> (s? t:f=w1559:dbl)
                  n778 = Select(t=1.0, s=w1574, f=0.0) -> (s? t:f=w1575:dbl)
                  n779 = Not Or(1:w1551, 2:w1552) -> (0:w1548:bool)
                  n780 = Not Or(1:w1549, 2:w1550) -> (0:w1546:bool)
                  n781 = Select(t=0.0, s=w1547, f=w1566) -> (s? t:f=w1565:dbl)
                  n782 = call <vilib>:"WPI_MotorControlRefNum Registry Get.vi"("refnum name"="Wrist") -> ("error out"=w1598:errorcluster, "MotorControlDevRef"=w1599:T5)  [unwired: 9 in]
                  n783 = call <vilib>:"WPI_SolenoidRefNum Registry Get.vi"("refnum name"="SOL A") -> ("error out"=w1607:errorcluster, "SolenoidDevRef"=w1608:T10)  [unwired: 9 in]
                  n784 = call <vilib>:"WPI_SolenoidRefNum Registry Get.vi"("refnum name"="SOL B") -> ("error out"=w1604:errorcluster, "SolenoidDevRef"=w1605:T10)  [unwired: 9 in]
                  n785 = call <vilib>:"WPI_MotorControlRefNum Registry Get.vi"("refnum name"="Intake") -> ("error out"=w1600:errorcluster, "MotorControlDevRef"=w1601:T5)  [unwired: 9 in]
                  n786 = call <vilib>:"WPI_MotorControlRefNum Registry Get.vi"("refnum name"="Lift") -> ("error out"=w1602:errorcluster, "MotorControlDevRef"=w1603:T5)  [unwired: 9 in]
                  n787 = call <vilib>:"WPI_MotorControlSetOutput.vi"("error in (no error)"=w1598, "Output"=w1559, "MotorControlDevRef"=w1599) -> ()  [unwired: 6 in, 3 out]
                  n788 = call-poly <vilib>:"WPI_SolenoidSet.vi"("error in (no error)"=w1607, "Value"=w1594, "SolenoidDevRef"=w1608) -> ()  [unwired: 7 in, 2 out]
                  n789 = call-poly <vilib>:"WPI_SolenoidSet.vi"("error in (no error)"=w1604, "Value"=w1593, "SolenoidDevRef"=w1605) -> ()  [unwired: 7 in, 2 out]
                  n790 = Or(x=w1548, y=w1547) -> (x .or. y?=w1544:bool)
                  n791 = Or(x=w1546, y=w1545) -> (x .or. y?=w1543:bool)
                  n792 = call <vilib>:"WPI_MotorControlSetOutput.vi"("error in (no error)"=w1600, "Output"=w1575, "MotorControlDevRef"=w1601) -> ()  [unwired: 6 in, 3 out]
                  n793 = call <vilib>:"WPI_MotorControlSetOutput.vi"("error in (no error)"=w1602, "Output"=w1565, "MotorControlDevRef"=w1603) -> ()  [unwired: 6 in, 3 out]
                  n794 = And(x=w1544, y=w1543) -> (x .and. y?=w1542:bool)
                  n795 = Select(t=0.0, s=w1541, f=w1570) -> (s? t:f=w1553:dbl)
                  n796 = Select(t=0.0, s=w1540, f=w1569) -> (s? t:f=w1554:dbl)
                  n797 = call <vilib>:"WPI_RobotDriveTankDrive.vi"("Right axis value"=w1553, "Left axis value"=w1554, "RobotDriveDevRef"=w1611) -> ("error out"=w1587:errorcluster, "Motor Values"=w1572:dbl[], "RobotDriveDevRef"=w1612:T4)  [unwired: 6 in]
                  n798 = global write "Robot Global Data.vi" "Wrist Reset"(w1555) -> ()
                  n799 = global write "Robot Global Data.vi" "Left Reset"(w1555) -> ()
                  n800 = global write "Robot Global Data.vi" "Right Reset"(w1555) -> ()
                  n801 = global write "Robot Global Data.vi" "Lift Reset"(w1555) -> ()
                  n802 = And(x=w1540, y=w1541) -> (x .and. y?=w1557:bool)
                  n803 = And(x=w1542, y=w1557) -> (x .and. y?=w1556:bool)
                  n804 = call-poly <vilib>:"NT Write Value.vi"("Numeric Array"=w1572, "Name"="RobotDrive Motors") -> ()  [unwired: 9 in, 1 out]
                  n805 = Select(t=0.0, s=w1556, f=w1588) -> (s? t:f=w1571:dbl)
                }
                frame False {
                  w1613 = TRUE ("Left Reset")
                  n806 = Select(t=-1.0, s=w1621, f=0.0) -> (s? t:f=w1620:dbl)
                  n807 = global write "Robot Global Data.vi" "Wrist Reset"(w1613) -> ()
                  n808 = global write "Robot Global Data.vi" "Left Reset"(w1613) -> ()
                  n809 = global write "Robot Global Data.vi" "Right Reset"(w1613) -> ()
                  n810 = global write "Robot Global Data.vi" "Lift Reset"(w1613) -> ()
                  n811 = call <vilib>:"WPI_RobotDriveTankDrive.vi"("Right axis value"=0.0, "Left axis value"=0.0, "RobotDriveDevRef"=w1631) -> ("error out"=w1629:errorcluster, "Motor Values"=w1634:dbl[], "RobotDriveDevRef"=w1630:T4)  [unwired: 6 in]
                  n812 = Wait (ms)(milliseconds to wait=w1619) -> ()  [unwired: 1 out]
                  n813 = call <vilib>:"WPI_MotorControlRefNum Registry Get.vi"("refnum name"="Intake") -> ("error out"=w1625:errorcluster, "MotorControlDevRef"=w1626:T5)  [unwired: 9 in]
                  n814 = call-poly <vilib>:"NT Write Value.vi"("Numeric Array"=w1634, "Name"="RobotDrive Motors") -> ()  [unwired: 9 in, 1 out]
                  n815 = global read "Robot Global Data.vi" "Wrist Reset"() -> (w1617:bool)
                  n816 = global read "Robot Global Data.vi" "Right Reset"() -> (w1627:bool)
                  n817 = global read "Robot Global Data.vi" "Lift Reset"() -> (w1618:bool)
                  n818 = global read "Robot Global Data.vi" "Left Reset"() -> (w1628:bool)
                  n819 = call <vilib>:"WPI_MotorControlSetOutput.vi"("error in (no error)"=w1625, "Output"=w1620, "MotorControlDevRef"=w1626) -> ()  [unwired: 6 in, 3 out]
                  n820 = And(x=w1628, y=w1627) -> (x .and. y?=w1615:bool)
                  n821 = And(x=w1618, y=w1617) -> (x .and. y?=w1616:bool)
                  n822 = And(x=w1615, y=w1616) -> (x .and. y?=w1614:bool)
                }
              }
            }
            n823 = call <vilib>:"WPI_RobotDriveDelayAndUpdateSafety.vi"("error in (no error)"=w1506, "Delay (s)"=w1508, "RobotDriveDevRef"=w1507) -> ("RobotDriveDevRef 2"=w1511:T4)  [unwired: 7 in, 1 out]
          }
        }
        frame "LLL", Default {
          n824 = Array Size(array="Right LLL") -> (size(s)=w1637:i32)
          n825 = call <vilib>:"WPI_RobotDriveRefNum Registry Get.vi"("refnum name"="Left and Right Motors") -> ("RobotDriveDevRef"=w1638:T4)  [unwired: 1 in, 9 out]
          n826 = for {
            N: w1637 -> [_]
            shift-right: [w1646] -> _
            shift-left: w1638 -> [w1645]
            tunnel: "Right LLL" -> [w1644] mode=indexing
            i -> [w1640]
            n827 = global write "Robot Global Data.vi" "Array Step"(w1640) -> ()
            n828 = while {
              shift-right: [w1674] -> w1642
              shift-left: w1645 -> [w1673]
              tunnel: w1644 -> [w1670]
              tunnel: [w1651] -> w1643
              tunnel: [w1654] -> w1641
              stop <- w1655 stop-if-true
              n829 = global read "Robot Global Data.vi" "Right Distance"() -> (w1658:dbl)
              n830 = global read "Robot Global Data.vi" "Lift Distance"() -> (w1649:dbl)
              n831 = global read "Robot Global Data.vi" "Left Distance"() -> (w1657:dbl)
              n832 = Unbundle By Name(w1670) -> ("Left Joystick"=w1669:dbl, "Right Joystick"=w1668:dbl, "Duration"=w1656:dbl, "SOL A"=w1667:bool, "SOL B"=w1666:bool, "Lift Up"=w1665:bool, "Lift Down"=w1664:bool, "Intake In"=w1663:bool, "Intake Out"=w1662:bool, "Wrist Up"=w1661:bool, "Wrist Down"=w1660:bool, "Left Distance"=w1650:dbl, "Right Distance"=w1659:dbl, "Drive?"=w1653:bool, "Lift Target"=w1648:dbl, "Wrist Target"=w1647:dbl)
              n833 = global read "Robot Global Data.vi" "Wrist Angle"() -> (w1652:dbl)
              n834 = global read "Robot Global Data.vi" "Left Rate"() -> (w1672:dbl)
              n835 = global read "Robot Global Data.vi" "Right Rate"() -> (w1671:dbl)
              n836 = case shown="True" w1653 {
                tunnel: [w1747 w1765] -> w1674
                tunnel: w1673 -> [w1746 w1766]
                tunnel: w1672 -> [_ _]
                tunnel: w1671 -> [_ _]
                tunnel: w1669 -> [w1704 _]
                tunnel: w1668 -> [w1705 _]
                tunnel: w1667 -> [w1729 _]
                tunnel: w1666 -> [w1728 _]
                tunnel: w1665 -> [w1687 _]
                tunnel: w1664 -> [w1686 _]
                tunnel: w1663 -> [w1709 _]
                tunnel: w1662 -> [_ w1756]
                tunnel: w1661 -> [w1685 _]
                tunnel: w1660 -> [w1684 _]
                tunnel: w1650 -> [w1708 _]
                tunnel: w1659 -> [w1727 _]
                tunnel: w1658 -> [w1726 _]
                tunnel: w1657 -> [w1725 _]
                tunnel: w1656 -> [w1723 w1754]
                tunnel: [w1706 w1754] -> w1651
                tunnel: [w1691 w1749] -> w1655
                tunnel: [w1722 w1764] -> w1654
                tunnel: w1652 -> [w1698 _]
                tunnel: w1649 -> [w1699 _]
                tunnel: w1648 -> [w1703 _]
                tunnel: w1647 -> [w1697 _]
                frame True {
                  w1690 = FALSE ("Left Reset")
                  n837 = Greater Or Equal?(x=w1698, y=w1697) -> (x >= y?=w1680:bool)
                  n838 = Select(t=-1.0, s=w1684, f=0.1) -> (s? t:f=w1712:dbl)
                  n839 = Greater Or Equal?(x=w1699, y=w1703) -> (x >= y?=w1682:bool)
                  n840 = Greater Or Equal?(x=w1725, y=w1708) -> (x >= y?=w1675:bool)
                  n841 = Greater Or Equal?(x=w1726, y=w1727) -> (x >= y?=w1676:bool)
                  n842 = Select(t=1.0, s=w1685, f=w1712) -> (s? t:f=w1695:dbl)
                  n843 = Select(t=-1.0, s=w1686, f=0.1) -> (s? t:f=w1711:dbl)
                  n844 = Select(t=1.0, s=w1687, f=w1711) -> (s? t:f=w1701:dbl)
                  n845 = Select(t=0.0, s=w1680, f=w1695) -> (s? t:f=w1694:dbl)
                  n846 = Select(t=1.0, s=w1709, f=0.0) -> (s? t:f=w1710:dbl)
                  n847 = Not Or(1:w1686, 2:w1687) -> (0:w1683:bool)
                  n848 = Not Or(1:w1684, 2:w1685) -> (0:w1681:bool)
                  n849 = Select(t=0.0, s=w1682, f=w1701) -> (s? t:f=w1700:dbl)
                  n850 = call <vilib>:"WPI_MotorControlRefNum Registry Get.vi"("refnum name"="Wrist") -> ("error out"=w1733:errorcluster, "MotorControlDevRef"=w1734:T5)  [unwired: 9 in]
                  n851 = call <vilib>:"WPI_SolenoidRefNum Registry Get.vi"("refnum name"="SOL A") -> ("error out"=w1742:errorcluster, "SolenoidDevRef"=w1743:T10)  [unwired: 9 in]
                  n852 = call <vilib>:"WPI_SolenoidRefNum Registry Get.vi"("refnum name"="SOL B") -> ("error out"=w1739:errorcluster, "SolenoidDevRef"=w1740:T10)  [unwired: 9 in]
                  n853 = call <vilib>:"WPI_MotorControlRefNum Registry Get.vi"("refnum name"="Intake") -> ("error out"=w1735:errorcluster, "MotorControlDevRef"=w1736:T5)  [unwired: 9 in]
                  n854 = call <vilib>:"WPI_MotorControlRefNum Registry Get.vi"("refnum name"="Lift") -> ("error out"=w1737:errorcluster, "MotorControlDevRef"=w1738:T5)  [unwired: 9 in]
                  n855 = call <vilib>:"WPI_MotorControlSetOutput.vi"("error in (no error)"=w1733, "Output"=w1694, "MotorControlDevRef"=w1734) -> ()  [unwired: 6 in, 3 out]
                  n856 = call-poly <vilib>:"WPI_SolenoidSet.vi"("error in (no error)"=w1742, "Value"=w1729, "SolenoidDevRef"=w1743) -> ()  [unwired: 7 in, 2 out]
                  n857 = call-poly <vilib>:"WPI_SolenoidSet.vi"("error in (no error)"=w1739, "Value"=w1728, "SolenoidDevRef"=w1740) -> ()  [unwired: 7 in, 2 out]
                  n858 = Or(x=w1683, y=w1682) -> (x .or. y?=w1679:bool)
                  n859 = Or(x=w1681, y=w1680) -> (x .or. y?=w1678:bool)
                  n860 = call <vilib>:"WPI_MotorControlSetOutput.vi"("error in (no error)"=w1735, "Output"=w1710, "MotorControlDevRef"=w1736) -> ()  [unwired: 6 in, 3 out]
                  n861 = call <vilib>:"WPI_MotorControlSetOutput.vi"("error in (no error)"=w1737, "Output"=w1700, "MotorControlDevRef"=w1738) -> ()  [unwired: 6 in, 3 out]
                  n862 = And(x=w1679, y=w1678) -> (x .and. y?=w1677:bool)
                  n863 = Select(t=0.0, s=w1676, f=w1705) -> (s? t:f=w1688:dbl)
                  n864 = Select(t=0.0, s=w1675, f=w1704) -> (s? t:f=w1689:dbl)
                  n865 = call <vilib>:"WPI_RobotDriveTankDrive.vi"("Right axis value"=w1688, "Left axis value"=w1689, "RobotDriveDevRef"=w1746) -> ("error out"=w1722:errorcluster, "Motor Values"=w1707:dbl[], "RobotDriveDevRef"=w1747:T4)  [unwired: 6 in]
                  n866 = global write "Robot Global Data.vi" "Wrist Reset"(w1690) -> ()
                  n867 = global write "Robot Global Data.vi" "Left Reset"(w1690) -> ()
                  n868 = global write "Robot Global Data.vi" "Right Reset"(w1690) -> ()
                  n869 = global write "Robot Global Data.vi" "Lift Reset"(w1690) -> ()
                  n870 = And(x=w1675, y=w1676) -> (x .and. y?=w1692:bool)
                  n871 = And(x=w1677, y=w1692) -> (x .and. y?=w1691:bool)
                  n872 = call-poly <vilib>:"NT Write Value.vi"("Numeric Array"=w1707, "Name"="RobotDrive Motors") -> ()  [unwired: 9 in, 1 out]
                  n873 = Select(t=0.0, s=w1691, f=w1723) -> (s? t:f=w1706:dbl)
                }
                frame False {
                  w1748 = TRUE ("Left Reset")
                  n874 = Select(t=-1.0, s=w1756, f=0.0) -> (s? t:f=w1755:dbl)
                  n875 = global write "Robot Global Data.vi" "Wrist Reset"(w1748) -> ()
                  n876 = global write "Robot Global Data.vi" "Left Reset"(w1748) -> ()
                  n877 = global write "Robot Global Data.vi" "Right Reset"(w1748) -> ()
                  n878 = global write "Robot Global Data.vi" "Lift Reset"(w1748) -> ()
                  n879 = call <vilib>:"WPI_RobotDriveTankDrive.vi"("Right axis value"=0.0, "Left axis value"=0.0, "RobotDriveDevRef"=w1766) -> ("error out"=w1764:errorcluster, "Motor Values"=w1769:dbl[], "RobotDriveDevRef"=w1765:T4)  [unwired: 6 in]
                  n880 = Wait (ms)(milliseconds to wait=w1754) -> ()  [unwired: 1 out]
                  n881 = call <vilib>:"WPI_MotorControlRefNum Registry Get.vi"("refnum name"="Intake") -> ("error out"=w1760:errorcluster, "MotorControlDevRef"=w1761:T5)  [unwired: 9 in]
                  n882 = call-poly <vilib>:"NT Write Value.vi"("Numeric Array"=w1769, "Name"="RobotDrive Motors") -> ()  [unwired: 9 in, 1 out]
                  n883 = global read "Robot Global Data.vi" "Wrist Reset"() -> (w1752:bool)
                  n884 = global read "Robot Global Data.vi" "Right Reset"() -> (w1762:bool)
                  n885 = global read "Robot Global Data.vi" "Lift Reset"() -> (w1753:bool)
                  n886 = global read "Robot Global Data.vi" "Left Reset"() -> (w1763:bool)
                  n887 = call <vilib>:"WPI_MotorControlSetOutput.vi"("error in (no error)"=w1760, "Output"=w1755, "MotorControlDevRef"=w1761) -> ()  [unwired: 6 in, 3 out]
                  n888 = And(x=w1763, y=w1762) -> (x .and. y?=w1750:bool)
                  n889 = And(x=w1753, y=w1752) -> (x .and. y?=w1751:bool)
                  n890 = And(x=w1750, y=w1751) -> (x .and. y?=w1749:bool)
                }
              }
            }
            n891 = call <vilib>:"WPI_RobotDriveDelayAndUpdateSafety.vi"("error in (no error)"=w1641, "Delay (s)"=w1643, "RobotDriveDevRef"=w1642) -> ("RobotDriveDevRef 2"=w1646:T4)  [unwired: 7 in, 1 out]
          }
        }
      }
    }
  }
